vi "BAES RI Retrieval with LABVIEW.vi"() -> ()   [LabVIEW 2013]
uses:
  BaesDataTypeDefinition.ctl
  ReadBaesDataTypeDefinition.ctl
  ParticleDistributionData.ctl
  GeneralDataForRIRetrieval.ctl
  <vilib>/Native 3D Graph/xcontrol/3DPC_SurfacePlot.xctl
  <vilib>/Native 3D Graph/classes/Surface/Surface.lvclass
  RIandRIMCResults.ctl
  <vilib>/gmath/NumericalOptimization/stopping criteria.ctl
  <vilib>/Analysis/1siggen.llb/Ramp Pattern by Samples.vi
  <vilib>/gmath/NumericalOptimization/Conjugate Gradient.vi
  <vilib>/Utility/file.llb/Write To Spreadsheet File (string).vi
  <vilib>/Analysis/Matrix/Numeric/Conversions/Matrix To Array - RM.vi
  <vilib>/gmath/statdist.llb/Normal Inverse CDF.vi
  <vilib>/imath/engines/lvmath2/RunTimeEngine/ErrorHandling/NIMS_Finalize Error.vi
  <vilib>/imath/engines/lvmath2/RunTimeEngine/RangeToken/NIMS_Range_R2 - Float.vi
  <instcachedir>/0/NIMS_Range_R2 - Float_E19924E36A3948A4B33043226480F83C.lvgen/NIMS_Range_R2 - Float_E19924E36A3948A4B33043226480F83C_000.vi
  <vilib>/imath/engines/lvmath2/RunTimeEngine/NodeEndStatement/NIMS_NodeEndStatement_Output.vi
  <instcachedir>/0/NIMS_NodeEndStatement_Output_53EC0D466D134D7ABD903AC30B43404B.lvgen/NIMS_NodeEndStatement_Output_53EC0D466D134D7ABD903AC30B43404B_002.vi
  <vilib>/imath/engines/lvmath2/RunTimeEngine/CommandStatement/MC_CommandStatement_break.vi
  <vilib>/imath/engines/lvmath2/RunTimeSupport/NIMS_Error if Not Equal.vi
  <instcachedir>/0/NIMS_Error if Not Equal_902F5D2649E64F5087A1EF57C55C58AB.lvgen/NIMS_Error if Not Equal_902F5D2649E64F5087A1EF57C55C58AB_000.vi
  <vilib>/imath/engines/lvmath2/RunTimeEngine/IndexRead/NIMS M($,S).vi
  <instcachedir>/0/NIMS M($,S)_3E5749BBB62E49528D4765A77F1F6D98.lvgen/NIMS M($,S)_3E5749BBB62E49528D4765A77F1F6D98_000.vi
  <vilib>/imath/engines/lvmath2/RunTimeEngine/RowToken/NIMS_RowToken_M_CV.vi
  <instcachedir>/0/NIMS_RowToken_M_CV_4FFFB80A1A2C4A06BEF1E2564C6BAFA4.lvgen/NIMS_RowToken_M_CV_4FFFB80A1A2C4A06BEF1E2564C6BAFA4_000.vi
  <vilib>/imath/engines/lvmath2/RunTimeEngine/ErrorHandling/NIMS_Create Error From Enums.vi
  <vilib>/gmath/NI_Gmath.lvlib
  <vilib>/Analysis/Matrix/NI_Matrix.lvlib
  <vilib>/Analysis/NI_AALBase.lvlib
panel:
  out "Size Distribution":T1(graph)=[{"Ramp Pattern"=[105.5, 109.4, 113.4, 117.6, 121.9, 126.3, 131.0, 135.8, 140.7, 145.9, 151.2, 156.8, 162.5, 168.5, 174.7, 181.1, 187.7, 194.6, 201.7, 209.1, 216.7, 224.7, 232.9, 241.4, 250.3, 259.5, 269.0, 278.8, 289.0, 299.6, 310.6, 322.0, 333.8, 346.0, 358.7, 371.8, 385.4, 399.5, 414.2, 429.4, 445.1, 461.4, 478.3, 495.8, 514.0, 532.8, 552.3, 572.5, 593.5, 615.3, 637.8, 661.2, 685.4, 710.5, 736.5, 763.5, 791.5], "Extinction"=[0.0, 0.0, 0.0, 0.0, 0.0, 0.0, 0.00366116, 0.0296415, 0.103002, 0.199671, 0.237311, 0.178682, 0.0821533, 0.0212338, 0.00234049, 0.0, 0.0, 0.0, 0.000322909, 0.00289299, 0.0111396, 0.0241563, 0.0327108, 0.029032, 0.0169297, 0.00614836, 0.00137168, 0.000708524, 0.00196524, 0.0037587, 0.00463248, 0.00371899, 0.00198243, 0.000683679, 0.00013815, 1.21e-05, 0.0, 0.0, 0.0, 0.0, 0.0, 0.0, 0.0, 0.0, 0.0, 0.0, 0.0, 0.0, 0.0, 0.0, 0.0, 0.0, 0.0, 0.0, 0.0, 0.0, 0.0]}, {"Ramp Pattern"=[105.5, 109.4, 113.4, 117.6, 121.9, 126.3, 131.0, 135.8, 140.7, 145.9, 151.2, 156.8, 162.5, 168.5, 174.7, 181.1, 187.7, 194.6, 201.7, 209.1, 216.7, 224.7, 232.9, 241.4, 250.3, 259.5, 269.0, 278.8, 289.0, 299.6, 310.6, 322.0, 333.8, 346.0, 358.7, 371.8, 385.4, 399.5, 414.2, 429.4, 445.1, 461.4, 478.3, 495.8, 514.0, 532.8, 552.3, 572.5, 593.5, 615.3, 637.8, 661.2, 685.4, 710.5, 736.5, 763.5, 791.5], "Extinction"=[0.0, 0.0, 0.0, 0.0, 0.0, 0.0, 0.0, 0.0, 0.0, 0.0, 0.0, 0.0, 0.0, 0.0, 0.00492, 0.0371074, 0.121809, 0.224941, 0.255025, 0.181972, 0.0807483, 0.0201359, 0.00215921, 0.0, 0.0, 0.0, 0.0, 0.000345586, 0.00252918, 0.00805624, 0.0149912, 0.0175018, 0.0135532, 0.00703785, 0.00236058, 0.000456625, 0.000114849, 0.000344556, 0.000807346, 0.00117242, 0.0010019, 0.000622724, 0.000225813, 5.24e-05, 7.42e-06, 4.28e-07, 0.0, 0.0, 0.0, 0.0, 0.0, 0.0, 0.0, 0.0, 0.0, 0.0, 0.0]}, {"Ramp Pattern"=[105.5, 109.4, 113.4, 117.6, 121.9, 126.3, 131.0, 135.8, 140.7, 145.9, 151.2, 156.8, 162.5, 168.5, 174.7, 181.1, 187.7, 194.6, 201.7, 209.1, 216.7, 224.7, 232.9, 241.4, 250.3, 259.5, 269.0, 278.8, 289.0, 299.6, 310.6, 322.0, 333.8, 346.0, 358.7, 371.8, 385.4, 399.5, 414.2, 429.4, 445.1, 461.4, 478.3, 495.8, 514.0, 532.8, 552.3, 572.5, 593.5, 615.3, 637.8, 661.2, 685.4, 710.5, 736.5, 763.5, 791.5], "Extinction"=[0.0, 0.0, 0.0, 0.0, 0.0, 0.0, 0.0, 0.0, 0.0, 0.0, 0.0, 0.0, 0.0, 0.0, 0.0, 0.0, 0.0, 0.0, 0.0, 0.0, 0.00609686, 0.0438534, 0.136127, 0.240173, 0.263478, 0.180795, 0.0780342, 0.019699, 0.00232773, 5.83e-05, 0.0, 0.0, 0.0, 0.0, 0.000288595, 0.00176402, 0.00479166, 0.00737608, 0.00718805, 0.004762, 0.00191333, 0.000545424, 8.17e-05, 1.76e-05, 5.87e-05, 0.000120519, 0.000171987, 0.000138883, 9.46e-05, 3.36e-05, 9.69e-06, 1.71e-06, 1.17e-07, 0.0, 0.0, 0.0, 0.0]}, {"Ramp Pattern"=[105.5, 109.4, 113.4, 117.6, 121.9, 126.3, 131.0, 135.8, 140.7, 145.9, 151.2, 156.8, 162.5, 168.5, 174.7, 181.1, 187.7, 194.6, 201.7, 209.1, 216.7, 224.7, 232.9, 241.4, 250.3, 259.5, 269.0, 278.8, 289.0, 299.6, 310.6, 322.0, 333.8, 346.0, 358.7, 371.8, 385.4, 399.5, 414.2, 429.4, 445.1, 461.4, 478.3, 495.8, 514.0, 532.8, 552.3, 572.5, 593.5, 615.3, 637.8, 661.2, 685.4, 710.5, 736.5, 763.5, 791.5], "Extinction"=[0.0, 0.0, 0.0, 0.0, 0.0, 0.0, 0.0, 0.0, 0.0, 0.0, 0.0, 0.0, 0.0, 0.0, 0.0, 0.0, 0.0, 0.0, 0.0, 0.0, 0.0, 0.0, 0.0, 0.0, 0.0, 0.00736806, 0.0500661, 0.148338, 0.249147, 0.261489, 0.176277, 0.0750088, 0.0194137, 0.00265533, 0.000136312, 0.0, 0.0, 0.0, 0.0, 7.49e-05, 0.000496319, 0.00144105, 0.00238802, 0.00252961, 0.00178475, 0.000847522, 0.000261538, 5.8e-05, 6.72e-06, 5.33e-06, 1.09e-05, 2.51e-05, 4.82e-05, 4.62e-05, 3.31e-05, 2.71e-05, 1.62e-05]}, {"Ramp Pattern"=[105.5, 109.4, 113.4, 117.6, 121.9, 126.3, 131.0, 135.8, 140.7, 145.9, 151.2, 156.8, 162.5, 168.5, 174.7, 181.1, 187.7, 194.6, 201.7, 209.1, 216.7, 224.7, 232.9, 241.4, 250.3, 259.5, 269.0, 278.8, 289.0, 299.6, 310.6, 322.0, 333.8, 346.0, 358.7, 371.8, 385.4, 399.5, 414.2, 429.4, 445.1, 461.4, 478.3, 495.8, 514.0, 532.8, 552.3, 572.5, 593.5, 615.3, 637.8, 661.2, 685.4, 710.5, 736.5, 763.5, 791.5], "Extinction"=[0.0, 0.0, 0.0, 0.0, 0.0, 0.0, 0.0, 0.0, 0.0, 0.0, 0.0, 0.0, 0.0, 0.0, 0.0, 0.0, 0.0, 0.0, 0.0, 0.0, 0.0, 0.0, 0.0, 0.0, 0.0, 0.0, 0.0, 0.0, 0.0, 0.00859775, 0.0562809, 0.158878, 0.25715, 0.258686, 0.166916, 0.0697154, 0.0177192, 0.00255357, 0.000156501, 0.0, 0.0, 0.0, 0.0, 0.0, 5.58e-05, 0.000279561, 0.000610125, 0.000902507, 0.000776539, 0.000511588, 0.000129793, 4.12e-05, 1.04e-05, 1.65e-06, 3.63e-06, 1.15e-05, 1.27e-05]}, {"Ramp Pattern"=[105.5, 109.4, 113.4, 117.6, 121.9, 126.3, 131.0, 135.8, 140.7, 145.9, 151.2, 156.8, 162.5, 168.5, 174.7, 181.1, 187.7, 194.6, 201.7, 209.1, 216.7, 224.7, 232.9, 241.4, 250.3, 259.5, 269.0, 278.8, 289.0, 299.6, 310.6, 322.0, 333.8, 346.0, 358.7, 371.8, 385.4, 399.5, 414.2, 429.4, 445.1, 461.4, 478.3, 495.8, 514.0, 532.8, 552.3, 572.5, 593.5, 615.3, 637.8, 661.2, 685.4, 710.5, 736.5, 763.5, 791.5], "Extinction"=[0.0, 0.0, 0.0, 0.0, 0.0, 0.0, 0.0, 0.0, 0.0, 0.0, 0.0, 0.0, 0.0, 0.0, 0.0, 0.0, 0.0, 0.0, 0.0, 0.0, 0.0, 0.0, 0.0, 0.0, 0.0, 0.0, 0.0, 0.0, 0.0, 0.0, 0.0, 0.0, 0.000337342, 0.0120252, 0.0672961, 0.175789, 0.261716, 0.2491, 0.154041, 0.0606694, 0.0148893, 0.00206533, 0.00012431, 0.0, 0.0, 0.0, 0.0, 0.0, 1.8e-05, 0.000111181, 0.000176009, 0.000314306, 0.00048843, 0.000387935, 0.000231014, 0.000148961, 7.12e-05]}]
  out "Extinction Data per size":T1(graph)=[{"Ramp Pattern"=[350.32001, 350.89999, 351.48999, 352.07001, 352.64001, 353.22, 353.79999, 354.37, 354.94, 355.51001, 356.07999, 356.64999, 357.22, 357.78, 358.35001, 358.91, 359.47, 360.03, 360.59, 361.14999, 361.70001, 362.26001, 362.81, 363.35999, 363.91, 364.45999, 365.01001, 365.56, 366.10001, 366.64999, 367.19, 367.73001, 368.26999, 368.81, 369.35001, 369.89001, 370.42001, 370.95999, 371.48999, 372.03, 372.56, 373.09, 373.62, 374.14999, 374.67999, 375.20999, 375.73001, 376.26001, 376.78, 377.31, 377.82999, 378.35001, 378.87, 379.39001, 379.91, 380.42999, 380.95001, 381.47, 381.98001, 382.5, 383.01001, 383.53, 384.04001, 384.54999, 385.07001, 385.57999, 386.09, 386.60001, 387.10999, 387.62, 388.13, 388.63, 389.14001, 389.64999, 390.14999, 390.66, 391.16, 391.67001, 392.17001, 392.67999, 389.64999, 390.14999, 390.66, 391.16, 391.67001, 392.17001, 392.67999, 393.17999, 393.67999, 394.17999, 394.67999, 395.19, 395.69, 396.19, 396.69, 397.19, 397.69, 398.19, 398.69, 399.19, 399.67999, 400.17999, 400.67999, 401.17999, 401.67999, 402.17001, 402.67001, 403.17001, 403.66, 404.16, 404.66, 405.14999, 405.64999, 406.14999, 406.64001, 407.14001, 407.64001, 408.13, 408.63, 409.13, 409.62, 410.12, 410.62, 411.10999, 411.60999, 412.10001, 412.60001, 413.10001, 413.60001, 414.09, 414.59, 415.09, 415.59, 416.07999, 416.57999, 417.07999, 417.57999, 418.07999, 418.57999, 419.07999, 419.57999, 420.07999, 420.57999, 421.07999, 421.57999, 422.07999, 422.57999, 423.09, 423.59, 424.09, 424.60001], "Extinction"=[3.6031483e-10, 3.5469322e-10, 3.408637e-10, 3.4673833e-10, 3.5910694e-10, 3.5203071e-10, 3.5239295e-10, 3.4944306e-10, 3.493629e-10, 3.5286396e-10, 3.4795894e-10, 3.4986902e-10, 3.4853767e-10, 3.5096345e-10, 3.4530029e-10, 3.4466185e-10, 3.4626552e-10, 3.4120637e-10, 3.4241246e-10, 3.4200121e-10, 3.4181197e-10, 3.3720463e-10, 3.3719594e-10, 3.3340947e-10, 3.3354805e-10, 3.3274e-10, 3.3309006e-10, 3.3158104e-10, 3.2785902e-10, 3.2471797e-10, 3.2142672e-10, 3.2117481e-10, 3.2014302e-10, 3.1719813e-10, 3.166491e-10, 3.1405822e-10, 3.1195083e-10, 3.110861e-10, 3.094415e-10, 3.099751e-10, 3.088679e-10, 3.0802863e-10, 3.071938e-10, 3.0652214e-10, 3.0398342e-10, 3.0334521e-10, 3.0076652e-10, 3.0019606e-10, 3.0035269e-10, 2.9731254e-10, 2.96869e-10, 2.9696506e-10, 2.9196398e-10, 2.9276614e-10, 2.9044214e-10, 2.9082409e-10, 2.8741481e-10, 2.9179151e-10, 2.8504288e-10, 2.8709229e-10, 2.8394356e-10, 2.8090996e-10, 2.8518576e-10, 2.8868899e-10, 2.8050293e-10, 2.7950373e-10, 2.7672264e-10, 2.8093736e-10, 2.7299504e-10, 2.720929e-10, 2.7319211e-10, 2.6788952e-10, 2.7177685e-10, 2.6777444e-10, 2.6549007e-10, 2.6517588e-10, 2.5819685e-10, 2.5802396e-10, 2.6200589e-10, 2.5678593e-10, 2.4595365e-10, 2.5029506e-10, 2.4660043e-10, 2.5315519e-10, 2.4632907e-10, 2.4791411e-10, 2.5175051e-10, 2.5503766e-10, 2.5349259e-10, 2.5248667e-10, 2.501967e-10, 2.5600969e-10, 2.5403385e-10, 2.5142943e-10, 2.4527874e-10, 2.5058799e-10, 2.4682448e-10, 2.5107827e-10, 2.5126284e-10, 2.474817e-10, 2.450305e-10, 2.4602284e-10, 2.4861557e-10, 2.450293e-10, 2.4555724e-10, 2.4487221e-10, 2.4607943e-10, 2.4489663e-10, 2.4417793e-10, 2.4483943e-10, 2.4053959e-10, 2.4118174e-10, 2.3976635e-10, 2.3970775e-10, 2.3782495e-10, 2.3706551e-10, 2.3564872e-10, 2.3965774e-10, 2.3784502e-10, 2.348195e-10, 2.346271e-10, 2.3122344e-10, 2.3139682e-10, 2.3208811e-10, 2.324928e-10, 2.2936233e-10, 2.2667579e-10, 2.2877959e-10, 2.2661809e-10, 2.2463069e-10, 2.2015421e-10, 2.2428925e-10, 2.2008011e-10, 2.200797e-10, 2.2119345e-10, 2.1855351e-10, 2.1575526e-10, 2.0835728e-10, 2.106471e-10, 2.1428238e-10, 2.0796455e-10, 2.0401462e-10, 2.1009262e-10, 2.1211491e-10, 2.0801062e-10, 1.9972174e-10, 2.0241465e-10, 1.9137965e-10, 2.0742474e-10, 1.8590617e-10, 1.9720794e-10]}, {"Ramp Pattern"=[350.32001, 350.32001, 350.32001, 350.89999, 350.89999, 350.89999, 351.48999, 351.48999, 351.48999, 352.07001, 352.07001, 352.07001, 352.64001, 352.64001, 352.64001, 353.22, 353.22, 353.22, 353.79999, 353.79999, 353.79999, 354.37, 354.37, 354.37, 354.94, 354.94, 354.94, 355.51001, 355.51001, 355.51001, 356.07999, 356.07999, 356.07999, 356.64999, 356.64999, 356.64999, 357.22, 357.22, 357.22, 357.78, 357.78, 357.78, 358.35001, 358.35001, 358.35001, 358.91, 358.91, 358.91, 359.47, 359.47, 359.47, 360.03, 360.03, 360.03, 360.59, 360.59, 360.59, 361.14999, 361.14999, 361.14999, 361.70001, 361.70001, 361.70001, 362.26001, 362.26001, 362.26001, 362.81, 362.81, 362.81, 363.35999, 363.35999, 363.35999, 363.91, 363.91, 363.91, 364.45999, 364.45999, 364.45999, 365.01001, 365.01001, 365.01001, 365.56, 365.56, 365.56, 366.10001, 366.10001, 366.10001, 366.64999, 366.64999, 366.64999, 367.19, 367.19, 367.19, 367.73001, 367.73001, 367.73001, 368.26999, 368.26999, 368.26999, 368.81, 368.81, 368.81, 369.35001, 369.35001, 369.35001, 369.89001, 369.89001, 369.89001, 370.42001, 370.42001, 370.42001, 370.95999, 370.95999, 370.95999, 371.48999, 371.48999, 371.48999, 372.03, 372.03, 372.03, 372.56, 372.56, 372.56, 373.09, 373.09, 373.09, 373.62, 373.62, 373.62, 374.14999, 374.14999, 374.14999, 374.67999, 374.67999, 374.67999, 375.20999, 375.20999, 375.20999, 375.73001, 375.73001, 375.73001, 376.26001, 376.26001, 376.26001, 376.78, 376.78, 376.78, 377.31, 377.31, 377.31, 377.82999, 377.82999, 377.82999, 378.35001, 378.35001, 378.35001, 378.87, 378.87, 378.87, 379.39001, 379.39001, 379.39001, 379.91, 379.91, 379.91, 380.42999, 380.42999, 380.42999, 380.95001, 380.95001, 380.95001, 381.47, 381.47, 381.47, 381.98001, 381.98001, 381.98001, 382.5, 382.5, 382.5, 383.01001, 383.01001, 383.01001, 383.53, 383.53, 383.53, 384.04001, 384.04001, 384.04001, 384.54999, 384.54999, 384.54999, 385.07001, 385.07001, 385.07001, 385.57999, 385.57999, 385.57999, 386.09, 386.09, 386.09, 386.60001, 386.60001, 386.60001, 387.10999, 387.10999, 387.10999, 387.62, 387.62, 387.62, 388.13, 388.13, 388.13, 388.63, 388.63, 388.63, 389.14001, 389.14001, 389.14001, 389.64999, 389.64999, 389.64999, 390.14999, 390.14999, 390.14999, 390.66, 390.66, 390.66, 391.16, 391.16, 391.16, 391.67001, 391.67001, 391.67001, 392.17001, 392.17001, 392.17001, 392.67999, 392.67999, 392.67999, 389.64999, 389.64999, 389.64999, 390.14999, 390.14999, 390.14999, 390.66, 390.66, 390.66, 391.16, 391.16, 391.16, 391.67001, 391.67001, 391.67001, 392.17001, 392.17001, 392.17001, 392.67999, 392.67999, 392.67999, 393.17999, 393.17999, 393.17999, 393.67999, 393.67999, 393.67999, 394.17999, 394.17999, 394.17999, 394.67999, 394.67999, 394.67999, 395.19, 395.19, 395.19, 395.69, 395.69, 395.69, 396.19, 396.19, 396.19, 396.69, 396.69, 396.69, 397.19, 397.19, 397.19, 397.69, 397.69, 397.69, 398.19, 398.19, 398.19, 398.69, 398.69, 398.69, 399.19, 399.19, 399.19, 399.67999, 399.67999, 399.67999, 400.17999, 400.17999, 400.17999, 400.67999, 400.67999, 400.67999, 401.17999, 401.17999, 401.17999, 401.67999, 401.67999, 401.67999, 402.17001, 402.17001, 402.17001, 402.67001, 402.67001, 402.67001, 403.17001, 403.17001, 403.17001, 403.66, 403.66, 403.66, 404.16, 404.16, 404.16, 404.66, 404.66, 404.66, 405.14999, 405.14999, 405.14999, 405.64999, 405.64999, 405.64999, 406.14999, 406.14999, 406.14999, 406.64001, 406.64001, 406.64001, 407.14001, 407.14001, 407.14001, 407.64001, 407.64001, 407.64001, 408.13, 408.13, 408.13, 408.63, 408.63, 408.63, 409.13, 409.13, 409.13, 409.62, 409.62, 409.62, 410.12, 410.12, 410.12, 410.62, 410.62, 410.62, 411.10999, 411.10999, 411.10999, 411.60999, 411.60999, 411.60999, 412.10001, 412.10001, 412.10001, 412.60001, 412.60001, 412.60001, 413.10001, 413.10001, 413.10001, 413.60001, 413.60001, 413.60001, 414.09, 414.09, 414.09, 414.59, 414.59, 414.59, 415.09, 415.09, 415.09, 415.59, 415.59, 415.59, 416.07999, 416.07999, 416.07999, 416.57999, 416.57999, 416.57999, 417.07999, 417.07999, 417.07999, 417.57999, 417.57999, 417.57999, 418.07999, 418.07999, 418.07999, 418.57999, 418.57999, 418.57999, 419.07999, 419.07999, 419.07999, 419.57999, 419.57999, 419.57999, 420.07999, 420.07999, 420.07999, 420.57999, 420.57999, 420.57999, 421.07999, 421.07999, 421.07999, 421.57999, 421.57999, 421.57999, 422.07999, 422.07999, 422.07999, 422.57999, 422.57999, 422.57999, 423.09, 423.09, 423.09, 423.59, 423.59, 423.59, 424.09, 424.09, 424.09, 424.60001, 424.60001, 424.60001], "Extinction"=[nan, 3.7357246399999996e-10, 3.47057196e-10, nan, 3.611797045e-10, 3.4820673550000004e-10, nan, 3.460333152e-10, 3.356940848e-10, nan, 3.5692603099999997e-10, 3.36550629e-10, nan, 3.66903319e-10, 3.5131056099999996e-10, nan, 3.571584273e-10, 3.4690299269999997e-10, nan, 3.612825804e-10, 3.435033196e-10, nan, 3.5314861060000003e-10, 3.457375094e-10, nan, 3.554364388e-10, 3.432893612e-10, nan, 3.588979332e-10, 3.4682998680000004e-10, nan, 3.546371275e-10, 3.412807525e-10, nan, 3.546063382e-10, 3.4513170179999997e-10, nan, 3.5280543929999996e-10, 3.442699007e-10, nan, 3.533413404e-10, 3.485855596e-10, nan, 3.487292019e-10, 3.4187137809999997e-10, nan, 3.478808699e-10, 3.414428301e-10, nan, 3.495679634e-10, 3.4296307659999997e-10, nan, 3.4375230480000004e-10, 3.386604352e-10, nan, 3.44482695e-10, 3.40342225e-10, nan, 3.444220593e-10, 3.395803607e-10, nan, 3.439163073e-10, 3.3970763270000003e-10, nan, 3.396687709e-10, 3.347404891e-10, nan, 3.386509659e-10, 3.357409141e-10, nan, 3.360008012e-10, 3.308181388e-10, nan, 3.358736546e-10, 3.312224454e-10, nan, 3.350119146e-10, 3.304680854e-10, nan, 3.3535446179999997e-10, 3.308256582e-10, nan, 3.3310472089999996e-10, 3.300573591e-10, nan, 3.2985239140000003e-10, 3.258656486e-10, nan, 3.265653824e-10, 3.228705576e-10, nan, 3.236659915e-10, 3.191874485e-10, nan, 3.234753625e-10, 3.188742575e-10, nan, 3.215786086e-10, 3.187074314e-10, nan, 3.192160928e-10, 3.151801672e-10, nan, 3.190595757e-10, 3.1423862430000003e-10, nan, 3.1628065709999996e-10, 3.118357829e-10, nan, 3.142807117e-10, 3.096209483e-10, nan, 3.133735016e-10, 3.087986984e-10, nan, 3.1179670109999996e-10, 3.070862989e-10, nan, 3.1277273539999997e-10, 3.071774646e-10, nan, 3.111672851e-10, 3.0656851489999997e-10, nan, 3.1042584240000004e-10, 3.056314176e-10, nan, 3.1053022920000003e-10, 3.038573708e-10, nan, 3.086601583e-10, 3.043841217e-10, nan, 3.062210144e-10, 3.017458256e-10, nan, 3.053000185e-10, 3.013904015e-10, nan, 3.037117359e-10, 2.9782130409999997e-10, nan, 3.026835177e-10, 2.9770860229999996e-10, nan, 3.025671699e-10, 2.981382101e-10, nan, 3.006446094e-10, 2.9398047060000003e-10, nan, 2.998528254e-10, 2.9388517460000003e-10, nan, 3.0030125809999996e-10, 2.936288619e-10, nan, 2.942132147e-10, 2.8971474529999997e-10, nan, 2.955178106e-10, 2.9001446939999996e-10, nan, 2.949105049e-10, 2.859737751e-10, nan, 2.938521242e-10, 2.877960558e-10, nan, 2.915295541e-10, 2.8330006590000003e-10, nan, 2.9364942289999996e-10, 2.899335971e-10, nan, 2.8797354719999997e-10, 2.821122128e-10, nan, 2.911359621e-10, 2.830486179e-10, nan, 2.871950353e-10, 2.8069208469999997e-10, nan, 2.842249953e-10, 2.775949247e-10, nan, 2.897911438e-10, 2.805803762e-10, nan, 2.913717672e-10, 2.860062128e-10, nan, 2.845407231e-10, 2.7646513689999997e-10, nan, 2.8275284669999997e-10, 2.762546133e-10, nan, 2.814956432e-10, 2.7194963679999997e-10, nan, 2.873712226e-10, 2.7450349739999997e-10, nan, 2.784144974e-10, 2.675755826e-10, nan, 2.7726002579999996e-10, 2.669257742e-10, nan, 2.795155613e-10, 2.668686587e-10, nan, 2.713324675e-10, 2.6444657250000004e-10, nan, 2.767898778e-10, 2.667638222e-10, nan, 2.7177316279999996e-10, 2.637757172e-10, nan, 2.6815014789999997e-10, 2.628299921e-10, nan, 2.730826585e-10, 2.572691015e-10, nan, 2.6436251349999997e-10, 2.520311865e-10, nan, 2.67955506e-10, 2.4809241400000003e-10, nan, 2.72526023e-10, 2.51485757e-10, nan, 2.69673682e-10, 2.4389817800000003e-10, nan, 2.5855748999999997e-10, 2.3334981e-10, nan, 2.62096477e-10, 2.3849364300000004e-10, nan, 2.57483807e-10, 2.35717053e-10, nan, 2.613657256e-10, 2.4494465440000003e-10, nan, 2.5075890450000003e-10, 2.418992355e-10, nan, 2.542791691e-10, 2.415490509e-10, nan, 2.5525458829999996e-10, 2.482464317e-10, nan, 2.609401976e-10, 2.491351224e-10, nan, 2.5839575079999997e-10, 2.485894292e-10, nan, 2.5728630509999996e-10, 2.476870349e-10, nan, 2.544552172e-10, 2.459381828e-10, nan, 2.620428236e-10, 2.499765564e-10, nan, 2.6098389899999997e-10, 2.47083801e-10, nan, 2.560743681e-10, 2.4678449190000005e-10, nan, 2.4962326859999997e-10, 2.409342114e-10, nan, 2.549615744e-10, 2.462144056e-10, nan, 2.508877041e-10, 2.4276125589999996e-10, nan, 2.543044231e-10, 2.4785211690000004e-10, nan, 2.544857008e-10, 2.480399792e-10, nan, 2.518423238e-10, 2.431210762e-10, nan, 2.4976100809999997e-10, 2.402999919e-10, nan, 2.488735545e-10, 2.431721255e-10, nan, 2.532837213e-10, 2.4394741869999996e-10, nan, 2.471098866e-10, 2.4294871340000004e-10, nan, 2.491831438e-10, 2.419313362e-10, nan, 2.4917066350000003e-10, 2.405737565e-10, nan, 2.500401307e-10, 2.4211872929999997e-10, nan, 2.480934699e-10, 2.416997901e-10, nan, 2.4687098060000003e-10, 2.414848794e-10, nan, 2.475274434e-10, 2.421514166e-10, nan, 2.435932305e-10, 2.374859495e-10, nan, 2.439275295e-10, 2.384359505e-10, nan, 2.434947023e-10, 2.3603799770000004e-10, nan, 2.432596674e-10, 2.361558326e-10, nan, 2.405329433e-10, 2.351169567e-10, nan, 2.4038961179999997e-10, 2.337414082e-10, nan, 2.385667333e-10, 2.327307067e-10, nan, 2.425947214e-10, 2.367207586e-10, nan, 2.413914316e-10, 2.342986084e-10, nan, 2.371332746e-10, 2.3250572540000003e-10, nan, 2.386091625e-10, 2.306450375e-10, nan, 2.344445661e-10, 2.280023139e-10, nan, 2.362935818e-10, 2.265000582e-10, nan, 2.3381514970000003e-10, 2.303610703e-10, nan, 2.355048984e-10, 2.294807016e-10, nan, 2.325831818e-10, 2.2614147820000001e-10, nan, 2.31238013e-10, 2.22113567e-10, nan, 2.3017824149999998e-10, 2.273809385e-10, nan, 2.303406583e-10, 2.228955217e-10, nan, 2.296121575e-10, 2.196492225e-10, nan, 2.213793912e-10, 2.189290288e-10, nan, 2.274153637e-10, 2.211631363e-10, nan, 2.224827695e-10, 2.176774505e-10, nan, 2.244833706e-10, 2.1567602940000001e-10, nan, 2.252119244e-10, 2.171749756e-10, nan, 2.237101742e-10, 2.1339684580000002e-10, nan, 2.230860236e-10, 2.084244964e-10, nan, 2.134441645e-10, 2.0327039549999999e-10, nan, 2.1511980949999999e-10, 2.061743905e-10, nan, 2.229584347e-10, 2.0560632530000002e-10, nan, 2.143742708e-10, 2.015548292e-10, nan, 2.1595248e-10, 1.9207676000000001e-10, nan, 2.2051368200000002e-10, 1.99671558e-10, nan, 2.23149221e-10, 2.01080599e-10, nan, 2.151061911e-10, 2.009150489e-10, nan, 2.083253995e-10, 1.911180805e-10, nan, 2.06863828e-10, 1.97965472e-10, nan, 1.988425119e-10, 1.8391678810000001e-10, nan, 2.152217166e-10, 1.9962776339999998e-10, nan, 1.9240108010000002e-10, 1.794112599e-10, nan, 2.1755240700000001e-10, 1.76863473e-10]}, {"Ramp Pattern"=[350.32001, 350.89999, 351.48999, 352.07001, 352.64001, 353.22, 353.79999, 354.37, 354.94, 355.51001, 356.07999, 356.64999, 357.22, 357.78, 358.35001, 358.91, 359.47, 360.03, 360.59, 361.14999, 361.70001, 362.26001, 362.81, 363.35999, 363.91, 364.45999, 365.01001, 365.56, 366.10001, 366.64999, 367.19, 367.73001, 368.26999, 368.81, 369.35001, 369.89001, 370.42001, 370.95999, 371.48999, 372.03, 372.56, 373.09, 373.62, 374.14999, 374.67999, 375.20999, 375.73001, 376.26001, 376.78, 377.31, 377.82999, 378.35001, 378.87, 379.39001, 379.91, 380.42999, 380.95001, 381.47, 381.98001, 382.5, 383.01001, 383.53, 384.04001, 384.54999, 385.07001, 385.57999, 386.09, 386.60001, 387.10999, 387.62, 388.13, 388.63, 389.14001, 389.64999, 390.14999, 390.66, 391.16, 391.67001, 392.17001, 392.67999, 389.64999, 390.14999, 390.66, 391.16, 391.67001, 392.17001, 392.67999, 393.17999, 393.67999, 394.17999, 394.67999, 395.19, 395.69, 396.19, 396.69, 397.19, 397.69, 398.19, 398.69, 399.19, 399.67999, 400.17999, 400.67999, 401.17999, 401.67999, 402.17001, 402.67001, 403.17001, 403.66, 404.16, 404.66, 405.14999, 405.64999, 406.14999, 406.64001, 407.14001, 407.64001, 408.13, 408.63, 409.13, 409.62, 410.12, 410.62, 411.10999, 411.60999, 412.10001, 412.60001, 413.10001, 413.60001, 414.09, 414.59, 415.09, 415.59, 416.07999, 416.57999, 417.07999, 417.57999, 418.07999, 418.57999, 419.07999, 419.57999, 420.07999, 420.57999, 421.07999, 421.57999, 422.07999, 422.57999, 423.09, 423.59, 424.09, 424.60001], "Extinction"=[8.6188351e-10, 8.5375762e-10, 8.3701029e-10, 8.405508e-10, 8.4759394e-10, 8.425069e-10, 8.5118895e-10, 8.4900309e-10, 8.5163598e-10, 8.5219604e-10, 8.4385615e-10, 8.454788e-10, 8.4285379e-10, 8.4870405e-10, 8.4042162e-10, 8.3830898e-10, 8.3843837e-10, 8.3187179e-10, 8.3101676e-10, 8.3085511e-10, 8.2594287e-10, 8.2098861e-10, 8.1772827e-10, 8.0942825e-10, 8.1061979e-10, 8.0654622e-10, 8.0405049e-10, 7.9797779e-10, 7.9032164e-10, 7.8061213e-10, 7.7135631e-10, 7.6664514e-10, 7.615068e-10, 7.5434514e-10, 7.5137241e-10, 7.4639356e-10, 7.3874012e-10, 7.3859185e-10, 7.3796669e-10, 7.3793333e-10, 7.3737022e-10, 7.3464668e-10, 7.3152939e-10, 7.2850703e-10, 7.2570666e-10, 7.2356021e-10, 7.1694006e-10, 7.1616524e-10, 7.1679107e-10, 7.1252398e-10, 7.1199663e-10, 7.0437617e-10, 6.9805273e-10, 7.0041534e-10, 6.9733275e-10, 6.9385686e-10, 6.9427603e-10, 6.893473e-10, 6.8755057e-10, 6.8600159e-10, 6.8316441e-10, 6.7775269e-10, 6.859785e-10, 6.8539219e-10, 6.7673761e-10, 6.7310091e-10, 6.6937972e-10, 6.7443784e-10, 6.6113431e-10, 6.5686584e-10, 6.5843608e-10, 6.4766359e-10, 6.4207201e-10, 6.4009492e-10, 6.3714722e-10, 6.3121103e-10, 6.2613853e-10, 6.0922761e-10, 6.0888056e-10, 6.0960798e-10, 5.9956151e-10, 6.1041266e-10, 6.2627464e-10, 6.2038352e-10, 6.0793703e-10, 6.0937488e-10, 6.2101285e-10, 6.1976541e-10, 6.2583327e-10, 6.1622307e-10, 6.1643368e-10, 6.1373145e-10, 6.1815736e-10, 6.1268868e-10, 6.1207384e-10, 6.156628e-10, 6.096168e-10, 6.1431243e-10, 6.1562594e-10, 6.1070826e-10, 6.1028776e-10, 6.0787936e-10, 6.1183425e-10, 6.0589955e-10, 6.0511174e-10, 6.0429189e-10, 5.9970662e-10, 6.0359145e-10, 6.0024885e-10, 5.9936373e-10, 5.9146121e-10, 5.9577365e-10, 5.8999733e-10, 5.9331562e-10, 5.8554422e-10, 5.7981214e-10, 5.8095651e-10, 5.8204769e-10, 5.7982857e-10, 5.7476485e-10, 5.6982158e-10, 5.7281113e-10, 5.7053068e-10, 5.6508048e-10, 5.6397831e-10, 5.6201027e-10, 5.5479082e-10, 5.5355104e-10, 5.4746363e-10, 5.5054628e-10, 5.4731625e-10, 5.4695287e-10, 5.4355409e-10, 5.4195931e-10, 5.3488858e-10, 5.3292099e-10, 5.2904964e-10, 5.2232596e-10, 5.1543331e-10, 5.1405197e-10, 5.0648696e-10, 5.0454541e-10, 5.1921417e-10, 5.1247828e-10, 5.1160692e-10, 5.0328786e-10, 4.9137666e-10, 4.7446586e-10, 4.8615734e-10, 4.7988896e-10, 4.8073928e-10]}, {"Ramp Pattern"=[350.32001, 350.32001, 350.32001, 350.89999, 350.89999, 350.89999, 351.48999, 351.48999, 351.48999, 352.07001, 352.07001, 352.07001, 352.64001, 352.64001, 352.64001, 353.22, 353.22, 353.22, 353.79999, 353.79999, 353.79999, 354.37, 354.37, 354.37, 354.94, 354.94, 354.94, 355.51001, 355.51001, 355.51001, 356.07999, 356.07999, 356.07999, 356.64999, 356.64999, 356.64999, 357.22, 357.22, 357.22, 357.78, 357.78, 357.78, 358.35001, 358.35001, 358.35001, 358.91, 358.91, 358.91, 359.47, 359.47, 359.47, 360.03, 360.03, 360.03, 360.59, 360.59, 360.59, 361.14999, 361.14999, 361.14999, 361.70001, 361.70001, 361.70001, 362.26001, 362.26001, 362.26001, 362.81, 362.81, 362.81, 363.35999, 363.35999, 363.35999, 363.91, 363.91, 363.91, 364.45999, 364.45999, 364.45999, 365.01001, 365.01001, 365.01001, 365.56, 365.56, 365.56, 366.10001, 366.10001, 366.10001, 366.64999, 366.64999, 366.64999, 367.19, 367.19, 367.19, 367.73001, 367.73001, 367.73001, 368.26999, 368.26999, 368.26999, 368.81, 368.81, 368.81, 369.35001, 369.35001, 369.35001, 369.89001, 369.89001, 369.89001, 370.42001, 370.42001, 370.42001, 370.95999, 370.95999, 370.95999, 371.48999, 371.48999, 371.48999, 372.03, 372.03, 372.03, 372.56, 372.56, 372.56, 373.09, 373.09, 373.09, 373.62, 373.62, 373.62, 374.14999, 374.14999, 374.14999, 374.67999, 374.67999, 374.67999, 375.20999, 375.20999, 375.20999, 375.73001, 375.73001, 375.73001, 376.26001, 376.26001, 376.26001, 376.78, 376.78, 376.78, 377.31, 377.31, 377.31, 377.82999, 377.82999, 377.82999, 378.35001, 378.35001, 378.35001, 378.87, 378.87, 378.87, 379.39001, 379.39001, 379.39001, 379.91, 379.91, 379.91, 380.42999, 380.42999, 380.42999, 380.95001, 380.95001, 380.95001, 381.47, 381.47, 381.47, 381.98001, 381.98001, 381.98001, 382.5, 382.5, 382.5, 383.01001, 383.01001, 383.01001, 383.53, 383.53, 383.53, 384.04001, 384.04001, 384.04001, 384.54999, 384.54999, 384.54999, 385.07001, 385.07001, 385.07001, 385.57999, 385.57999, 385.57999, 386.09, 386.09, 386.09, 386.60001, 386.60001, 386.60001, 387.10999, 387.10999, 387.10999, 387.62, 387.62, 387.62, 388.13, 388.13, 388.13, 388.63, 388.63, 388.63, 389.14001, 389.14001, 389.14001, 389.64999, 389.64999, 389.64999, 390.14999, 390.14999, 390.14999, 390.66, 390.66, 390.66, 391.16, 391.16, 391.16, 391.67001, 391.67001, 391.67001, 392.17001, 392.17001, 392.17001, 392.67999, 392.67999, 392.67999, 389.64999, 389.64999, 389.64999, 390.14999, 390.14999, 390.14999, 390.66, 390.66, 390.66, 391.16, 391.16, 391.16, 391.67001, 391.67001, 391.67001, 392.17001, 392.17001, 392.17001, 392.67999, 392.67999, 392.67999, 393.17999, 393.17999, 393.17999, 393.67999, 393.67999, 393.67999, 394.17999, 394.17999, 394.17999, 394.67999, 394.67999, 394.67999, 395.19, 395.19, 395.19, 395.69, 395.69, 395.69, 396.19, 396.19, 396.19, 396.69, 396.69, 396.69, 397.19, 397.19, 397.19, 397.69, 397.69, 397.69, 398.19, 398.19, 398.19, 398.69, 398.69, 398.69, 399.19, 399.19, 399.19, 399.67999, 399.67999, 399.67999, 400.17999, 400.17999, 400.17999, 400.67999, 400.67999, 400.67999, 401.17999, 401.17999, 401.17999, 401.67999, 401.67999, 401.67999, 402.17001, 402.17001, 402.17001, 402.67001, 402.67001, 402.67001, 403.17001, 403.17001, 403.17001, 403.66, 403.66, 403.66, 404.16, 404.16, 404.16, 404.66, 404.66, 404.66, 405.14999, 405.14999, 405.14999, 405.64999, 405.64999, 405.64999, 406.14999, 406.14999, 406.14999, 406.64001, 406.64001, 406.64001, 407.14001, 407.14001, 407.14001, 407.64001, 407.64001, 407.64001, 408.13, 408.13, 408.13, 408.63, 408.63, 408.63, 409.13, 409.13, 409.13, 409.62, 409.62, 409.62, 410.12, 410.12, 410.12, 410.62, 410.62, 410.62, 411.10999, 411.10999, 411.10999, 411.60999, 411.60999, 411.60999, 412.10001, 412.10001, 412.10001, 412.60001, 412.60001, 412.60001, 413.10001, 413.10001, 413.10001, 413.60001, 413.60001, 413.60001, 414.09, 414.09, 414.09, 414.59, 414.59, 414.59, 415.09, 415.09, 415.09, 415.59, 415.59, 415.59, 416.07999, 416.07999, 416.07999, 416.57999, 416.57999, 416.57999, 417.07999, 417.07999, 417.07999, 417.57999, 417.57999, 417.57999, 418.07999, 418.07999, 418.07999, 418.57999, 418.57999, 418.57999, 419.07999, 419.07999, 419.07999, 419.57999, 419.57999, 419.57999, 420.07999, 420.07999, 420.07999, 420.57999, 420.57999, 420.57999, 421.07999, 421.07999, 421.07999, 421.57999, 421.57999, 421.57999, 422.07999, 422.07999, 422.07999, 422.57999, 422.57999, 422.57999, 423.09, 423.09, 423.09, 423.59, 423.59, 423.59, 424.09, 424.09, 424.09, 424.60001, 424.60001, 424.60001], "Extinction"=[nan, 8.67621006e-10, 8.561460140000001e-10, nan, 8.595138961e-10, 8.480013439e-10, nan, 8.444521696e-10, 8.295684104e-10, nan, 8.504097366e-10, 8.306918634e-10, nan, 8.535281671000001e-10, 8.416597129e-10, nan, 8.474807959e-10, 8.375330040999999e-10, nan, 8.575972883000001e-10, 8.447806117e-10, nan, 8.528993375e-10, 8.451068424999999e-10, nan, 8.560060477e-10, 8.472659123000001e-10, nan, 8.560297584999999e-10, 8.483623215e-10, nan, 8.498799942000001e-10, 8.378323058e-10, nan, 8.484340829e-10, 8.425235171e-10, nan, 8.456156762e-10, 8.400919037999999e-10, nan, 8.50961417e-10, 8.46446683e-10, nan, 8.436407559e-10, 8.372024841e-10, nan, 8.408139534e-10, 8.358040066e-10, nan, 8.404637982000001e-10, 8.364129418e-10, nan, 8.336055267e-10, 8.301380532999999e-10, nan, 8.336424294e-10, 8.283910906000001e-10, nan, 8.334866111e-10, 8.282236089e-10, nan, 8.282481961e-10, 8.236375439e-10, nan, 8.22803843e-10, 8.19173377e-10, nan, 8.19734798e-10, 8.157217419999999e-10, nan, 8.11604425e-10, 8.07252075e-10, nan, 8.129024348000001e-10, 8.083371452e-10, nan, 8.085615127e-10, 8.045309273e-10, nan, 8.066140271e-10, 8.014869529e-10, nan, 8.003117822e-10, 7.956437978000001e-10, nan, 7.93140629e-10, 7.87502651e-10, nan, 7.830493679000001e-10, 7.781748921e-10, nan, 7.738794293e-10, 7.688331907e-10, nan, 7.695510573e-10, 7.637392227e-10, nan, 7.643132313e-10, 7.587003687e-10, nan, 7.573774869e-10, 7.513127931000001e-10, nan, 7.550176187e-10, 7.477272013e-10, nan, 7.498331708e-10, 7.429539491999999e-10, nan, 7.423344679e-10, 7.351457721e-10, nan, 7.41896212e-10, 7.35287488e-10, nan, 7.418571604000001e-10, 7.340762196e-10, nan, 7.420926002e-10, 7.337740598e-10, nan, 7.412363817e-10, 7.335040582999999e-10, nan, 7.390708359e-10, 7.302225241000001e-10, nan, 7.359794584e-10, 7.270793216000001e-10, nan, 7.33063175e-10, 7.23950885e-10, nan, 7.291781242e-10, 7.222351958e-10, nan, 7.269656723000001e-10, 7.201547477e-10, nan, 7.210692318e-10, 7.128108882e-10, nan, 7.196632095e-10, 7.126672705e-10, nan, 7.214903391999999e-10, 7.120918008e-10, nan, 7.170612515999999e-10, 7.079867084e-10, nan, 7.156355586e-10, 7.083577014e-10, nan, 7.084840251e-10, 7.002683149e-10, nan, 7.016623747000001e-10, 6.944430853e-10, nan, 7.038731496e-10, 6.969575303999999e-10, nan, 7.023469938e-10, 6.923185061999999e-10, nan, 6.970039981e-10, 6.907097219e-10, nan, 6.994512431e-10, 6.891008169e-10, nan, 6.951437627e-10, 6.835508373e-10, nan, 6.902380795e-10, 6.848630605e-10, nan, 6.911030469999999e-10, 6.80900133e-10, nan, 6.876785374000001e-10, 6.786502826e-10, nan, 6.814977064e-10, 6.740076735999999e-10, nan, 6.893606711e-10, 6.825963289e-10, nan, 6.890246832e-10, 6.817596967999999e-10, nan, 6.828508293e-10, 6.706243907e-10, nan, 6.775242723e-10, 6.686775477e-10, nan, 6.751503011000001e-10, 6.636091389e-10, nan, 6.816836008e-10, 6.671920792e-10, nan, 6.655549462000001e-10, 6.567136738e-10, nan, 6.644629426e-10, 6.492687374e-10, nan, 6.644497911999999e-10, 6.524223688e-10, nan, 6.52986193e-10, 6.42340987e-10, nan, 6.490808371e-10, 6.350631829e-10, nan, 6.449972876e-10, 6.351925524e-10, nan, 6.407721196e-10, 6.335223204e-10, nan, 6.375934644999999e-10, 6.248285955e-10, nan, 6.323641919000001e-10, 6.199128681e-10, nan, 6.157469333e-10, 6.027082867e-10, nan, 6.19371488e-10, 5.983896319999999e-10, nan, 6.190064004e-10, 6.002095596e-10, nan, 6.053290964999999e-10, 5.937939235e-10, nan, 6.185120345000001e-10, 6.023132855e-10, nan, 6.355838974e-10, 6.169653826000001e-10, nan, 6.253522594e-10, 6.154147806e-10, nan, 6.135416574e-10, 6.023324026e-10, nan, 6.16595022e-10, 6.02154738e-10, nan, 6.270037687e-10, 6.150219313e-10, nan, 6.277772729e-10, 6.117535471000001e-10, nan, 6.305012842e-10, 6.211652558e-10, nan, 6.215217074e-10, 6.109244326e-10, nan, 6.249738815e-10, 6.078934784999999e-10, nan, 6.199811993999999e-10, 6.074817006e-10, nan, 6.237864175e-10, 6.125283025e-10, nan, 6.185901191e-10, 6.067872408999999e-10, nan, 6.163611497e-10, 6.077865303e-10, nan, 6.182809940999999e-10, 6.130446059e-10, nan, 6.14525874e-10, 6.04707726e-10, nan, 6.197029362e-10, 6.089219238e-10, nan, 6.217857826e-10, 6.094660974e-10, nan, 6.175906261999999e-10, 6.038258938e-10, nan, 6.142632839e-10, 6.063122361000001e-10, nan, 6.111489109e-10, 6.046098091e-10, nan, 6.157452786e-10, 6.079232214e-10, nan, 6.094992595000001e-10, 6.022998405e-10, nan, 6.094062214e-10, 6.008172586e-10, nan, 6.086996285000001e-10, 5.998841515e-10, nan, 6.053972698000001e-10, 5.940159702e-10, nan, 6.093043988e-10, 5.978785012000001e-10, nan, 6.030072405000001e-10, 5.974904595e-10, nan, 6.023525669999999e-10, 5.96374893e-10, nan, 5.949095842e-10, 5.880128357999999e-10, nan, 6.012870791e-10, 5.902602209e-10, nan, 5.940761346e-10, 5.859185254000001e-10, nan, 5.974529585e-10, 5.891782815e-10, nan, 5.897613063e-10, 5.813271337e-10, nan, 5.852088417e-10, 5.744154383e-10, nan, 5.854095447e-10, 5.765034753e-10, nan, 5.863220248000001e-10, 5.777733552e-10, nan, 5.847120841999999e-10, 5.749450558e-10, nan, 5.789439492999999e-10, 5.705857507e-10, nan, 5.745901622e-10, 5.650529978e-10, nan, 5.763431161e-10, 5.692791439e-10, nan, 5.762962117e-10, 5.647651483e-10, nan, 5.704217213e-10, 5.597392387000001e-10, nan, 5.685083755999999e-10, 5.594482444e-10, nan, 5.661100894e-10, 5.579104505999999e-10, nan, 5.590891061e-10, 5.504925339000001e-10, nan, 5.580024172e-10, 5.490996628e-10, nan, 5.537190181000001e-10, 5.412082419e-10, nan, 5.537292541e-10, 5.473633059e-10, nan, 5.503389872e-10, 5.442935128e-10, nan, 5.496522812e-10, 5.442534588000001e-10, nan, 5.485693217e-10, 5.385388583e-10, nan, 5.477796473e-10, 5.361389727e-10, nan, 5.421077471e-10, 5.276694129e-10, nan, 5.384708973000001e-10, 5.273710827e-10, nan, 5.343063574e-10, 5.237929226e-10, nan, 5.31148297e-10, 5.13503623e-10, nan, 5.204702188e-10, 5.103964012e-10, nan, 5.181617953e-10, 5.099421446999999e-10, nan, 5.136710696e-10, 4.993028503999999e-10, nan, 5.140257033e-10, 4.950651167e-10, nan, 5.282282069e-10, 5.102001331e-10, nan, 5.185561986e-10, 5.064003614e-10, nan, 5.177331103e-10, 5.054807296999999e-10, nan, 5.14768532e-10, 4.91807188e-10, nan, 4.936311183e-10, 4.891222017e-10, nan, 4.799721680999999e-10, 4.689595519e-10, nan, 4.922572219000001e-10, 4.800574581e-10, nan, 4.96835812e-10, 4.62942108e-10, nan, 5.00217928e-10, 4.61260632e-10]}, {"Ramp Pattern"=[350.32001, 350.89999, 351.48999, 352.07001, 352.64001, 353.22, 353.79999, 354.37, 354.94, 355.51001, 356.07999, 356.64999, 357.22, 357.78, 358.35001, 358.91, 359.47, 360.03, 360.59, 361.14999, 361.70001, 362.26001, 362.81, 363.35999, 363.91, 364.45999, 365.01001, 365.56, 366.10001, 366.64999, 367.19, 367.73001, 368.26999, 368.81, 369.35001, 369.89001, 370.42001, 370.95999, 371.48999, 372.03, 372.56, 373.09, 373.62, 374.14999, 374.67999, 375.20999, 375.73001, 376.26001, 376.78, 377.31, 377.82999, 378.35001, 378.87, 379.39001, 379.91, 380.42999, 380.95001, 381.47, 381.98001, 382.5, 383.01001, 383.53, 384.04001, 384.54999, 385.07001, 385.57999, 386.09, 386.60001, 387.10999, 387.62, 388.13, 388.63, 389.14001, 389.64999, 390.14999, 390.66, 391.16, 391.67001, 392.17001, 392.67999, 389.64999, 390.14999, 390.66, 391.16, 391.67001, 392.17001, 392.67999, 393.17999, 393.67999, 394.17999, 394.67999, 395.19, 395.69, 396.19, 396.69, 397.19, 397.69, 398.19, 398.69, 399.19, 399.67999, 400.17999, 400.67999, 401.17999, 401.67999, 402.17001, 402.67001, 403.17001, 403.66, 404.16, 404.66, 405.14999, 405.64999, 406.14999, 406.64001, 407.14001, 407.64001, 408.13, 408.63, 409.13, 409.62, 410.12, 410.62, 411.10999, 411.60999, 412.10001, 412.60001, 413.10001, 413.60001, 414.09, 414.59, 415.09, 415.59, 416.07999, 416.57999, 417.07999, 417.57999, 418.07999, 418.57999, 419.07999, 419.57999, 420.07999, 420.57999, 421.07999, 421.57999, 422.07999, 422.57999, 423.09, 423.59, 424.09, 424.60001], "Extinction"=[1.6042444e-09, 1.6193433e-09, 1.607113e-09, 1.6134795e-09, 1.5807594e-09, 1.566866e-09, 1.590775e-09, 1.5640784e-09, 1.5754599e-09, 1.5819691e-09, 1.5575061e-09, 1.5780176e-09, 1.5567401e-09, 1.5462417e-09, 1.5405127e-09, 1.5478201e-09, 1.535495e-09, 1.5271079e-09, 1.5251926e-09, 1.5253228e-09, 1.5133768e-09, 1.516078e-09, 1.5150128e-09, 1.4988693e-09, 1.4973418e-09, 1.4976772e-09, 1.493291e-09, 1.488961e-09, 1.480441e-09, 1.4782531e-09, 1.4693284e-09, 1.4685163e-09, 1.4619217e-09, 1.4496809e-09, 1.4480611e-09, 1.4436951e-09, 1.4379518e-09, 1.4346799e-09, 1.4352233e-09, 1.4302546e-09, 1.4279919e-09, 1.427039e-09, 1.4235819e-09, 1.4244379e-09, 1.4198029e-09, 1.4138236e-09, 1.413819e-09, 1.4099226e-09, 1.4018124e-09, 1.4024498e-09, 1.4042442e-09, 1.4017647e-09, 1.3910322e-09, 1.3930013e-09, 1.3894086e-09, 1.38554e-09, 1.384027e-09, 1.375292e-09, 1.3852907e-09, 1.3769809e-09, 1.3757454e-09, 1.386908e-09, 1.376557e-09, 1.3837755e-09, 1.3738084e-09, 1.379403e-09, 1.3696372e-09, 1.3581176e-09, 1.3710086e-09, 1.3627306e-09, 1.3558902e-09, 1.339493e-09, 1.3503464e-09, 1.3414119e-09, 1.332737e-09, 1.3475286e-09, 1.3471819e-09, 1.3413515e-09, 1.3037036e-09, 1.3505032e-09, 1.317102e-09, 1.3257242e-09, 1.3175273e-09, 1.33094e-09, 1.3134843e-09, 1.3320818e-09, 1.3220177e-09, 1.2950032e-09, 1.3120133e-09, 1.3101115e-09, 1.304379e-09, 1.3040179e-09, 1.3026366e-09, 1.2923907e-09, 1.2850443e-09, 1.2891297e-09, 1.2866137e-09, 1.2864294e-09, 1.2758068e-09, 1.2776398e-09, 1.2847561e-09, 1.2772065e-09, 1.2805823e-09, 1.2777885e-09, 1.275908e-09, 1.2663115e-09, 1.2797776e-09, 1.2728698e-09, 1.268134e-09, 1.2669639e-09, 1.261699e-09, 1.2627666e-09, 1.2579354e-09, 1.2516999e-09, 1.2484116e-09, 1.2449271e-09, 1.252131e-09, 1.2448163e-09, 1.2371809e-09, 1.2396761e-09, 1.2407702e-09, 1.2405125e-09, 1.2292343e-09, 1.2229795e-09, 1.2224624e-09, 1.228458e-09, 1.2202899e-09, 1.2203069e-09, 1.1996554e-09, 1.2139013e-09, 1.2188386e-09, 1.2051193e-09, 1.1992796e-09, 1.1997117e-09, 1.1963343e-09, 1.1817739e-09, 1.1957139e-09, 1.1627628e-09, 1.1618078e-09, 1.182384e-09, 1.1596676e-09, 1.1607032e-09, 1.1761888e-09, 1.1516913e-09, 1.1730256e-09, 1.1319983e-09, 1.1242637e-09, 1.1504181e-09, 1.1687754e-09, 1.1205662e-09, 1.1325998e-09]}, {"Ramp Pattern"=[350.32001, 350.32001, 350.32001, 350.89999, 350.89999, 350.89999, 351.48999, 351.48999, 351.48999, 352.07001, 352.07001, 352.07001, 352.64001, 352.64001, 352.64001, 353.22, 353.22, 353.22, 353.79999, 353.79999, 353.79999, 354.37, 354.37, 354.37, 354.94, 354.94, 354.94, 355.51001, 355.51001, 355.51001, 356.07999, 356.07999, 356.07999, 356.64999, 356.64999, 356.64999, 357.22, 357.22, 357.22, 357.78, 357.78, 357.78, 358.35001, 358.35001, 358.35001, 358.91, 358.91, 358.91, 359.47, 359.47, 359.47, 360.03, 360.03, 360.03, 360.59, 360.59, 360.59, 361.14999, 361.14999, 361.14999, 361.70001, 361.70001, 361.70001, 362.26001, 362.26001, 362.26001, 362.81, 362.81, 362.81, 363.35999, 363.35999, 363.35999, 363.91, 363.91, 363.91, 364.45999, 364.45999, 364.45999, 365.01001, 365.01001, 365.01001, 365.56, 365.56, 365.56, 366.10001, 366.10001, 366.10001, 366.64999, 366.64999, 366.64999, 367.19, 367.19, 367.19, 367.73001, 367.73001, 367.73001, 368.26999, 368.26999, 368.26999, 368.81, 368.81, 368.81, 369.35001, 369.35001, 369.35001, 369.89001, 369.89001, 369.89001, 370.42001, 370.42001, 370.42001, 370.95999, 370.95999, 370.95999, 371.48999, 371.48999, 371.48999, 372.03, 372.03, 372.03, 372.56, 372.56, 372.56, 373.09, 373.09, 373.09, 373.62, 373.62, 373.62, 374.14999, 374.14999, 374.14999, 374.67999, 374.67999, 374.67999, 375.20999, 375.20999, 375.20999, 375.73001, 375.73001, 375.73001, 376.26001, 376.26001, 376.26001, 376.78, 376.78, 376.78, 377.31, 377.31, 377.31, 377.82999, 377.82999, 377.82999, 378.35001, 378.35001, 378.35001, 378.87, 378.87, 378.87, 379.39001, 379.39001, 379.39001, 379.91, 379.91, 379.91, 380.42999, 380.42999, 380.42999, 380.95001, 380.95001, 380.95001, 381.47, 381.47, 381.47, 381.98001, 381.98001, 381.98001, 382.5, 382.5, 382.5, 383.01001, 383.01001, 383.01001, 383.53, 383.53, 383.53, 384.04001, 384.04001, 384.04001, 384.54999, 384.54999, 384.54999, 385.07001, 385.07001, 385.07001, 385.57999, 385.57999, 385.57999, 386.09, 386.09, 386.09, 386.60001, 386.60001, 386.60001, 387.10999, 387.10999, 387.10999, 387.62, 387.62, 387.62, 388.13, 388.13, 388.13, 388.63, 388.63, 388.63, 389.14001, 389.14001, 389.14001, 389.64999, 389.64999, 389.64999, 390.14999, 390.14999, 390.14999, 390.66, 390.66, 390.66, 391.16, 391.16, 391.16, 391.67001, 391.67001, 391.67001, 392.17001, 392.17001, 392.17001, 392.67999, 392.67999, 392.67999, 389.64999, 389.64999, 389.64999, 390.14999, 390.14999, 390.14999, 390.66, 390.66, 390.66, 391.16, 391.16, 391.16, 391.67001, 391.67001, 391.67001, 392.17001, 392.17001, 392.17001, 392.67999, 392.67999, 392.67999, 393.17999, 393.17999, 393.17999, 393.67999, 393.67999, 393.67999, 394.17999, 394.17999, 394.17999, 394.67999, 394.67999, 394.67999, 395.19, 395.19, 395.19, 395.69, 395.69, 395.69, 396.19, 396.19, 396.19, 396.69, 396.69, 396.69, 397.19, 397.19, 397.19, 397.69, 397.69, 397.69, 398.19, 398.19, 398.19, 398.69, 398.69, 398.69, 399.19, 399.19, 399.19, 399.67999, 399.67999, 399.67999, 400.17999, 400.17999, 400.17999, 400.67999, 400.67999, 400.67999, 401.17999, 401.17999, 401.17999, 401.67999, 401.67999, 401.67999, 402.17001, 402.17001, 402.17001, 402.67001, 402.67001, 402.67001, 403.17001, 403.17001, 403.17001, 403.66, 403.66, 403.66, 404.16, 404.16, 404.16, 404.66, 404.66, 404.66, 405.14999, 405.14999, 405.14999, 405.64999, 405.64999, 405.64999, 406.14999, 406.14999, 406.14999, 406.64001, 406.64001, 406.64001, 407.14001, 407.14001, 407.14001, 407.64001, 407.64001, 407.64001, 408.13, 408.13, 408.13, 408.63, 408.63, 408.63, 409.13, 409.13, 409.13, 409.62, 409.62, 409.62, 410.12, 410.12, 410.12, 410.62, 410.62, 410.62, 411.10999, 411.10999, 411.10999, 411.60999, 411.60999, 411.60999, 412.10001, 412.10001, 412.10001, 412.60001, 412.60001, 412.60001, 413.10001, 413.10001, 413.10001, 413.60001, 413.60001, 413.60001, 414.09, 414.09, 414.09, 414.59, 414.59, 414.59, 415.09, 415.09, 415.09, 415.59, 415.59, 415.59, 416.07999, 416.07999, 416.07999, 416.57999, 416.57999, 416.57999, 417.07999, 417.07999, 417.07999, 417.57999, 417.57999, 417.57999, 418.07999, 418.07999, 418.07999, 418.57999, 418.57999, 418.57999, 419.07999, 419.07999, 419.07999, 419.57999, 419.57999, 419.57999, 420.07999, 420.07999, 420.07999, 420.57999, 420.57999, 420.57999, 421.07999, 421.07999, 421.07999, 421.57999, 421.57999, 421.57999, 422.07999, 422.07999, 422.07999, 422.57999, 422.57999, 422.57999, 423.09, 423.09, 423.09, 423.59, 423.59, 423.59, 424.09, 424.09, 424.09, 424.60001, 424.60001, 424.60001], "Extinction"=[nan, 1.628401705e-09, 1.580087095e-09, nan, 1.658736525e-09, 1.579950075e-09, nan, 1.630528891e-09, 1.583697109e-09, nan, 1.6272254589999999e-09, 1.599733541e-09, nan, 1.5984802210000001e-09, 1.563038579e-09, nan, 1.58162972e-09, 1.5521022799999999e-09, nan, 1.605907491e-09, 1.575642509e-09, nan, 1.580556571e-09, 1.547600229e-09, nan, 1.5928839e-09, 1.5580359e-09, nan, 1.595474427e-09, 1.568463773e-09, nan, 1.5732366419999998e-09, 1.541775558e-09, nan, 1.590952161e-09, 1.5650830389999999e-09, nan, 1.567766457e-09, 1.545713743e-09, nan, 1.558785622e-09, 1.533697778e-09, nan, 1.553574827e-09, 1.5274505729999998e-09, nan, 1.5559646684e-09, 1.5396755315999999e-09, nan, 1.5437539066e-09, 1.5272360934e-09, nan, 1.538798526e-09, 1.5154172740000001e-09, nan, 1.538418848e-09, 1.511966352e-09, nan, 1.5351482572999999e-09, 1.5154973427e-09, nan, 1.5215967031e-09, 1.5051568969e-09, nan, 1.5237714162e-09, 1.5083845838e-09, nan, 1.525027078e-09, 1.504998522e-09, nan, 1.509405434e-09, 1.488333166e-09, nan, 1.5050786979000001e-09, 1.4896049021e-09, nan, 1.5067267181000001e-09, 1.4886276819e-09, nan, 1.5010468602e-09, 1.4855351398e-09, nan, 1.4959158538e-09, 1.4820061461999998e-09, nan, 1.4887938054e-09, 1.4720881946e-09, nan, 1.4861244919000001e-09, 1.4703817081e-09, nan, 1.4763601641e-09, 1.4622966359e-09, nan, 1.4755234306e-09, 1.4615091694e-09, nan, 1.4690368778e-09, 1.4548065222e-09, nan, 1.4570590814e-09, 1.4423027186e-09, nan, 1.4542004217e-09, 1.4419217783e-09, nan, 1.4513892726e-09, 1.4360009274e-09, nan, 1.4448900521e-09, 1.4310135478999999e-09, nan, 1.4413160821e-09, 1.4280437179e-09, nan, 1.4426472764e-09, 1.4277993235999999e-09, nan, 1.4379362643e-09, 1.4225729356999999e-09, nan, 1.435517454e-09, 1.4204663459999998e-09, nan, 1.4333693408e-09, 1.4207086591999999e-09, nan, 1.4310349841999999e-09, 1.4161288158e-09, nan, 1.4305741946e-09, 1.4183016054000001e-09, nan, 1.4254901606000001e-09, 1.4141156394e-09, nan, 1.4208384041e-09, 1.4068087959000001e-09, nan, 1.4205157525e-09, 1.4071222475000001e-09, nan, 1.416502211e-09, 1.403342989e-09, nan, 1.4112666143e-09, 1.3923581857000002e-09, nan, 1.4115532081e-09, 1.3933463919e-09, nan, 1.4125797909e-09, 1.3959086091e-09, nan, 1.4089264759e-09, 1.3946029241e-09, nan, 1.3974592763e-09, 1.3846051237e-09, nan, 1.4011043009e-09, 1.3848982991000001e-09, nan, 1.3978037466e-09, 1.3810134534e-09, nan, 1.3942633311e-09, 1.3768166689e-09, nan, 1.397102508e-09, 1.3709514919999998e-09, nan, 1.387370169e-09, 1.363213831e-09, nan, 1.3953490480000002e-09, 1.375232352e-09, nan, 1.3838281888e-09, 1.3701336112e-09, nan, 1.3837754912999999e-09, 1.3677153087e-09, nan, 1.3971360299999999e-09, 1.37667997e-09, nan, 1.3904144659999998e-09, 1.362699534e-09, nan, 1.395623825e-09, 1.371927175e-09, nan, 1.3844872449999999e-09, 1.363129555e-09, nan, 1.389408202e-09, 1.3693977979999999e-09, nan, 1.385400487e-09, 1.3538739129999999e-09, nan, 1.369113442e-09, 1.3471217579999999e-09, nan, 1.38585322e-09, 1.35616398e-09, nan, 1.3713080452e-09, 1.3541531548000002e-09, nan, 1.368696274e-09, 1.343084126e-09, nan, 1.3493280633e-09, 1.3296579367e-09, nan, 1.364019246e-09, 1.3366735540000002e-09, nan, 1.353521515e-09, 1.329302285e-09, nan, 1.350878951e-09, 1.314595049e-09, nan, 1.365432853e-09, 1.329624347e-09, nan, 1.369192889e-09, 1.3251709110000002e-09, nan, 1.360199697e-09, 1.322503303e-09, nan, 1.324006344e-09, 1.283400856e-09, nan, 1.383703958e-09, 1.317302442e-09, nan, 1.3370847879999998e-09, 1.297119212e-09, nan, 1.3352040708999998e-09, 1.3162443291e-09, nan, 1.3294987190000002e-09, 1.305555881e-09, nan, 1.3523904749999999e-09, 1.309489525e-09, nan, 1.3302793170000001e-09, 1.296689283e-09, nan, 1.347858643e-09, 1.316304957e-09, nan, 1.334730796e-09, 1.309304604e-09, nan, 1.307162044e-09, 1.2828443559999999e-09, nan, 1.331746859e-09, 1.2922797409999998e-09, nan, 1.324097142e-09, 1.296125858e-09, nan, 1.3174922410000002e-09, 1.291265759e-09, nan, 1.3123341817e-09, 1.2957016182999999e-09, nan, 1.3104734751999999e-09, 1.2947997248e-09, nan, 1.3023693472e-09, 1.2824120528e-09, nan, 1.299928514e-09, 1.270160086e-09, nan, 1.300285662e-09, 1.277973738e-09, nan, 1.2931945751999998e-09, 1.2800328248e-09, nan, 1.2958883692e-09, 1.2769704308000001e-09, nan, 1.286745121e-09, 1.264868479e-09, nan, 1.2869712237000002e-09, 1.2683083763e-09, nan, 1.2929360368e-09, 1.2765761632000001e-09, nan, 1.2863341483e-09, 1.2680788517000002e-09, nan, 1.2888394276e-09, 1.2723251724000001e-09, nan, 1.2856852743999999e-09, 1.2698917256e-09, nan, 1.288159864e-09, 1.263656136e-09, nan, 1.2739039987e-09, 1.2587190013e-09, nan, 1.29190229e-09, 1.26765291e-09, nan, 1.2802641949999999e-09, 1.265475405e-09, nan, 1.277759507e-09, 1.2585084930000002e-09, nan, 1.2754495549e-09, 1.2584782450999998e-09, nan, 1.2688647741e-09, 1.2545332259e-09, nan, 1.2700121478999999e-09, 1.2555210521e-09, nan, 1.2655928138e-09, 1.2502779862000002e-09, nan, 1.2600171245000002e-09, 1.2433826755e-09, nan, 1.2537452844e-09, 1.2430779156e-09, nan, 1.2530569831e-09, 1.2367972169000002e-09, nan, 1.2616217988e-09, 1.2426402012e-09, nan, 1.2520758458e-09, 1.2375567541999999e-09, nan, 1.2448439672e-09, 1.2295178328e-09, nan, 1.2472621273e-09, 1.2320900727e-09, nan, 1.2500232522999999e-09, 1.2315171477e-09, nan, 1.248065506e-09, 1.232959494e-09, nan, 1.2385682312e-09, 1.2199003688e-09, nan, 1.2305889755000001e-09, 1.2153700245e-09, nan, 1.2359189600000001e-09, 1.20900584e-09, nan, 1.237995318e-09, 1.2189206820000002e-09, nan, 1.2284961654999999e-09, 1.2120836345e-09, nan, 1.231422416e-09, 1.209191384e-09, nan, 1.2122312279999999e-09, 1.187079572e-09, nan, 1.228691372e-09, 1.1991112279999998e-09, nan, 1.2256005404e-09, 1.2120766596e-09, nan, 1.2135598443e-09, 1.1966787557000001e-09, nan, 1.209882186e-09, 1.1886770140000002e-09, nan, 1.210207675e-09, 1.1892157249999998e-09, nan, 1.2027634519000001e-09, 1.1899051481e-09, nan, 1.19445196e-09, 1.16909584e-09, nan, 1.209019523e-09, 1.182408277e-09, nan, 1.1738859500000001e-09, 1.15163965e-09, nan, 1.186474409e-09, 1.1371411910000001e-09, nan, 1.192463644e-09, 1.172304356e-09, nan, 1.1692856017000001e-09, 1.1500495983e-09, nan, 1.172510167e-09, 1.1488962329999998e-09, nan, 1.18879739e-09, 1.1635802100000001e-09, nan, 1.168521088e-09, 1.134861512e-09, nan, 1.195075122e-09, 1.1509760780000001e-09, nan, 1.1566526500000002e-09, 1.10734395e-09, nan, 1.1549251799999999e-09, 1.09360222e-09, nan, 1.1729806840000001e-09, 1.127855516e-09, nan, 1.199854137e-09, 1.137696663e-09, nan, 1.13336668e-09, 1.10776572e-09, nan, 1.1477455509999999e-09, 1.117454049e-09]}, {"Ramp Pattern"=[350.32001, 350.89999, 351.48999, 352.07001, 352.64001, 353.22, 353.79999, 354.37, 354.94, 355.51001, 356.07999, 356.64999, 357.22, 357.78, 358.35001, 358.91, 359.47, 360.03, 360.59, 361.14999, 361.70001, 362.26001, 362.81, 363.35999, 363.91, 364.45999, 365.01001, 365.56, 366.10001, 366.64999, 367.19, 367.73001, 368.26999, 368.81, 369.35001, 369.89001, 370.42001, 370.95999, 371.48999, 372.03, 372.56, 373.09, 373.62, 374.14999, 374.67999, 375.20999, 375.73001, 376.26001, 376.78, 377.31, 377.82999, 378.35001, 378.87, 379.39001, 379.91, 380.42999, 380.95001, 381.47, 381.98001, 382.5, 383.01001, 383.53, 384.04001, 384.54999, 385.07001, 385.57999, 386.09, 386.60001, 387.10999, 387.62, 388.13, 388.63, 389.14001, 389.64999, 390.14999, 390.66, 391.16, 391.67001, 392.17001, 392.67999, 389.64999, 390.14999, 390.66, 391.16, 391.67001, 392.17001, 392.67999, 393.17999, 393.67999, 394.17999, 394.67999, 395.19, 395.69, 396.19, 396.69, 397.19, 397.69, 398.19, 398.69, 399.19, 399.67999, 400.17999, 400.67999, 401.17999, 401.67999, 402.17001, 402.67001, 403.17001, 403.66, 404.16, 404.66, 405.14999, 405.64999, 406.14999, 406.64001, 407.14001, 407.64001, 408.13, 408.63, 409.13, 409.62, 410.12, 410.62, 411.10999, 411.60999, 412.10001, 412.60001, 413.10001, 413.60001, 414.09, 414.59, 415.09, 415.59, 416.07999, 416.57999, 417.07999, 417.57999, 418.07999, 418.57999, 419.07999, 419.57999, 420.07999, 420.57999, 421.07999, 421.57999, 422.07999, 422.57999, 423.09, 423.59, 424.09, 424.60001], "Extinction"=[2.772367e-09, 2.7228004e-09, 2.7553348e-09, 2.7445968e-09, 2.7080524e-09, 2.6963629e-09, 2.7228155e-09, 2.7038518e-09, 2.7120022e-09, 2.7041378e-09, 2.681011e-09, 2.7063101e-09, 2.6995763e-09, 2.6839533e-09, 2.6846094e-09, 2.6921303e-09, 2.6684794e-09, 2.6661997e-09, 2.6704619e-09, 2.6729465e-09, 2.6511755e-09, 2.6560254e-09, 2.6534506e-09, 2.6429319e-09, 2.6384424e-09, 2.6388964e-09, 2.6328564e-09, 2.6227853e-09, 2.6148381e-09, 2.6067057e-09, 2.5946323e-09, 2.5875326e-09, 2.5804678e-09, 2.5645457e-09, 2.5595865e-09, 2.5525952e-09, 2.5388394e-09, 2.5458087e-09, 2.5432108e-09, 2.5406579e-09, 2.5337874e-09, 2.5365456e-09, 2.5335596e-09, 2.5324081e-09, 2.5241746e-09, 2.5148934e-09, 2.5135354e-09, 2.5082587e-09, 2.4993363e-09, 2.5058078e-09, 2.5011062e-09, 2.4967493e-09, 2.4744338e-09, 2.4773057e-09, 2.4814943e-09, 2.48579e-09, 2.474674e-09, 2.4616695e-09, 2.4650513e-09, 2.4744553e-09, 2.4559641e-09, 2.4618632e-09, 2.4667153e-09, 2.4588873e-09, 2.4505622e-09, 2.4398825e-09, 2.43972e-09, 2.421207e-09, 2.4187508e-09, 2.4247635e-09, 2.4183975e-09, 2.3746243e-09, 2.3975719e-09, 2.3739155e-09, 2.3682234e-09, 2.3716624e-09, 2.37271e-09, 2.3573938e-09, 2.3243405e-09, 2.3504572e-09, 2.3266755e-09, 2.3583941e-09, 2.3436673e-09, 2.3537712e-09, 2.3249183e-09, 2.3632014e-09, 2.3467379e-09, 2.3109796e-09, 2.3347106e-09, 2.3174391e-09, 2.3162434e-09, 2.3121753e-09, 2.2907389e-09, 2.2822149e-09, 2.2733098e-09, 2.2722575e-09, 2.2669215e-09, 2.2607483e-09, 2.2467708e-09, 2.2294797e-09, 2.2549358e-09, 2.2250621e-09, 2.2528104e-09, 2.2260656e-09, 2.2279372e-09, 2.2082056e-09, 2.2304125e-09, 2.2120181e-09, 2.2075739e-09, 2.2009825e-09, 2.1842652e-09, 2.186693e-09, 2.1678033e-09, 2.1691866e-09, 2.1622639e-09, 2.1585573e-09, 2.1555637e-09, 2.1533959e-09, 2.1358235e-09, 2.1476172e-09, 2.1404227e-09, 2.1248747e-09, 2.1276483e-09, 2.1060507e-09, 2.1012125e-09, 2.0962829e-09, 2.0926265e-09, 2.0892696e-09, 2.0678974e-09, 2.0693607e-09, 2.0709898e-09, 2.0644824e-09, 2.0653022e-09, 2.0376822e-09, 2.0472324e-09, 2.0212887e-09, 2.0346873e-09, 1.9883715e-09, 2.002555e-09, 2.0188162e-09, 1.9756812e-09, 1.9786406e-09, 1.9613791e-09, 1.9421744e-09, 2.0166537e-09, 1.9663078e-09, 1.8936779e-09, 1.9514952e-09, 1.9762367e-09, 1.9853403e-09, 1.8305074e-09]}, {"Ramp Pattern"=[350.32001, 350.32001, 350.32001, 350.89999, 350.89999, 350.89999, 351.48999, 351.48999, 351.48999, 352.07001, 352.07001, 352.07001, 352.64001, 352.64001, 352.64001, 353.22, 353.22, 353.22, 353.79999, 353.79999, 353.79999, 354.37, 354.37, 354.37, 354.94, 354.94, 354.94, 355.51001, 355.51001, 355.51001, 356.07999, 356.07999, 356.07999, 356.64999, 356.64999, 356.64999, 357.22, 357.22, 357.22, 357.78, 357.78, 357.78, 358.35001, 358.35001, 358.35001, 358.91, 358.91, 358.91, 359.47, 359.47, 359.47, 360.03, 360.03, 360.03, 360.59, 360.59, 360.59, 361.14999, 361.14999, 361.14999, 361.70001, 361.70001, 361.70001, 362.26001, 362.26001, 362.26001, 362.81, 362.81, 362.81, 363.35999, 363.35999, 363.35999, 363.91, 363.91, 363.91, 364.45999, 364.45999, 364.45999, 365.01001, 365.01001, 365.01001, 365.56, 365.56, 365.56, 366.10001, 366.10001, 366.10001, 366.64999, 366.64999, 366.64999, 367.19, 367.19, 367.19, 367.73001, 367.73001, 367.73001, 368.26999, 368.26999, 368.26999, 368.81, 368.81, 368.81, 369.35001, 369.35001, 369.35001, 369.89001, 369.89001, 369.89001, 370.42001, 370.42001, 370.42001, 370.95999, 370.95999, 370.95999, 371.48999, 371.48999, 371.48999, 372.03, 372.03, 372.03, 372.56, 372.56, 372.56, 373.09, 373.09, 373.09, 373.62, 373.62, 373.62, 374.14999, 374.14999, 374.14999, 374.67999, 374.67999, 374.67999, 375.20999, 375.20999, 375.20999, 375.73001, 375.73001, 375.73001, 376.26001, 376.26001, 376.26001, 376.78, 376.78, 376.78, 377.31, 377.31, 377.31, 377.82999, 377.82999, 377.82999, 378.35001, 378.35001, 378.35001, 378.87, 378.87, 378.87, 379.39001, 379.39001, 379.39001, 379.91, 379.91, 379.91, 380.42999, 380.42999, 380.42999, 380.95001, 380.95001, 380.95001, 381.47, 381.47, 381.47, 381.98001, 381.98001, 381.98001, 382.5, 382.5, 382.5, 383.01001, 383.01001, 383.01001, 383.53, 383.53, 383.53, 384.04001, 384.04001, 384.04001, 384.54999, 384.54999, 384.54999, 385.07001, 385.07001, 385.07001, 385.57999, 385.57999, 385.57999, 386.09, 386.09, 386.09, 386.60001, 386.60001, 386.60001, 387.10999, 387.10999, 387.10999, 387.62, 387.62, 387.62, 388.13, 388.13, 388.13, 388.63, 388.63, 388.63, 389.14001, 389.14001, 389.14001, 389.64999, 389.64999, 389.64999, 390.14999, 390.14999, 390.14999, 390.66, 390.66, 390.66, 391.16, 391.16, 391.16, 391.67001, 391.67001, 391.67001, 392.17001, 392.17001, 392.17001, 392.67999, 392.67999, 392.67999, 389.64999, 389.64999, 389.64999, 390.14999, 390.14999, 390.14999, 390.66, 390.66, 390.66, 391.16, 391.16, 391.16, 391.67001, 391.67001, 391.67001, 392.17001, 392.17001, 392.17001, 392.67999, 392.67999, 392.67999, 393.17999, 393.17999, 393.17999, 393.67999, 393.67999, 393.67999, 394.17999, 394.17999, 394.17999, 394.67999, 394.67999, 394.67999, 395.19, 395.19, 395.19, 395.69, 395.69, 395.69, 396.19, 396.19, 396.19, 396.69, 396.69, 396.69, 397.19, 397.19, 397.19, 397.69, 397.69, 397.69, 398.19, 398.19, 398.19, 398.69, 398.69, 398.69, 399.19, 399.19, 399.19, 399.67999, 399.67999, 399.67999, 400.17999, 400.17999, 400.17999, 400.67999, 400.67999, 400.67999, 401.17999, 401.17999, 401.17999, 401.67999, 401.67999, 401.67999, 402.17001, 402.17001, 402.17001, 402.67001, 402.67001, 402.67001, 403.17001, 403.17001, 403.17001, 403.66, 403.66, 403.66, 404.16, 404.16, 404.16, 404.66, 404.66, 404.66, 405.14999, 405.14999, 405.14999, 405.64999, 405.64999, 405.64999, 406.14999, 406.14999, 406.14999, 406.64001, 406.64001, 406.64001, 407.14001, 407.14001, 407.14001, 407.64001, 407.64001, 407.64001, 408.13, 408.13, 408.13, 408.63, 408.63, 408.63, 409.13, 409.13, 409.13, 409.62, 409.62, 409.62, 410.12, 410.12, 410.12, 410.62, 410.62, 410.62, 411.10999, 411.10999, 411.10999, 411.60999, 411.60999, 411.60999, 412.10001, 412.10001, 412.10001, 412.60001, 412.60001, 412.60001, 413.10001, 413.10001, 413.10001, 413.60001, 413.60001, 413.60001, 414.09, 414.09, 414.09, 414.59, 414.59, 414.59, 415.09, 415.09, 415.09, 415.59, 415.59, 415.59, 416.07999, 416.07999, 416.07999, 416.57999, 416.57999, 416.57999, 417.07999, 417.07999, 417.07999, 417.57999, 417.57999, 417.57999, 418.07999, 418.07999, 418.07999, 418.57999, 418.57999, 418.57999, 419.07999, 419.07999, 419.07999, 419.57999, 419.57999, 419.57999, 420.07999, 420.07999, 420.07999, 420.57999, 420.57999, 420.57999, 421.07999, 421.07999, 421.07999, 421.57999, 421.57999, 421.57999, 422.07999, 422.07999, 422.07999, 422.57999, 422.57999, 422.57999, 423.09, 423.09, 423.09, 423.59, 423.59, 423.59, 424.09, 424.09, 424.09, 424.60001, 424.60001, 424.60001], "Extinction"=[nan, 2.8087139709999998e-09, 2.736020029e-09, nan, 2.75871081e-09, 2.6868899899999998e-09, nan, 2.7765402510000002e-09, 2.734129349e-09, nan, 2.776797563e-09, 2.712396037e-09, nan, 2.7328686549999998e-09, 2.683236145e-09, nan, 2.71958642e-09, 2.6731393800000003e-09, nan, 2.753880026e-09, 2.691750974e-09, nan, 2.7319257600000002e-09, 2.67577784e-09, nan, 2.740898429e-09, 2.683105971e-09, nan, 2.738533488e-09, 2.669742112e-09, nan, 2.7167032029999997e-09, 2.645318797e-09, nan, 2.741205339e-09, 2.671414861e-09, nan, 2.733064065e-09, 2.666088535e-09, nan, 2.722805648e-09, 2.6451009519999997e-09, nan, 2.718969939e-09, 2.650248861e-09, nan, 2.726463159e-09, 2.657797441e-09, nan, 2.701524172e-09, 2.635434628e-09, nan, 2.7011863910000003e-09, 2.631213009e-09, nan, 2.7054647370000003e-09, 2.635459063e-09, nan, 2.707658521e-09, 2.6382344790000003e-09, nan, 2.68606548e-09, 2.61628552e-09, nan, 2.690436291e-09, 2.6216145090000003e-09, nan, 2.686385557e-09, 2.620515643e-09, nan, 2.679286274e-09, 2.6065775259999997e-09, nan, 2.6715202110000004e-09, 2.605364589e-09, nan, 2.673015625e-09, 2.604777175e-09, nan, 2.6670668750000002e-09, 2.598645925e-09, nan, 2.655425489e-09, 2.590145111e-09, nan, 2.647342762e-09, 2.582333438e-09, nan, 2.639107951e-09, 2.574303449e-09, nan, 2.627262771e-09, 2.562001829e-09, nan, 2.61753177e-09, 2.55753343e-09, nan, 2.609773108e-09, 2.551162492e-09, nan, 2.593950279e-09, 2.535141121e-09, nan, 2.591006231e-09, 2.528166769e-09, nan, 2.5818010670000003e-09, 2.523389333e-09, nan, 2.569336227e-09, 2.508342573e-09, nan, 2.5761214869999998e-09, 2.515495913e-09, nan, 2.5734265850000003e-09, 2.512995015e-09, nan, 2.5679839809999997e-09, 2.513331819e-09, nan, 2.56392456e-09, 2.5036502400000004e-09, nan, 2.5648440430000003e-09, 2.508247157e-09, nan, 2.559890164e-09, 2.507229036e-09, nan, 2.560555482e-09, 2.5042607180000002e-09, nan, 2.5525038430000002e-09, 2.495845357e-09, nan, 2.544511097e-09, 2.4852757030000002e-09, nan, 2.5416769150000003e-09, 2.485393885e-09, nan, 2.535480782e-09, 2.4810366180000003e-09, nan, 2.527534483e-09, 2.4711381169999997e-09, nan, 2.531513446e-09, 2.480102154e-09, nan, 2.530157321e-09, 2.4720550789999997e-09, nan, 2.522824036e-09, 2.470674564e-09, nan, 2.501360197e-09, 2.447507403e-09, nan, 2.504676844e-09, 2.449934556e-09, nan, 2.512241909e-09, 2.450746691e-09, nan, 2.516616199e-09, 2.454963801e-09, nan, 2.505352547e-09, 2.443995453e-09, nan, 2.492153293e-09, 2.4311857070000003e-09, nan, 2.4895924189999998e-09, 2.440510181e-09, nan, 2.5048758199999997e-09, 2.44403478e-09, nan, 2.482064513e-09, 2.4298636869999998e-09, nan, 2.4866608139999996e-09, 2.437065586e-09, nan, 2.4977552100000002e-09, 2.43567539e-09, nan, 2.478814939e-09, 2.438959661e-09, nan, 2.475257756e-09, 2.425866644e-09, nan, 2.470731421e-09, 2.409033579e-09, nan, 2.463185131e-09, 2.416254869e-09, nan, 2.444201247e-09, 2.3982127530000002e-09, nan, 2.447412474e-09, 2.390089126e-09, nan, 2.443293813e-09, 2.406233187e-09, nan, 2.448610128e-09, 2.3881848719999998e-09, nan, 2.398049328e-09, 2.351199272e-09, nan, 2.416015822e-09, 2.3791279779999996e-09, nan, 2.3963233079999996e-09, 2.351507692e-09, nan, 2.398833595e-09, 2.3376132050000003e-09, nan, 2.399855913e-09, 2.343468887e-09, nan, 2.390772612e-09, 2.354647388e-09, nan, 2.3764971529999998e-09, 2.338290447e-09, nan, 2.357468976e-09, 2.291212024e-09, nan, 2.3773779210000003e-09, 2.323536479e-09, nan, 2.349389624e-09, 2.3039613759999997e-09, nan, 2.382537511e-09, 2.3342506889999997e-09, nan, 2.372094382e-09, 2.315240218e-09, nan, 2.3830054750000002e-09, 2.324536925e-09, nan, 2.3561074760000002e-09, 2.293729124e-09, nan, 2.385895344e-09, 2.340507456e-09, nan, 2.382728662e-09, 2.310747138e-09, nan, 2.3358472830000003e-09, 2.286111917e-09, nan, 2.375948412e-09, 2.293472788e-09, nan, 2.347457064e-09, 2.287421136e-09, nan, 2.351326298e-09, 2.281160502e-09, nan, 2.328120854e-09, 2.2962297459999998e-09, nan, 2.312804021e-09, 2.268673779e-09, nan, 2.307581841e-09, 2.256847959e-09, nan, 2.2996850559999997e-09, 2.246934544e-09, nan, 2.293727602e-09, 2.2507873980000004e-09, nan, 2.294540211e-09, 2.239302789e-09, nan, 2.282034405e-09, 2.239462195e-09, nan, 2.27782609e-09, 2.21571551e-09, nan, 2.2559517899999998e-09, 2.20300761e-09, nan, 2.273248013e-09, 2.236623587e-09, nan, 2.259540895e-09, 2.190583305e-09, nan, 2.277559342e-09, 2.228061458e-09, nan, 2.2450422950000003e-09, 2.207088905e-09, nan, 2.252437026e-09, 2.203437374e-09, nan, 2.237038732e-09, 2.179372468e-09, nan, 2.252171546e-09, 2.208653454e-09, nan, 2.231319858e-09, 2.1927163420000004e-09, nan, 2.230091563e-09, 2.185056237e-09, nan, 2.227022507e-09, 2.174942493e-09, nan, 2.2087684410000002e-09, 2.159761959e-09, nan, 2.2045545320000002e-09, 2.168831468e-09, nan, 2.194368e-09, 2.1412386000000003e-09, nan, 2.1895774730000003e-09, 2.148795727e-09, nan, 2.193680943e-09, 2.130846857e-09, nan, 2.187479491e-09, 2.129635109e-09, nan, 2.182145449e-09, 2.1289819509999998e-09, nan, 2.184342243e-09, 2.122449557e-09, nan, 2.1553560440000002e-09, 2.116290956e-09, nan, 2.170575492e-09, 2.124658908e-09, nan, 2.166876369e-09, 2.113969031e-09, nan, 2.145557782e-09, 2.1041916180000002e-09, nan, 2.15090674e-09, 2.1043898600000002e-09, nan, 2.130936712e-09, 2.081164688e-09, nan, 2.124908526e-09, 2.077516474e-09, nan, 2.118136591e-09, 2.0744292089999997e-09, nan, 2.11958119e-09, 2.0656718100000004e-09, nan, 2.109357332e-09, 2.069181868e-09, nan, 2.0979268269999997e-09, 2.037867973e-09, nan, 2.0927021450000004e-09, 2.046019255e-09, nan, 2.096391965e-09, 2.045587635e-09, nan, 2.0825970829999997e-09, 2.046367717e-09, nan, 2.084580453e-09, 2.0460239470000003e-09, nan, 2.056492861e-09, 2.0188715389999998e-09, nan, 2.064994112e-09, 2.029470688e-09, nan, 2.048468955e-09, 1.9941084450000003e-09, nan, 2.058566357e-09, 2.010808243e-09, nan, 2.006146877e-09, 1.970596123e-09, nan, 2.0341655339999997e-09, 1.970944466e-09, nan, 2.037588371e-09, 2.000044029e-09, nan, 1.995429982e-09, 1.955932418e-09, nan, 2.010580245e-09, 1.9467009549999997e-09, nan, 1.984861734e-09, 1.9378964659999997e-09, nan, 1.9611013609999998e-09, 1.923247439e-09, nan, 2.054100628e-09, 1.979206772e-09, nan, 2.006100667e-09, 1.926514933e-09, nan, 1.913555016e-09, 1.8738007840000002e-09, nan, 1.9613192122999997e-09, 1.9416711877e-09, nan, 2.00943537e-09, 1.94303803e-09, nan, 2.0036614400000003e-09, 1.96701916e-09, nan, 1.865503888e-09, 1.795510912e-09]}, {"Ramp Pattern"=[350.32001, 350.89999, 351.48999, 352.07001, 352.64001, 353.22, 353.79999, 354.37, 354.94, 355.51001, 356.07999, 356.64999, 357.22, 357.78, 358.35001, 358.91, 359.47, 360.03, 360.59, 361.14999, 361.70001, 362.26001, 362.81, 363.35999, 363.91, 364.45999, 365.01001, 365.56, 366.10001, 366.64999, 367.19, 367.73001, 368.26999, 368.81, 369.35001, 369.89001, 370.42001, 370.95999, 371.48999, 372.03, 372.56, 373.09, 373.62, 374.14999, 374.67999, 375.20999, 375.73001, 376.26001, 376.78, 377.31, 377.82999, 378.35001, 378.87, 379.39001, 379.91, 380.42999, 380.95001, 381.47, 381.98001, 382.5, 383.01001, 383.53, 384.04001, 384.54999, 385.07001, 385.57999, 386.09, 386.60001, 387.10999, 387.62, 388.13, 388.63, 389.14001, 389.64999, 390.14999, 390.66, 391.16, 391.67001, 392.17001, 392.67999, 389.64999, 390.14999, 390.66, 391.16, 391.67001, 392.17001, 392.67999, 393.17999, 393.67999, 394.17999, 394.67999, 395.19, 395.69, 396.19, 396.69, 397.19, 397.69, 398.19, 398.69, 399.19, 399.67999, 400.17999, 400.67999, 401.17999, 401.67999, 402.17001, 402.67001, 403.17001, 403.66, 404.16, 404.66, 405.14999, 405.64999, 406.14999, 406.64001, 407.14001, 407.64001, 408.13, 408.63, 409.13, 409.62, 410.12, 410.62, 411.10999, 411.60999, 412.10001, 412.60001, 413.10001, 413.60001, 414.09, 414.59, 415.09, 415.59, 416.07999, 416.57999, 417.07999, 417.57999, 418.07999, 418.57999, 419.07999, 419.57999, 420.07999, 420.57999, 421.07999, 421.57999, 422.07999, 422.57999, 423.09, 423.59, 424.09, 424.60001], "Extinction"=[3.7474073e-09, 3.7074486e-09, 3.6598513e-09, 3.6549492e-09, 3.5969301e-09, 3.6299781e-09, 3.651963e-09, 3.6045327e-09, 3.6079004e-09, 3.6398144e-09, 3.6043215e-09, 3.6234278e-09, 3.5779146e-09, 3.5782266e-09, 3.5755705e-09, 3.5890875e-09, 3.5385066e-09, 3.5425163e-09, 3.5297552e-09, 3.5531891e-09, 3.53375e-09, 3.5373493e-09, 3.520743e-09, 3.5107139e-09, 3.4941887e-09, 3.5045247e-09, 3.4933612e-09, 3.4834748e-09, 3.4722214e-09, 3.4675505e-09, 3.4477934e-09, 3.4372998e-09, 3.4275862e-09, 3.4168457e-09, 3.4125107e-09, 3.4006749e-09, 3.3962524e-09, 3.3919685e-09, 3.3795857e-09, 3.3828191e-09, 3.3812189e-09, 3.3785783e-09, 3.3728846e-09, 3.3668262e-09, 3.3390335e-09, 3.3446357e-09, 3.3506398e-09, 3.354641e-09, 3.3375056e-09, 3.3427636e-09, 3.3320953e-09, 3.3111829e-09, 3.3251071e-09, 3.3194745e-09, 3.3225096e-09, 3.3372629e-09, 3.3312213e-09, 3.3045431e-09, 3.2981087e-09, 3.3109069e-09, 3.3083305e-09, 3.300465e-09, 3.3208729e-09, 3.3029757e-09, 3.3287881e-09, 3.2993899e-09, 3.2980294e-09, 3.2588727e-09, 3.299915e-09, 3.2995859e-09, 3.3010643e-09, 3.2732419e-09, 3.2728542e-09, 3.2734144e-09, 3.247697e-09, 3.2917e-09, 3.2790919e-09, 3.2495604e-09, 3.2474754e-09, 3.3088081e-09, 3.2537593e-09, 3.2989182e-09, 3.2555398e-09, 3.2793475e-09, 3.2306242e-09, 3.2161613e-09, 3.2337031e-09, 3.2439356e-09, 3.2693275e-09, 3.238765e-09, 3.2587568e-09, 3.2314214e-09, 3.2456937e-09, 3.251492e-09, 3.2155485e-09, 3.2224214e-09, 3.238054e-09, 3.2333936e-09, 3.2242247e-09, 3.2056175e-09, 3.2117129e-09, 3.2370677e-09, 3.248853e-09, 3.2536456e-09, 3.2312324e-09, 3.227683e-09, 3.2410366e-09, 3.2395302e-09, 3.2429917e-09, 3.2214176e-09, 3.2375387e-09, 3.2434122e-09, 3.2143246e-09, 3.2134606e-09, 3.2222718e-09, 3.207389e-09, 3.2258165e-09, 3.2156064e-09, 3.2161591e-09, 3.2278837e-09, 3.2202092e-09, 3.2140077e-09, 3.2067629e-09, 3.1962242e-09, 3.2102889e-09, 3.215213e-09, 3.200106e-09, 3.2350358e-09, 3.1780696e-09, 3.1962939e-09, 3.1882597e-09, 3.1952168e-09, 3.2247427e-09, 3.1955336e-09, 3.2007321e-09, 3.1840914e-09, 3.1359968e-09, 3.0872773e-09, 3.1342036e-09, 3.1927376e-09, 3.0964638e-09, 3.1321892e-09, 3.1040883e-09, 3.0997929e-09, 3.1517573e-09, 3.1029235e-09, 3.1260168e-09, 3.1430067e-09, 3.2714684e-09, 3.1587717e-09, 3.076986e-09]}, {"Ramp Pattern"=[350.32001, 350.32001, 350.32001, 350.89999, 350.89999, 350.89999, 351.48999, 351.48999, 351.48999, 352.07001, 352.07001, 352.07001, 352.64001, 352.64001, 352.64001, 353.22, 353.22, 353.22, 353.79999, 353.79999, 353.79999, 354.37, 354.37, 354.37, 354.94, 354.94, 354.94, 355.51001, 355.51001, 355.51001, 356.07999, 356.07999, 356.07999, 356.64999, 356.64999, 356.64999, 357.22, 357.22, 357.22, 357.78, 357.78, 357.78, 358.35001, 358.35001, 358.35001, 358.91, 358.91, 358.91, 359.47, 359.47, 359.47, 360.03, 360.03, 360.03, 360.59, 360.59, 360.59, 361.14999, 361.14999, 361.14999, 361.70001, 361.70001, 361.70001, 362.26001, 362.26001, 362.26001, 362.81, 362.81, 362.81, 363.35999, 363.35999, 363.35999, 363.91, 363.91, 363.91, 364.45999, 364.45999, 364.45999, 365.01001, 365.01001, 365.01001, 365.56, 365.56, 365.56, 366.10001, 366.10001, 366.10001, 366.64999, 366.64999, 366.64999, 367.19, 367.19, 367.19, 367.73001, 367.73001, 367.73001, 368.26999, 368.26999, 368.26999, 368.81, 368.81, 368.81, 369.35001, 369.35001, 369.35001, 369.89001, 369.89001, 369.89001, 370.42001, 370.42001, 370.42001, 370.95999, 370.95999, 370.95999, 371.48999, 371.48999, 371.48999, 372.03, 372.03, 372.03, 372.56, 372.56, 372.56, 373.09, 373.09, 373.09, 373.62, 373.62, 373.62, 374.14999, 374.14999, 374.14999, 374.67999, 374.67999, 374.67999, 375.20999, 375.20999, 375.20999, 375.73001, 375.73001, 375.73001, 376.26001, 376.26001, 376.26001, 376.78, 376.78, 376.78, 377.31, 377.31, 377.31, 377.82999, 377.82999, 377.82999, 378.35001, 378.35001, 378.35001, 378.87, 378.87, 378.87, 379.39001, 379.39001, 379.39001, 379.91, 379.91, 379.91, 380.42999, 380.42999, 380.42999, 380.95001, 380.95001, 380.95001, 381.47, 381.47, 381.47, 381.98001, 381.98001, 381.98001, 382.5, 382.5, 382.5, 383.01001, 383.01001, 383.01001, 383.53, 383.53, 383.53, 384.04001, 384.04001, 384.04001, 384.54999, 384.54999, 384.54999, 385.07001, 385.07001, 385.07001, 385.57999, 385.57999, 385.57999, 386.09, 386.09, 386.09, 386.60001, 386.60001, 386.60001, 387.10999, 387.10999, 387.10999, 387.62, 387.62, 387.62, 388.13, 388.13, 388.13, 388.63, 388.63, 388.63, 389.14001, 389.14001, 389.14001, 389.64999, 389.64999, 389.64999, 390.14999, 390.14999, 390.14999, 390.66, 390.66, 390.66, 391.16, 391.16, 391.16, 391.67001, 391.67001, 391.67001, 392.17001, 392.17001, 392.17001, 392.67999, 392.67999, 392.67999, 389.64999, 389.64999, 389.64999, 390.14999, 390.14999, 390.14999, 390.66, 390.66, 390.66, 391.16, 391.16, 391.16, 391.67001, 391.67001, 391.67001, 392.17001, 392.17001, 392.17001, 392.67999, 392.67999, 392.67999, 393.17999, 393.17999, 393.17999, 393.67999, 393.67999, 393.67999, 394.17999, 394.17999, 394.17999, 394.67999, 394.67999, 394.67999, 395.19, 395.19, 395.19, 395.69, 395.69, 395.69, 396.19, 396.19, 396.19, 396.69, 396.69, 396.69, 397.19, 397.19, 397.19, 397.69, 397.69, 397.69, 398.19, 398.19, 398.19, 398.69, 398.69, 398.69, 399.19, 399.19, 399.19, 399.67999, 399.67999, 399.67999, 400.17999, 400.17999, 400.17999, 400.67999, 400.67999, 400.67999, 401.17999, 401.17999, 401.17999, 401.67999, 401.67999, 401.67999, 402.17001, 402.17001, 402.17001, 402.67001, 402.67001, 402.67001, 403.17001, 403.17001, 403.17001, 403.66, 403.66, 403.66, 404.16, 404.16, 404.16, 404.66, 404.66, 404.66, 405.14999, 405.14999, 405.14999, 405.64999, 405.64999, 405.64999, 406.14999, 406.14999, 406.14999, 406.64001, 406.64001, 406.64001, 407.14001, 407.14001, 407.14001, 407.64001, 407.64001, 407.64001, 408.13, 408.13, 408.13, 408.63, 408.63, 408.63, 409.13, 409.13, 409.13, 409.62, 409.62, 409.62, 410.12, 410.12, 410.12, 410.62, 410.62, 410.62, 411.10999, 411.10999, 411.10999, 411.60999, 411.60999, 411.60999, 412.10001, 412.10001, 412.10001, 412.60001, 412.60001, 412.60001, 413.10001, 413.10001, 413.10001, 413.60001, 413.60001, 413.60001, 414.09, 414.09, 414.09, 414.59, 414.59, 414.59, 415.09, 415.09, 415.09, 415.59, 415.59, 415.59, 416.07999, 416.07999, 416.07999, 416.57999, 416.57999, 416.57999, 417.07999, 417.07999, 417.07999, 417.57999, 417.57999, 417.57999, 418.07999, 418.07999, 418.07999, 418.57999, 418.57999, 418.57999, 419.07999, 419.07999, 419.07999, 419.57999, 419.57999, 419.57999, 420.07999, 420.07999, 420.07999, 420.57999, 420.57999, 420.57999, 421.07999, 421.07999, 421.07999, 421.57999, 421.57999, 421.57999, 422.07999, 422.07999, 422.07999, 422.57999, 422.57999, 422.57999, 423.09, 423.09, 423.09, 423.59, 423.59, 423.59, 424.09, 424.09, 424.09, 424.60001, 424.60001, 424.60001], "Extinction"=[nan, 3.799603134e-09, 3.6952114660000005e-09, nan, 3.784085568e-09, 3.630811632e-09, nan, 3.708245328e-09, 3.6114572719999998e-09, nan, 3.697910026e-09, 3.611988374e-09, nan, 3.6307311769999998e-09, 3.563129023e-09, nan, 3.666703986e-09, 3.593252214e-09, nan, 3.69298784e-09, 3.61093816e-09, nan, 3.6367540780000004e-09, 3.572311322e-09, nan, 3.638905213e-09, 3.576895587e-09, nan, 3.6774136259999997e-09, 3.602215174e-09, nan, 3.625947994e-09, 3.5826950059999998e-09, nan, 3.647727484e-09, 3.599128116e-09, nan, 3.609716512e-09, 3.5461126879999998e-09, nan, 3.603699566e-09, 3.552753634e-09, nan, 3.599004614e-09, 3.552136386e-09, nan, 3.612646287e-09, 3.565528713e-09, nan, 3.561348896e-09, 3.515664304e-09, nan, 3.562823781e-09, 3.522208819e-09, nan, 3.551964325e-09, 3.5075460750000004e-09, nan, 3.5812853599999997e-09, 3.52509284e-09, nan, 3.557313155e-09, 3.510186845e-09, nan, 3.558690215e-09, 3.5160083850000003e-09, nan, 3.541645086e-09, 3.499840914e-09, nan, 3.530837666e-09, 3.490590134e-09, nan, 3.514679743e-09, 3.473697657e-09, nan, 3.526016921e-09, 3.4830324790000003e-09, nan, 3.516535229e-09, 3.470187171e-09, nan, 3.504461866e-09, 3.462487734e-09, nan, 3.492240487e-09, 3.452202313e-09, nan, 3.487519681e-09, 3.4475813189999997e-09, nan, 3.467993908e-09, 3.427592892e-09, nan, 3.457887843e-09, 3.4167117570000002e-09, nan, 3.449215733e-09, 3.4059566670000003e-09, nan, 3.437480158e-09, 3.3962112420000002e-09, nan, 3.433978531e-09, 3.391042869e-09, nan, 3.422514987e-09, 3.3788348129999998e-09, nan, 3.418448175e-09, 3.374056625e-09, nan, 3.413253338e-09, 3.3706836620000003e-09, nan, 3.3998652250000003e-09, 3.359306175e-09, nan, 3.405848413e-09, 3.3597897869999997e-09, nan, 3.40245667e-09, 3.35998113e-09, nan, 3.401635226e-09, 3.355521374e-09, nan, 3.3932991949999997e-09, 3.352470005e-09, nan, 3.388728834e-09, 3.3449235660000003e-09, nan, 3.358749187e-09, 3.319317813e-09, nan, 3.368058247e-09, 3.321213153e-09, nan, 3.373278538e-09, 3.3280010619999997e-09, nan, 3.3782871939999998e-09, 3.330994806e-09, nan, 3.3616303129999997e-09, 3.313380887e-09, nan, 3.367998076e-09, 3.3175291240000002e-09, nan, 3.352068448e-09, 3.3121221519999997e-09, nan, 3.336593789e-09, 3.2857720109999997e-09, nan, 3.346607785e-09, 3.3036064149999998e-09, nan, 3.344519447e-09, 3.294429553e-09, nan, 3.347340045e-09, 3.2976791549999998e-09, nan, 3.3712806749999998e-09, 3.303245125e-09, nan, 3.358968799e-09, 3.303473801e-09, nan, 3.330549554e-09, 3.278536646e-09, nan, 3.325700866e-09, 3.270516534e-09, nan, 3.337819083e-09, 3.283994717e-09, nan, 3.330303247e-09, 3.286357753e-09, nan, 3.329102754e-09, 3.271827246e-09, nan, 3.351966611e-09, 3.289779189e-09, nan, 3.332917145e-09, 3.273034255e-09, nan, 3.370514757e-09, 3.287061443e-09, nan, 3.323857824e-09, 3.274921976e-09, nan, 3.3321321759999998e-09, 3.263926624e-09, nan, 3.292277645e-09, 3.225467755e-09, nan, 3.337500018e-09, 3.262329982e-09, nan, 3.321588754e-09, 3.277583046e-09, nan, 3.341285671e-09, 3.260842929e-09, nan, 3.305082961e-09, 3.241400839e-09, nan, 3.30082029e-09, 3.24488811e-09, nan, 3.3065457689999997e-09, 3.240283031e-09, nan, 3.276240074e-09, 3.219153926e-09, nan, 3.351928232e-09, 3.231471768e-09, nan, 3.323976815e-09, 3.234206985e-09, nan, 3.2978474719999997e-09, 3.201273328e-09, nan, 3.3103276029999998e-09, 3.184623197e-09, nan, 3.365160391e-09, 3.252455809e-09, nan, 3.29108547e-09, 3.21643313e-09, nan, 3.35472354e-09, 3.24311286e-09, nan, 3.3154709640000002e-09, 3.195608636e-09, nan, 3.3093050089999998e-09, 3.249389991e-09, nan, 3.261934137e-09, 3.1993142629999998e-09, nan, 3.2419211370000004e-09, 3.190401463e-09, nan, 3.2698936229999998e-09, 3.197512577e-09, nan, 3.2748142050000002e-09, 3.213056995e-09, nan, 3.293756474e-09, 3.244898526e-09, nan, 3.275759241e-09, 3.201770759e-09, nan, 3.291619405e-09, 3.2258941949999997e-09, nan, 3.25922709e-09, 3.20361571e-09, nan, 3.284108877e-09, 3.207278523e-09, nan, 3.276677911e-09, 3.2263060890000002e-09, nan, 3.241880202e-09, 3.189216798e-09, nan, 3.24289615e-09, 3.2019466500000003e-09, nan, 3.273201992e-09, 3.202906008e-09, nan, 3.260335415e-09, 3.2064517850000002e-09, nan, 3.246781139e-09, 3.201668261e-09, nan, 3.230875868e-09, 3.180359132e-09, nan, 3.239757593e-09, 3.183668207e-09, nan, 3.270632021e-09, 3.203503379e-09, nan, 3.2802971530000003e-09, 3.217408847e-09, nan, 3.278924964e-09, 3.228366236e-09, nan, 3.251454514e-09, 3.211010286e-09, nan, 3.261093063e-09, 3.194272937e-09, nan, 3.264935988e-09, 3.217137212e-09, nan, 3.263266279e-09, 3.215794121e-09, nan, 3.26916709e-09, 3.21681631e-09, nan, 3.245136569e-09, 3.197698631e-09, nan, 3.260366912e-09, 3.214710488e-09, nan, 3.265615337e-09, 3.221209063e-09, nan, 3.237369395e-09, 3.191279805e-09, nan, 3.237770815e-09, 3.189150385e-09, nan, 3.247689824e-09, 3.196853776e-09, nan, 3.231488731e-09, 3.183289269e-09, nan, 3.25105048e-09, 3.20058252e-09, nan, 3.2380714799999997e-09, 3.19314132e-09, nan, 3.246822721e-09, 3.1854954789999998e-09, nan, 3.249355203e-09, 3.206412197e-09, nan, 3.246378735e-09, 3.1940396650000003e-09, nan, 3.240324319e-09, 3.1876910809999998e-09, nan, 3.229251676e-09, 3.1842741239999997e-09, nan, 3.228898862e-09, 3.163549538e-09, nan, 3.233204198e-09, 3.187373602e-09, nan, 3.2420609939999997e-09, 3.188365006e-09, nan, 3.232523947e-09, 3.167688053e-09, nan, 3.269178513e-09, 3.200893087e-09, nan, 3.206068431e-09, 3.150070769e-09, nan, 3.219633694e-09, 3.172954106e-09, nan, 3.214493339e-09, 3.1620260609999996e-09, nan, 3.225451167e-09, 3.164982433e-09, nan, 3.250190854e-09, 3.1992945459999996e-09, nan, 3.235913678e-09, 3.155153522e-09, nan, 3.241276373e-09, 3.1601878269999996e-09, nan, 3.211601585e-09, 3.156581215e-09, nan, 3.174687892e-09, 3.097305708e-09, nan, 3.131261734e-09, 3.043292866e-09, nan, 3.181808992e-09, 3.0865982080000003e-09, nan, 3.233700142e-09, 3.151775058e-09, nan, 3.1425407649999998e-09, 3.050386835e-09, nan, 3.180176193e-09, 3.084202207e-09, nan, 3.153028197e-09, 3.055148403e-09, nan, 3.1541028700000003e-09, 3.04548293e-09, nan, 3.19496369e-09, 3.1085509099999997e-09, nan, 3.167224856e-09, 3.038622144e-09, nan, 3.190068779e-09, 3.061964821e-09, nan, 3.226477521e-09, 3.059535879e-09, nan, 3.336822185e-09, 3.2061146149999998e-09, nan, 3.226348748e-09, 3.091194652e-09, nan, 3.171589519e-09, 2.9823824810000002e-09]}, {"Ramp Pattern"=[350.32001, 350.89999, 351.48999, 352.07001, 352.64001, 353.22, 353.79999, 354.37, 354.94, 355.51001, 356.07999, 356.64999, 357.22, 357.78, 358.35001, 358.91, 359.47, 360.03, 360.59, 361.14999, 361.70001, 362.26001, 362.81, 363.35999, 363.91, 364.45999, 365.01001, 365.56, 366.10001, 366.64999, 367.19, 367.73001, 368.26999, 368.81, 369.35001, 369.89001, 370.42001, 370.95999, 371.48999, 372.03, 372.56, 373.09, 373.62, 374.14999, 374.67999, 375.20999, 375.73001, 376.26001, 376.78, 377.31, 377.82999, 378.35001, 378.87, 379.39001, 379.91, 380.42999, 380.95001, 381.47, 381.98001, 382.5, 383.01001, 383.53, 384.04001, 384.54999, 385.07001, 385.57999, 386.09, 386.60001, 387.10999, 387.62, 388.13, 388.63, 389.14001, 389.64999, 390.14999, 390.66, 391.16, 391.67001, 392.17001, 392.67999, 389.64999, 390.14999, 390.66, 391.16, 391.67001, 392.17001, 392.67999, 393.17999, 393.67999, 394.17999, 394.67999, 395.19, 395.69, 396.19, 396.69, 397.19, 397.69, 398.19, 398.69, 399.19, 399.67999, 400.17999, 400.67999, 401.17999, 401.67999, 402.17001, 402.67001, 403.17001, 403.66, 404.16, 404.66, 405.14999, 405.64999, 406.14999, 406.64001, 407.14001, 407.64001, 408.13, 408.63, 409.13, 409.62, 410.12, 410.62, 411.10999, 411.60999, 412.10001, 412.60001, 413.10001, 413.60001, 414.09, 414.59, 415.09, 415.59, 416.07999, 416.57999, 417.07999, 417.57999, 418.07999, 418.57999, 419.07999, 419.57999, 420.07999, 420.57999, 421.07999, 421.57999, 422.07999, 422.57999, 423.09, 423.59, 424.09, 424.60001], "Extinction"=[4.3745572e-09, 4.337859e-09, 4.3808392e-09, 4.2718717e-09, 4.2808499e-09, 4.2863175e-09, 4.3089967e-09, 4.2364467e-09, 4.2719086e-09, 4.3698383e-09, 4.2854689e-09, 4.3801793e-09, 4.2871369e-09, 4.3137476e-09, 4.3153761e-09, 4.3193946e-09, 4.3025539e-09, 4.3145727e-09, 4.2992561e-09, 4.2915933e-09, 4.3011381e-09, 4.3050088e-09, 4.3078563e-09, 4.3033039e-09, 4.2906803e-09, 4.3190056e-09, 4.2985975e-09, 4.2953712e-09, 4.273538e-09, 4.285202e-09, 4.2655972e-09, 4.2557406e-09, 4.2351731e-09, 4.2364405e-09, 4.239824e-09, 4.2367976e-09, 4.242585e-09, 4.2576787e-09, 4.2411732e-09, 4.2629402e-09, 4.2566697e-09, 4.2559081e-09, 4.2717194e-09, 4.2823403e-09, 4.2671848e-09, 4.2666968e-09, 4.2822963e-09, 4.2859845e-09, 4.259193e-09, 4.3025241e-09, 4.3002313e-09, 4.3079904e-09, 4.2648201e-09, 4.275365e-09, 4.3164854e-09, 4.3354316e-09, 4.3161061e-09, 4.3707171e-09, 4.300801e-09, 4.3639781e-09, 4.35656e-09, 4.3658579e-09, 4.3601576e-09, 4.3791446e-09, 4.3526223e-09, 4.3885016e-09, 4.4086303e-09, 4.332867e-09, 4.3520516e-09, 4.4201776e-09, 4.3225445e-09, 4.29515e-09, 4.3346944e-09, 4.4070965e-09, 4.2593467e-09, 4.3264445e-09, 4.344729e-09, 4.3095034e-09, 4.2225561e-09, 4.3461257e-09, 4.2268198e-09, 4.3749777e-09, 4.3380153e-09, 4.3563904e-09, 4.3220387e-09, 4.3807669e-09, 4.3495292e-09, 4.336667e-09, 4.2956527e-09, 4.3645358e-09, 4.3047832e-09, 4.2943773e-09, 4.3470743e-09, 4.3549173e-09, 4.3017003e-09, 4.2789572e-09, 4.2708352e-09, 4.3186028e-09, 4.2920174e-09, 4.2470116e-09, 4.3064237e-09, 4.2893338e-09, 4.3340087e-09, 4.2642037e-09, 4.2642316e-09, 4.2634505e-09, 4.3024331e-09, 4.2846944e-09, 4.2405737e-09, 4.2380535e-09, 4.2506514e-09, 4.2684727e-09, 4.2686574e-09, 4.2304191e-09, 4.2500532e-09, 4.1988755e-09, 4.2486992e-09, 4.1885593e-09, 4.1801038e-09, 4.1874708e-09, 4.1708148e-09, 4.165682e-09, 4.203045e-09, 4.1132915e-09, 4.1717669e-09, 4.1820898e-09, 4.1241646e-09, 4.1477115e-09, 4.1017785e-09, 4.1311292e-09, 4.1095225e-09, 4.1101336e-09, 4.1410555e-09, 4.1347041e-09, 4.1272665e-09, 4.0885055e-09, 4.0175006e-09, 3.9775774e-09, 3.9987973e-09, 4.1108059e-09, 4.0211798e-09, 4.0659596e-09, 3.9198844e-09, 3.8821679e-09, 4.1236388e-09, 4.040702e-09, 3.9411363e-09, 4.1209991e-09, 4.1564316e-09, 3.8459174e-09, 3.8327905e-09]}, {"Ramp Pattern"=[350.32001, 350.32001, 350.32001, 350.89999, 350.89999, 350.89999, 351.48999, 351.48999, 351.48999, 352.07001, 352.07001, 352.07001, 352.64001, 352.64001, 352.64001, 353.22, 353.22, 353.22, 353.79999, 353.79999, 353.79999, 354.37, 354.37, 354.37, 354.94, 354.94, 354.94, 355.51001, 355.51001, 355.51001, 356.07999, 356.07999, 356.07999, 356.64999, 356.64999, 356.64999, 357.22, 357.22, 357.22, 357.78, 357.78, 357.78, 358.35001, 358.35001, 358.35001, 358.91, 358.91, 358.91, 359.47, 359.47, 359.47, 360.03, 360.03, 360.03, 360.59, 360.59, 360.59, 361.14999, 361.14999, 361.14999, 361.70001, 361.70001, 361.70001, 362.26001, 362.26001, 362.26001, 362.81, 362.81, 362.81, 363.35999, 363.35999, 363.35999, 363.91, 363.91, 363.91, 364.45999, 364.45999, 364.45999, 365.01001, 365.01001, 365.01001, 365.56, 365.56, 365.56, 366.10001, 366.10001, 366.10001, 366.64999, 366.64999, 366.64999, 367.19, 367.19, 367.19, 367.73001, 367.73001, 367.73001, 368.26999, 368.26999, 368.26999, 368.81, 368.81, 368.81, 369.35001, 369.35001, 369.35001, 369.89001, 369.89001, 369.89001, 370.42001, 370.42001, 370.42001, 370.95999, 370.95999, 370.95999, 371.48999, 371.48999, 371.48999, 372.03, 372.03, 372.03, 372.56, 372.56, 372.56, 373.09, 373.09, 373.09, 373.62, 373.62, 373.62, 374.14999, 374.14999, 374.14999, 374.67999, 374.67999, 374.67999, 375.20999, 375.20999, 375.20999, 375.73001, 375.73001, 375.73001, 376.26001, 376.26001, 376.26001, 376.78, 376.78, 376.78, 377.31, 377.31, 377.31, 377.82999, 377.82999, 377.82999, 378.35001, 378.35001, 378.35001, 378.87, 378.87, 378.87, 379.39001, 379.39001, 379.39001, 379.91, 379.91, 379.91, 380.42999, 380.42999, 380.42999, 380.95001, 380.95001, 380.95001, 381.47, 381.47, 381.47, 381.98001, 381.98001, 381.98001, 382.5, 382.5, 382.5, 383.01001, 383.01001, 383.01001, 383.53, 383.53, 383.53, 384.04001, 384.04001, 384.04001, 384.54999, 384.54999, 384.54999, 385.07001, 385.07001, 385.07001, 385.57999, 385.57999, 385.57999, 386.09, 386.09, 386.09, 386.60001, 386.60001, 386.60001, 387.10999, 387.10999, 387.10999, 387.62, 387.62, 387.62, 388.13, 388.13, 388.13, 388.63, 388.63, 388.63, 389.14001, 389.14001, 389.14001, 389.64999, 389.64999, 389.64999, 390.14999, 390.14999, 390.14999, 390.66, 390.66, 390.66, 391.16, 391.16, 391.16, 391.67001, 391.67001, 391.67001, 392.17001, 392.17001, 392.17001, 392.67999, 392.67999, 392.67999, 389.64999, 389.64999, 389.64999, 390.14999, 390.14999, 390.14999, 390.66, 390.66, 390.66, 391.16, 391.16, 391.16, 391.67001, 391.67001, 391.67001, 392.17001, 392.17001, 392.17001, 392.67999, 392.67999, 392.67999, 393.17999, 393.17999, 393.17999, 393.67999, 393.67999, 393.67999, 394.17999, 394.17999, 394.17999, 394.67999, 394.67999, 394.67999, 395.19, 395.19, 395.19, 395.69, 395.69, 395.69, 396.19, 396.19, 396.19, 396.69, 396.69, 396.69, 397.19, 397.19, 397.19, 397.69, 397.69, 397.69, 398.19, 398.19, 398.19, 398.69, 398.69, 398.69, 399.19, 399.19, 399.19, 399.67999, 399.67999, 399.67999, 400.17999, 400.17999, 400.17999, 400.67999, 400.67999, 400.67999, 401.17999, 401.17999, 401.17999, 401.67999, 401.67999, 401.67999, 402.17001, 402.17001, 402.17001, 402.67001, 402.67001, 402.67001, 403.17001, 403.17001, 403.17001, 403.66, 403.66, 403.66, 404.16, 404.16, 404.16, 404.66, 404.66, 404.66, 405.14999, 405.14999, 405.14999, 405.64999, 405.64999, 405.64999, 406.14999, 406.14999, 406.14999, 406.64001, 406.64001, 406.64001, 407.14001, 407.14001, 407.14001, 407.64001, 407.64001, 407.64001, 408.13, 408.13, 408.13, 408.63, 408.63, 408.63, 409.13, 409.13, 409.13, 409.62, 409.62, 409.62, 410.12, 410.12, 410.12, 410.62, 410.62, 410.62, 411.10999, 411.10999, 411.10999, 411.60999, 411.60999, 411.60999, 412.10001, 412.10001, 412.10001, 412.60001, 412.60001, 412.60001, 413.10001, 413.10001, 413.10001, 413.60001, 413.60001, 413.60001, 414.09, 414.09, 414.09, 414.59, 414.59, 414.59, 415.09, 415.09, 415.09, 415.59, 415.59, 415.59, 416.07999, 416.07999, 416.07999, 416.57999, 416.57999, 416.57999, 417.07999, 417.07999, 417.07999, 417.57999, 417.57999, 417.57999, 418.07999, 418.07999, 418.07999, 418.57999, 418.57999, 418.57999, 419.07999, 419.07999, 419.07999, 419.57999, 419.57999, 419.57999, 420.07999, 420.07999, 420.07999, 420.57999, 420.57999, 420.57999, 421.07999, 421.07999, 421.07999, 421.57999, 421.57999, 421.57999, 422.07999, 422.07999, 422.07999, 422.57999, 422.57999, 422.57999, 423.09, 423.09, 423.09, 423.59, 423.59, 423.59, 424.09, 424.09, 424.09, 424.60001, 424.60001, 424.60001], "Extinction"=[nan, 4.51505262e-09, 4.234061779999999e-09, nan, 4.51054986e-09, 4.16516814e-09, nan, 4.509363339999999e-09, 4.25231506e-09, nan, 4.366163781e-09, 4.177579619e-09, nan, 4.3253394819999995e-09, 4.236360318e-09, nan, 4.339907955e-09, 4.232727045e-09, nan, 4.3972248119999994e-09, 4.220768588e-09, nan, 4.297852081e-09, 4.175041319e-09, nan, 4.34450965e-09, 4.19930755e-09, nan, 4.451701719e-09, 4.287974881e-09, nan, 4.34323964e-09, 4.2276981599999994e-09, nan, 4.43429784e-09, 4.32606076e-09, nan, 4.357570288e-09, 4.2167035120000006e-09, nan, 4.365039286e-09, 4.2624559140000006e-09, nan, 4.371368051e-09, 4.259384149e-09, nan, 4.371103473e-09, 4.2676857269999995e-09, nan, 4.365652655e-09, 4.2394551449999995e-09, nan, 4.363322527e-09, 4.265822873000001e-09, nan, 4.34865887e-09, 4.24985333e-09, nan, 4.346896357e-09, 4.2362902429999995e-09, nan, 4.352915866e-09, 4.2493603340000005e-09, nan, 4.3460312489999996e-09, 4.263986351e-09, nan, 4.349944553e-09, 4.265768047e-09, nan, 4.348372942e-09, 4.258234858e-09, nan, 4.333825534e-09, 4.247535066e-09, nan, 4.366002191e-09, 4.272009008999999e-09, nan, 4.342833608e-09, 4.254361392e-09, nan, 4.336081097e-09, 4.254661303e-09, nan, 4.318436887e-09, 4.2286391129999996e-09, nan, 4.325340427e-09, 4.245063573e-09, nan, 4.306806396e-09, 4.224388004e-09, nan, 4.297243377e-09, 4.214237823e-09, nan, 4.279686979e-09, 4.1906592210000005e-09, nan, 4.2797227669999995e-09, 4.193158233e-09, nan, 4.278479992000001e-09, 4.201168008e-09, nan, 4.276949745e-09, 4.1966454550000005e-09, nan, 4.282696754e-09, 4.202473246000001e-09, nan, 4.301415367e-09, 4.213942033e-09, nan, 4.281809816e-09, 4.200536584e-09, nan, 4.303931286e-09, 4.221949114e-09, nan, 4.294033708000001e-09, 4.219305692e-09, nan, 4.297600881e-09, 4.214215319e-09, nan, 4.312235987e-09, 4.231202813e-09, nan, 4.320753881e-09, 4.243926719e-09, nan, 4.311747163999999e-09, 4.222622436e-09, nan, 4.315050486e-09, 4.218343114000001e-09, nan, 4.325888319e-09, 4.2387042810000005e-09, nan, 4.325097411e-09, 4.246871589e-09, nan, 4.3006507609999994e-09, 4.217735239e-09, nan, 4.34754618e-09, 4.2575020200000006e-09, nan, 4.338373484e-09, 4.262089116e-09, nan, 4.35805148e-09, 4.2579293199999995e-09, nan, 4.318452351000001e-09, 4.211187849e-09, nan, 4.322386092e-09, 4.228343908e-09, nan, 4.358466628e-09, 4.274504171999999e-09, nan, 4.396485443e-09, 4.274377757e-09, nan, 4.369621507e-09, 4.262590693000001e-09, nan, 4.428605176e-09, 4.312829024e-09, nan, 4.364680055e-09, 4.236921945e-09, nan, 4.42127015e-09, 4.30668605e-09, nan, 4.40553301e-09, 4.3075869900000005e-09, nan, 4.42813457e-09, 4.30358123e-09, nan, 4.401090354e-09, 4.319224846e-09, nan, 4.4441449869999996e-09, 4.314144213e-09, nan, 4.414960483e-09, 4.2902841169999995e-09, nan, 4.432183942000001e-09, 4.344819258e-09, nan, 4.470260258e-09, 4.3470003420000006e-09, nan, 4.3950376509999996e-09, 4.270696349e-09, nan, 4.430181485e-09, 4.2739217149999995e-09, nan, 4.482809416000001e-09, 4.357545784e-09, nan, 4.3852826689999995e-09, 4.259806331e-09, nan, 4.3513305639999995e-09, 4.238969436e-09, nan, 4.413327472e-09, 4.256061328e-09, nan, 4.49041463e-09, 4.3237783700000005e-09, nan, 4.328408456e-09, 4.1902849439999996e-09, nan, 4.4386351400000006e-09, 4.21425386e-09, nan, 4.416409516e-09, 4.2730484839999995e-09, nan, 4.398986529e-09, 4.2200202709999996e-09, nan, 4.274906783e-09, 4.170205417e-09, nan, 4.4905965e-09, 4.2016549e-09, nan, 4.316273446e-09, 4.137366154e-09, nan, 4.468173054e-09, 4.281782345999999e-09, nan, 4.510447989999999e-09, 4.16558261e-09, nan, 4.436460864e-09, 4.2763199359999995e-09, nan, 4.418419838999999e-09, 4.225657561e-09, nan, 4.4444581609999996e-09, 4.317075639e-09, nan, 4.434949308e-09, 4.264109092e-09, nan, 4.418428868e-09, 4.254905132e-09, nan, 4.377726798e-09, 4.2135786020000005e-09, nan, 4.426867752e-09, 4.3022038479999996e-09, nan, 4.3664191879999995e-09, 4.243147212e-09, nan, 4.364418724e-09, 4.2243358759999996e-09, nan, 4.445894294e-09, 4.2482543059999995e-09, nan, 4.421218515e-09, 4.288616085e-09, nan, 4.3781496399999995e-09, 4.22525096e-09, nan, 4.3393608200000005e-09, 4.21855358e-09, nan, 4.336454051e-09, 4.2052163490000004e-09, nan, 4.38052245e-09, 4.2566831499999996e-09, nan, 4.352084476e-09, 4.2319503240000004e-09, nan, 4.312513933e-09, 4.181509267000001e-09, nan, 4.381874936e-09, 4.230972464e-09, nan, 4.360525707e-09, 4.2181418930000005e-09, nan, 4.405650544999999e-09, 4.262366855e-09, nan, 4.328697707e-09, 4.1997096929999994e-09, nan, 4.3201804120000005e-09, 4.208282788e-09, nan, 4.341863366e-09, 4.1850376340000004e-09, nan, 4.35987785e-09, 4.2449883500000005e-09, nan, 4.3393694180000005e-09, 4.230019382e-09, nan, 4.300811855e-09, 4.180335545e-09, nan, 4.289066718e-09, 4.187040282e-09, nan, 4.30298595e-09, 4.19831685e-09, nan, 4.322973191e-09, 4.213972209e-09, nan, 4.336922273e-09, 4.200392527e-09, nan, 4.2866464670000005e-09, 4.174191733e-09, nan, 4.302769711999999e-09, 4.197336688e-09, nan, 4.254532396e-09, 4.143218604e-09, nan, 4.302603172e-09, 4.194795228e-09, nan, 4.240444602e-09, 4.136673997999999e-09, nan, 4.24671868e-09, 4.11348892e-09, nan, 4.2546825500000004e-09, 4.12025905e-09, nan, 4.2307371660000005e-09, 4.110892434e-09, nan, 4.224573038e-09, 4.1067909620000005e-09, nan, 4.2645258e-09, 4.1415642e-09, nan, 4.190008098e-09, 4.036574902e-09, nan, 4.243336095e-09, 4.100197705e-09, nan, 4.240226643e-09, 4.123952957e-09, nan, 4.181738272e-09, 4.066590928e-09, nan, 4.235513009e-09, 4.059909991e-09, nan, 4.158501258e-09, 4.045055742e-09, nan, 4.201614117e-09, 4.060644283e-09, nan, 4.197488419e-09, 4.021556581e-09, nan, 4.1924660739999995e-09, 4.027801126e-09, nan, 4.201697325e-09, 4.080413675e-09, nan, 4.195657571000001e-09, 4.073750629e-09, nan, 4.194904721e-09, 4.0596282790000004e-09, nan, 4.138424732e-09, 4.038586268e-09, nan, 4.0889491479999995e-09, 3.946052052e-09, nan, 4.069659894e-09, 3.885494906e-09, nan, 4.077766326e-09, 3.919828274e-09, nan, 4.193909653e-09, 4.0277021469999995e-09, nan, 4.1260693100000004e-09, 3.91629029e-09, nan, 4.20052013e-09, 3.93139907e-09, nan, 4.014133023e-09, 3.825635777e-09, nan, 3.981864477e-09, 3.782471323e-09, nan, 4.216403374e-09, 4.030874226e-09, nan, 4.1472298499999995e-09, 3.93417415e-09, nan, 4.09645545e-09, 3.7858171499999996e-09, nan, 4.22465504e-09, 4.01734316e-09, nan, 4.29784509e-09, 4.0150181100000005e-09, nan, 3.99360605e-09, 3.6982287500000004e-09, nan, 3.98260741e-09, 3.68297359e-09]}]
  out "Wavelength":string="WL=413.600nm"
  out "Imaginary Part":string="k=0.020±0.000"
  out "Real Part":string="n=1.583±0.000"
  in  "Quick Fit":bool
  in  "Diameters to fit":i32[](listbox)=[5]
  out "Residue":dbl=1.6495086916401946
  in  "ExtinctionOrAbsorptionOrScattering":i8(knob) scale=0.0..2.0
  in  "Plot RI":bool
  in  "k":dbl=0.042
  in  "n":dbl=1.668
  out "Residue (CDMRI)":dbl=39.086698664953175
  out "Wavelength":dbl=413.60001 format="%.3g"
  out "Imaginary Uncertainty":dbl caption="±" format="%.3g"
  out "Imaginary Part":dbl=0.0195021318464305 format="%.3g"
  out "Real Uncertainty":dbl caption="±" format="%.3g"
  out "Real part":dbl=1.5826360995824014 format="%.3g"
  out "Diameter Offset":dbl
  out "Diameter Factor":dbl=1.0
  out "Extinction Factor":dbl=1.0
  out "Residue (MDBF)":dbl=5.222371255351293
  out "Time Left (min)":dbl=22.74556666666667 format="%#.1f"
  out "Progress bar for Extinction search":u8(slide)=12 max=5 scale=-1.0..51.0
  in  "Diameter Factor Radio Button":bool
  in  "Diamter Offset Radio Button":bool=TRUE
  in  "Diameter FO Interval":dbl=1.0 caption="Interval"
  in  "Diameter FO Finish":dbl=5.0 caption="Finish"
  in  "Diameter FO start":dbl=-5.0 caption="Start"
  in  "Diameter Offset":dbl
  in  "Diameter Factor":dbl=1.0
  in  "Extinction Factor":dbl=1.2
  in  "Extinction Factor Interval":dbl=0.1 caption="Interval"
  in  "Extinction Factor Finish":dbl=1.2 caption="Finish"
  in  "Extinction Factor Start":dbl=0.8 caption="Start"
  in  "Find Extinction Factor Graph":bool
  out "3D Graph":refnum<class "Base Datatype.lvclass">[](xcontrol)
  in  "Use Factors":bool
  in  "Min Wavelength":string(combo)="0"
  in  "Max Wavelength":string(combo)="150"
  in  "Restrict to Positive Imaginary Part":bool=TRUE
  in  "Calculate Errors":bool=TRUE
  in  "Approximate Errors":bool
  in  "Save RI":bool
  in  "Retrieve RI":bool
  in  "Mutiple Charge Data File":path=path "SRFA_Multiply charge distribution.txt"
  in  "Extinction Cross Section File":path=path "ext data for lior.txt"
  in  "Diameter Factor or Offset 2":bool=TRUE caption="Offset - True, Factor - OFF"
  out "Simplex":T2(graph)=[{"Size parameters"=[1.5804453509322545, 1.5804416862605781, 1.580446807878156, 1.5804453509322545], "Normalized Residuals"=[0.0019796920484383444, 0.0020030778938541043, 0.0020224415674907938, 0.0019796920484383444]}]
  in  "Diameter Factor or Offset":bool=TRUE caption="Offset - True, Factor - OFF"
  in  "Minimization method":u16(ring)=1 items=["LM method", "Simplex Method"]
  in  "Extinction Factor in Data":dbl=1.0
  out "Residue Graph Matrix":dbl[][](array[numeric])=[[0.8817748876641518, 0.7943260267120898, 0.7221799384952265, 0.6683504995926692, 0.6311277469517097, 0.6088767086158524], [0.7307518731289654, 0.673042958848353, 0.6345421279928648, 0.6122901406297341, 0.6040701363961388, 0.6079500250191767], [0.6456146353159482, 0.6217239264490524, 0.6132715417472164, 0.6175167400813633, 0.6328117960393451, 0.6563665043893292], [0.6273068413741216, 0.6311010869376654, 0.6464620791865137, 0.671082182122829, 0.7034305368703453, 0.741845745993439], [0.6631237737749567, 0.6880232407171314, 0.7208560286150587, 0.7602689432195936, 0.8046376766720158, 0.8530494481747876]]
  out "Extinction Factor Results":cluster{dbl[], dbl[]}[](graph)=[{[0.8, 0.9, 1.0, 1.1, 1.2], [1.539671374334097, 1.5976213646223005, 1.5606320545412844, 1.5516397914476685, 1.5319499648100456]}, {[0.8, 0.9, 1.0, 1.1, 1.2], [-0.11096660801067405, -0.0653657766346238, -0.05966999471633491, -0.017727862931787984, 0.01906205546692944]}, {[0.8, 0.9, 1.0, 1.1, 1.2], [13.260187371616055, 8.444315776530917, 1.2615157523101117, 0.7276563123626676, 0.6329059597830448]}]
  in  "General Data for RI Retrieval VI":T3={"Min WaveLength Index"=0, "Max WaveLength Index"=0, "Extinction Factor"=FALSE, "Size Parameter Factor"=FALSE, "Size Paramter Offset"=FALSE, "Extinction Factor"=1.0, "Diameter Factor"=1.0, "Diameter Offset"=0.0, "ExtinctionOrAbsorptionOrScattering"=0} {"ExtinctionOrAbsorptionOrScattering" scale=0.0..2.0; "Max WaveLength Index" max=200 step=1; "Min WaveLength Index" max=200 step=1}
  in  "Graph Refs 2":T4
  in  "Size Parameter Offset":bool
  in  "Size Parameter Factor":bool
  in  "Extinction Factor":bool
  out "Minimized Size Parameter Factor":dbl
  out "Minimized Extinction Factor":dbl
  in  "Data for RIRetrieval VI":T7={"Approximate Errors"=FALSE, "Extinction ExtinctionUncertainity Size parameter and Number ofS sizes"={"Extinction"=[], "Extinction Uncertainty"=[], "Size parameters"=[], "Number ofSizes"=0.0, "GeometricCrossSection"=[], "WaveLength"=[], "Sizes"=[]}, "Minimization method"=0, "Graph Ref"={"Real Part vs wavelength"=refnum, "Imaginary Part vs wavelength"=refnum, "Normalized Residuals vs Size parameter"=refnum, "Not Corrected for Multiple charge particles"=refnum, "Simplex 2"=refnum}, "Particle Distribution Data"={"SMPS Sizes"=[], "Concentration"=[], "Double Charge Correction Flag"=FALSE}, "Calculate Errors"=FALSE, "Restrict to Positive Imaginary Part"=FALSE, "MinMaxWavelength"={0, 0, "Extinction Factor"=FALSE, "Size Parameter Factor"=FALSE, "Size Parameter Offset"=TRUE, "Extinction Factor"=1.0, "Diameter Factor"=1.0, "Diameter Offset"=0.0, "ExtinctionOrAbsorptionOrScattering"=0}} {"MinMaxWavelength"."ExtinctionOrAbsorptionOrScattering" scale=0.0..2.0}
  in  "Graph Refs":T4
  in  "Factor Ext Uncertainty in Data":dbl=1.0
  in  "Save RI expanded Edition":bool
  out "Saved RI to this filename and path 2":path=path "Z:/Dropbox/Lior Segev/Lior Segev Projects/RI retrieval in Labview/Data/Ammonium Sulfate/20130724ForMatlabRetrival-RIresult.xls"
  out "index of element":i32=128
  out "Corrected for multiple charge particles":cluster{"Size parameters":dbl[], dbl[]}[](graph)=[{"Size parameters"=[1.1393590102632467, 1.5191453470176624, 1.8989316837720778, 2.2787180205264934, 2.658504357280909], [9.401560883343829e-11, 3.7348341970896743e-10, 1.0776478608049149e-09, 2.0097516486454724e-09, 3.1564749317119423e-09]}, {"Size parameters"=[1.1393590102632467, 1.5191453470176624, 1.8989316837720778, 2.2787180205264934, 2.658504357280909], [2.2661809e-10, 5.4746363e-10, 1.1996554e-09, 2.0678974e-09, 3.1780696e-09]}, {"Size parameters"=[0.9114872082105974, 0.9342743884158623, 0.9570615686211272, 0.9798487488263922, 1.002635929031657, 1.0254231092369221, 1.048210289442187, 1.0709974696474518, 1.0937846498527168, 1.1165718300579819, 1.1393590102632467, 1.1621461904685115, 1.1849333706737766, 1.2077205508790416, 1.2305077310843064, 1.2532949112895713, 1.2760820914948363, 1.2988692717001014, 1.3216564519053662, 1.344443632110631, 1.367230812315896, 1.390017992521161, 1.412805172726426, 1.4355923529316907, 1.4583795331369558, 1.4811667133422208, 1.5039538935474857, 1.5267410737527505, 1.5495282539580155, 1.5723154341632806, 1.5951026143685454, 1.6178897945738102, 1.6406769747790753, 1.6634641549843403, 1.6862513351896051, 1.70903851539487, 1.731825695600135, 1.7546128758054, 1.7774000560106649, 1.8001872362159297, 1.8229744164211947, 1.8457615966264598, 1.8685487768317246, 1.8913359570369894, 1.9141231372422545, 1.9369103174475195, 1.9596974976527843, 1.9824846778580492, 2.005271858063314, 2.0280590382685793, 2.0508462184738443, 2.073633398679109, 2.096420578884374, 2.119207759089639, 2.1419949392949036, 2.1647821195001686, 2.1875692997054337, 2.2103564799106987, 2.2331436601159638, 2.2559308403212284, 2.2787180205264934, 2.3015052007317585, 2.324292380937023, 2.347079561142288, 2.369866741347553, 2.392653921552818, 2.4154411017580832, 2.438228281963348, 2.461015462168613, 2.483802642373878, 2.5065898225791425, 2.5293770027844076, 2.5521641829896726, 2.5749513631949377, 2.5977385434002027, 2.6205257236054673, 2.6433129038107324, 2.6661000840159974, 2.688887264221262, 2.711674444426527, 2.734461624631792, 2.757248804837057, 2.780035985042322, 2.802823165247587, 2.825610345452852, 2.848397525658117, 2.8711847058633815, 2.8939718860686465, 2.9167590662739116, 2.9395462464791766, 2.9623334266844417, 2.9851206068897063, 3.0079077870949713, 3.0306949673002364, 3.053482147505501, 3.076269327710766, 3.099056507916031, 3.121843688121296, 3.144630868326561, 3.1674180485318257, 3.190205228737091], [2.8627016139019763e-11, 3.2621640096618214e-11, 3.704154269464328e-11, 4.191334345355653e-11, 4.726316052253534e-11, 5.311662717416695e-11, 5.949871590739165e-11, 6.643373170848311e-11, 7.39455997265154e-11, 8.205795408770465e-11, 9.079478993087089e-11, 1.001808265013646e-10, 1.102421605179007e-10, 1.2100776422150365e-10, 1.3251014095638043e-10, 1.4478641906515875e-10, 1.578800421631613e-10, 1.7184266987486228e-10, 1.8673470472876231e-10, 2.0262740501603027e-10, 2.1960362056339615e-10, 2.3775925541856704e-10, 2.5720255494660736e-10, 2.780547333951105e-10, 3.004475518242973e-10, 3.2452049058363325e-10, 3.504168297259522e-10, 3.7827738605854277e-10, 4.0823219274343914e-10, 4.403907047776598e-10, 4.748304519920101e-10, 5.115871434565556e-10, 5.506412361820939e-10, 5.919096452956665e-10, 6.352393422202262e-10, 6.804094898000639e-10, 7.271334267114976e-10, 7.750736937119327e-10, 8.23858550402552e-10, 8.731076787982143e-10, 9.224544572312689e-10, 9.715719005012873e-10, 1.02019399271762e-09, 1.0681283385737478e-09, 1.1152692350656976e-09, 1.1615974828247653e-09, 1.207178466767119e-09, 1.2521523619110985e-09, 1.2967296973115024e-09, 1.341172979748723e-09, 1.3857920865058363e-09, 1.4309315213194903e-09, 1.4769635093934683e-09, 1.5242813475807354e-09, 1.5732951037806631e-09, 1.6244261675808928e-09, 1.6781056690249909e-09, 1.7347680490271024e-09, 1.7948445936541683e-09, 1.8587574988168223e-09, 1.9269024765619817e-09, 1.9996326165294874e-09, 2.077236860001548e-09, 2.1599060705827714e-09, 2.247703085616502e-09, 2.3405288978069358e-09, 2.438087746801078e-09, 2.539863421904488e-09, 2.6451104934935647e-09, 2.7528731610198846e-09, 2.8620228010005904e-09, 2.971311291064927e-09, 3.0794684560556956e-09, 3.1852835638670228e-09, 3.287696777454103e-09, 3.385862671833763e-09, 3.4792024424071533e-09, 3.567418256329342e-09, 3.6504836208046184e-09, 3.7286098001593054e-09, 3.802214815339008e-09, 3.8718696117833835e-09, 3.938261268497967e-09, 4.0021558789005335e-09, 4.064375171128178e-09, 4.125776397318854e-09, 4.187238746651813e-09, 4.2496604424331545e-09, 4.313953178694662e-09, 4.381043155833081e-09, 4.451862950811546e-09, 4.527347964114023e-09, 4.608424479457589e-09, 4.695978919300792e-09, 4.790833316547059e-09, 4.89368854406351e-09, 5.0050629523803745e-09, 5.125209537155244e-09, 5.2540210361110224e-09, 5.390941752573273e-09, 5.534891287544577e-09]}, {"Size parameters"=[1.1393590102632467, 1.1393590102632467, 1.1393590102632467, 1.5191453470176624, 1.5191453470176624, 1.5191453470176624, 1.8989316837720778, 1.8989316837720778, 1.8989316837720778, 2.2787180205264934, 2.2787180205264934, 2.2787180205264934, 2.658504357280909, 2.658504357280909, 2.658504357280909], [nan, 9.773817713343829e-11, 9.029304053343828e-11, nan, 3.7973880780896745e-10, 3.672280316089674e-10, nan, 1.0902236888049148e-09, 1.065072032804915e-09, nan, 2.0397810756454723e-09, 1.9797222216454726e-09, nan, 3.1844737627119423e-09, 3.1284761007119423e-09]}, {"Size parameters"=[1.1393590102632467, 1.5191453470176624, 1.8989316837720778, 2.2787180205264934, 2.658504357280909], [9.542777204943743e-11, 3.849904819901546e-10, 1.050837168490422e-09, 1.8964553943199e-09, 3.21838351648841e-09]}]
  out "Multiple charge correction term":cluster{"Size parameters":dbl[], dbl[]}(graph)={"Size parameters"=[1.1393590102632467, 1.5191453470176624, 1.8989316837720778, 2.2787180205264934, 2.658504357280909], [1.4598125268393792e-10, 2.005655775613868e-10, 1.5364460339416157e-10, 7.844564575651224e-11, 3.2158377368662943e-11]}
  in  "Baes data type definition":T8={"Extinction"=[], "Extinction Uncertainty"=[], "Size parameters"=[], "Number ofSizes"=0.0, "GeometricCrossSection"=[], "Wave Length"=0.0, "SMPS Sizes"=[], "Concentration"=[], "Double Charge Correction"=FALSE, "Extincation Factor"=1.0, "Diameter Factor"=1.0, "Diameter Offset"=0.0, "Extinction Factor Flag"=FALSE, "Diameter Factor Flag"=FALSE, "Diameter Offset Flag"=FALSE, "Sizes"=[], "ExtinctionOrAbsorptionOrScattering"=0} {"ExtinctionOrAbsorptionOrScattering" scale=0.0..2.0}
  in  "Retrieve RI without taking the mean (MC)":bool
  out "Loop index (MC) 2":i32=4
  in  "Retrieve RI Calculate lines seperately":bool
  out "MC progress":u8(slide)=5 max=5 scale=-1.0..5.0
  in  "Save RI MC":bool
  out "Saved RI (MC) to this filename and path":path=path "Z:/Dropbox/Lior Segev/Lior Segev Projects/RI retrieval in Labview/Data/SyntheticData/SRFA_Spectrafit1-RI-MC-result.xls"
  out "Saved RI to this filename and path":path=path "Z:/Dropbox/Lior Segev/Lior Segev Projects/RI retrieval in Labview/Data/SyntheticData/PahokeeSynthetic/data/PahokeeFake4nd-ApproxError-Error-Restricted_RIresult.txt"
  out "Time Left (min) (MC)":dbl=0.0242 format="%#.1f"
  out "Loop index (MC)":i32=4
  out "Imaginary Part MC":cluster{dbl[], dbl[]}[](graph)=[{[414.59], [0.0008685207556328173]}, {[414.59, 414.59, 414.59], [nan, 0.004360832212642005, -0.0026237907013763706]}]
  out "Real Part MC":cluster{dbl[], dbl[]}[](graph)=[{[414.59], [1.5002369861550031]}, {[414.59, 414.59, 414.59], [nan, 1.5023737313826764, 1.4981002409273299]}]
  in  "Size of statistics":i32=5 min=0 max=150 step=1
  in  "Retrieve RI (MC)":bool
  out "Not Corrected for Multiple charge Best fit result":T1(graph)=[{"Ramp Pattern"=[1.1393590102632467, 1.5191453470176624, 1.8989316837720778, 2.2787180205264934, 2.658504357280909], "Extinction"=[2.2661809e-10, 5.4746363e-10, 1.1996554e-09, 2.0678974e-09, 3.1780696e-09]}, {"Ramp Pattern"=[1.1393590102632467, 1.1393590102632467, 1.1393590102632467, 1.5191453470176624, 1.5191453470176624, 1.5191453470176624, 1.8989316837720778, 1.8989316837720778, 1.8989316837720778, 2.2787180205264934, 2.2787180205264934, 2.2787180205264934, 2.658504357280909, 2.658504357280909, 2.658504357280909], "Extinction"=[nan, 2.303406583e-10, 2.228955217e-10, nan, 5.537190181000001e-10, 5.412082419e-10, nan, 1.2122312279999999e-09, 1.187079572e-09, nan, 2.0979268269999997e-09, 2.037867973e-09, nan, 3.206068431e-09, 3.150070769e-09]}, {"Ramp Pattern"=[1.1393590102632467, 1.5191453470176624, 1.8989316837720778, 2.2787180205264934, 2.658504357280909], "Extinction"=[2.2782930008433976e-10, 5.58151556196404e-10, 1.173631806965889e-09, 1.955745494397593e-09, 3.2397709450082568e-09]}]
  out "Normalized Residuals vs Size parameter":T2(graph)=[{"Size parameters"=[1.1393590102632467, 1.5191453470176624, 1.8989316837720778, 2.2787180205264934, 2.658504357280909], "Normalized Residuals"=[0.325368669461459, 1.7085991051071756, -2.069330276750928, -3.7347310857393725, 2.2037097192348725]}]
  out "Imaginary Part vs wavelength":cluster{dbl[], dbl[]}[](graph)=[{[350.32001, 350.89999, 351.48999, 352.07001, 352.64001, 353.22, 353.79999, 354.37, 354.94, 355.51001, 356.07999, 356.64999, 357.22, 357.78, 358.35001, 358.91, 359.47, 360.03, 360.59, 361.14999, 361.70001, 362.26001, 362.81, 363.35999, 363.91, 364.45999, 365.01001, 365.56, 366.10001, 366.64999, 367.19, 367.73001, 368.26999, 368.81, 369.35001, 369.89001, 370.42001, 370.95999, 371.48999, 372.03, 372.56, 373.09, 373.62, 374.14999, 374.67999, 375.20999, 375.73001, 376.26001, 376.78, 377.31, 377.82999, 378.35001, 378.87, 379.39001, 379.91, 380.42999, 380.95001, 381.47, 381.98001, 382.5, 383.01001, 383.53, 384.04001, 384.54999, 385.07001, 385.57999, 386.09, 386.60001, 387.10999, 387.62, 388.13, 388.63, 389.14001, 389.64999, 390.14999, 390.66, 391.16, 391.67001, 392.17001, 392.67999, 389.64999, 390.14999, 390.66, 391.16, 391.67001, 392.17001, 392.67999, 393.17999, 393.67999, 394.17999, 394.67999, 395.19, 395.69, 396.19, 396.69, 397.19, 397.69, 398.19, 398.69, 399.19, 399.67999, 400.17999, 400.67999, 401.17999, 401.67999, 402.17001, 402.67001, 403.17001, 403.66, 404.16, 404.66, 405.14999, 405.64999, 406.14999, 406.64001, 407.14001, 407.64001, 408.13, 408.63, 409.13, 409.62, 410.12, 410.62, 411.10999, 411.60999, 412.10001, 412.60001, 413.10001, 413.60001, 414.09, 414.59, 415.09, 415.59, 416.07999, 416.57999, 417.07999, 417.57999, 418.07999, 418.57999, 419.07999, 419.57999, 420.07999, 420.57999, 421.07999, 421.57999, 422.07999, 422.57999, 423.09, 423.59, 424.09, 424.60001], [0.0032465245443988825, 0.016968699981331367, 0.005037666436984677, 0.01936742454426761, 0.02279093758917637, 0.02016760218392126, 0.017620429931402736, 0.027050954497160256, 0.02280122233144674, 0.021476830360551973, 0.028353294726249048, 0.02356415214116757, 0.027093510170658343, 0.040640367899250046, 0.03157699222944578, 0.027114399603122393, 0.034232110152277236, 0.035509103251145174, 0.04068536416000644, 0.03494289750495387, 0.03886384499272926, 0.03122774114998709, 0.041866583303920096, 0.03426940450675572, 0.03531236152989348, 0.034648618674496215, 0.03534046083383027, 0.03974478999617978, 0.036629905241561095, 0.03473353902726623, 0.030743827354715005, 0.03104417855947706, 0.03745144058806831, 0.03349695166256325, 0.030777343134365153, 0.03230507633820971, 0.02996607375960376, 0.029752518114942554, 0.03317049735256953, 0.03042214022724793, 0.03328364657382599, 0.0298859641083688, 0.03213062410782323, 0.03155198440422261, 0.03208173794083552, 0.03206269676429634, 0.027674130000977498, 0.025252949641615965, 0.03499659883769575, 0.027635368062602046, 0.033380887599540734, 0.026287442477049658, 0.026972927786426987, 0.026338335463461683, 0.029175787653240245, 0.016065785033701784, 0.0280005755486352, 0.03770952793845013, 0.020733597859613092, 0.025452126534518563, 0.029263289281719767, 0.0184168713552146, 0.02359655910592824, 0.022027178531908623, 0.011859986470408541, 0.02822974802983215, 0.01964879502143673, 0.030887667620897792, 0.014480422230023916, 0.032534117044465266, 0.01626315956548971, 0.018283923990351347, 0.024759052372106037, 0.015399317736444908, 0.027067549743449233, -0.0018236079784033448, -0.00032369057028436374, -0.003962513873249953, 0.010044920458841478, 0.0018630153637172848, 0.003291441139401014, -0.008061517736504863, 0.004960993390728122, 0.01693993161337472, 0.016826188906184134, 0.02693300936197654, 0.016476329345686852, 0.02660549400917228, 0.02784598379007515, 0.016141889892599265, 0.022214900618194207, 0.022547598559582813, 0.012701267631432929, 0.025226805058309456, 0.025426721795382627, 0.026591705885986697, 0.012260740380875646, 0.024118716648388532, 0.033363301610408166, 0.03296349297645204, 0.019404280574365204, 0.01732468526718023, 0.018528084756499554, 0.016167773665570314, 0.02949762887660318, 0.019926565644149664, 0.02659248674399744, 0.025392196865126906, 0.019489659350983245, 0.024104275269459012, 0.019739905134710318, 0.023208163652662532, 0.024520492819059526, 0.024907626701606192, 0.0185320369472174, 0.02417297054370946, 0.019857412619872124, 0.024652537501074483, 0.018995024642440777, 0.0194275375305571, 0.01897258480299092, 0.01524214226027398, 0.025452640681257622, 0.014936756577305652, 0.021580613873338372, 0.015208689195331495, 0.01120784030778366, 0.009153973845409087, 0.0195021318464305, 0.016288356747009437, 0.004718247335757715, 0.007597332025340498, 0.008934411009025773, 0.007175404877732928, 0.005732335932651022, 0.012900275231611871, 0.008112209857208846, 0.008946298250202829, 0.0044484880483105765, -0.00765963122398087, 0.0012481177977954156, 0.002513707030240866, 0.01131981169360136, 0.005074136454413231, 0.0035737428691112964, 0.0029461835419141913, -0.0050001317729657475, -0.033910587764534435, -0.02025979691748839, -0.022626314686973594, 0.0019796920484383444]}, ...(3 in all)]
  out "Real Part vs wavelength":cluster{dbl[], dbl[]}[](graph)=[{[350.32001, 350.89999, 351.48999, 352.07001, 352.64001, 353.22, 353.79999, 354.37, 354.94, 355.51001, 356.07999, 356.64999, 357.22, 357.78, 358.35001, 358.91, 359.47, 360.03, 360.59, 361.14999, 361.70001, 362.26001, 362.81, 363.35999, 363.91, 364.45999, 365.01001, 365.56, 366.10001, 366.64999, 367.19, 367.73001, 368.26999, 368.81, 369.35001, 369.89001, 370.42001, 370.95999, 371.48999, 372.03, 372.56, 373.09, 373.62, 374.14999, 374.67999, 375.20999, 375.73001, 376.26001, 376.78, 377.31, 377.82999, 378.35001, 378.87, 379.39001, 379.91, 380.42999, 380.95001, 381.47, 381.98001, 382.5, 383.01001, 383.53, 384.04001, 384.54999, 385.07001, 385.57999, 386.09, 386.60001, 387.10999, 387.62, 388.13, 388.63, 389.14001, 389.64999, 390.14999, 390.66, 391.16, 391.67001, 392.17001, 392.67999, 389.64999, 390.14999, 390.66, 391.16, 391.67001, 392.17001, 392.67999, 393.17999, 393.67999, 394.17999, 394.67999, 395.19, 395.69, 396.19, 396.69, 397.19, 397.69, 398.19, 398.69, 399.19, 399.67999, 400.17999, 400.67999, 401.17999, 401.67999, 402.17001, 402.67001, 403.17001, 403.66, 404.16, 404.66, 405.14999, 405.64999, 406.14999, 406.64001, 407.14001, 407.64001, 408.13, 408.63, 409.13, 409.62, 410.12, 410.62, 411.10999, 411.60999, 412.10001, 412.60001, 413.10001, 413.60001, 414.09, 414.59, 415.09, 415.59, 416.07999, 416.57999, 417.07999, 417.57999, 418.07999, 418.57999, 419.07999, 419.57999, 420.07999, 420.57999, 421.07999, 421.57999, 422.07999, 422.57999, 423.09, 423.59, 424.09, 424.60001], [1.6082150616930115, 1.6077943258027976, 1.6074953767596862, 1.6223823862387432, 1.6119126488351245, 1.6104408936100527, 1.6165398587127808, 1.6125082764908256, 1.6137473643686284, 1.615586969463532, 1.6154720248134051, 1.6134970778733049, 1.613409271211019, 1.6165778909911213, 1.6145851460277012, 1.6154072473919852, 1.6146513747787814, 1.6112255934129953, 1.6140014338462225, 1.615618904931255, 1.6143717140566856, 1.6115592873689435, 1.6118137512894386, 1.6079693852126162, 1.6108840562016167, 1.6090166644803525, 1.6112603639880534, 1.6103718307298391, 1.6077479011063285, 1.6041804540847275, 1.601714417348271, 1.6025803645525307, 1.6020973504905063, 1.5991488179700544, 1.6024185918286262, 1.5985539988441473, 1.5978626034447287, 1.5976750297763194, 1.598552322842027, 1.599885190470355, 1.599383435759499, 1.6028776412678654, 1.6003643351409538, 1.603318407132448, 1.5994122204522851, 1.5974692451735617, 1.5984442344114647, 1.5974618853263602, 1.5974618708987909, 1.5970862896031646, 1.5947991641009733, 1.5971956323451315, 1.594153673250688, 1.5936125916085184, 1.5957450510168307, 1.5929241559881082, 1.593208689715789, 1.594560243374521, 1.5903981531308133, 1.598002470090507, 1.5944690763761014, 1.5925204882691621, 1.5922040022042014, 1.598013464743186, 1.6001585417728268, 1.5928970205695112, 1.5958302965126676, 1.6007782934720762, 1.5911567338752228, 1.6027129361150978, 1.5947088613941691, 1.5911263129682698, 1.5969864438086123, 1.5900941235357504, 1.580380470801179, 1.5922854412521397, 1.5950535671916704, 1.5915880569252736, 1.5874040078615497, 1.5923407886626997, 1.5765365443414265, 1.5908326574650498, 1.5915454112521306, 1.5793573743704725, 1.575168342585465, 1.5849310656864697, 1.5836007127537663, 1.5874627120100984, 1.5794196934306153, 1.584119066928443, 1.5858382892804097, 1.5947438137619612, 1.5926095848294728, 1.5862087701468583, 1.580187427051917, 1.5814658686177987, 1.5893557736261603, 1.5890216649537376, 1.5843997176183158, 1.5870628176797883, 1.5903474806183024, 1.5861924149084734, 1.591176664530558, 1.589386255233374, 1.5850030554512955, 1.5894970006526254, 1.5899115164244704, 1.5930367033262134, 1.588315136776235, 1.5874493103660747, 1.5876993354601736, 1.5924206398938778, 1.5876289483739945, 1.5894394324453454, 1.589758612276476, 1.5866667068669236, 1.5875566094957656, 1.5882490248589205, 1.5911626299327652, 1.5880954463147767, 1.588059994105508, 1.5898918629447971, 1.5883646152295943, 1.5887267355049803, 1.5852681159424749, 1.5883721242582771, 1.587939899514784, 1.590159323633305, 1.5826360995824014, 1.5834161767218957, 1.5877181195386574, 1.5883366780204837, 1.5876053120131373, 1.5899303474533073, 1.5918023983505254, 1.583182689229695, 1.58555388203875, 1.5831404838321699, 1.579203890316478, 1.5881340358552638, 1.5832538207896207, 1.5829868986081963, 1.5865412477336516, 1.5828814734066992, 1.583913498792347, 1.5798499276728604, 1.5772784524001084, 1.590113229148155, 1.5890578729777407, 1.5874694403131198, 1.5804453509322545]}, ...(3 in all)]
  in  "OK":bool
  # "Finding Factors is performed on only a single wavelength"
  # "Developed by Lior Segev\nsegev.lior@gmail.com\nYinon Rudich's Group\nDepartment of Earth and Planetary Sciences\n09 Dec 2013\nVer 1.0"
  # "Factors that minimize \nthe residue"
  # "Extinction Factor"
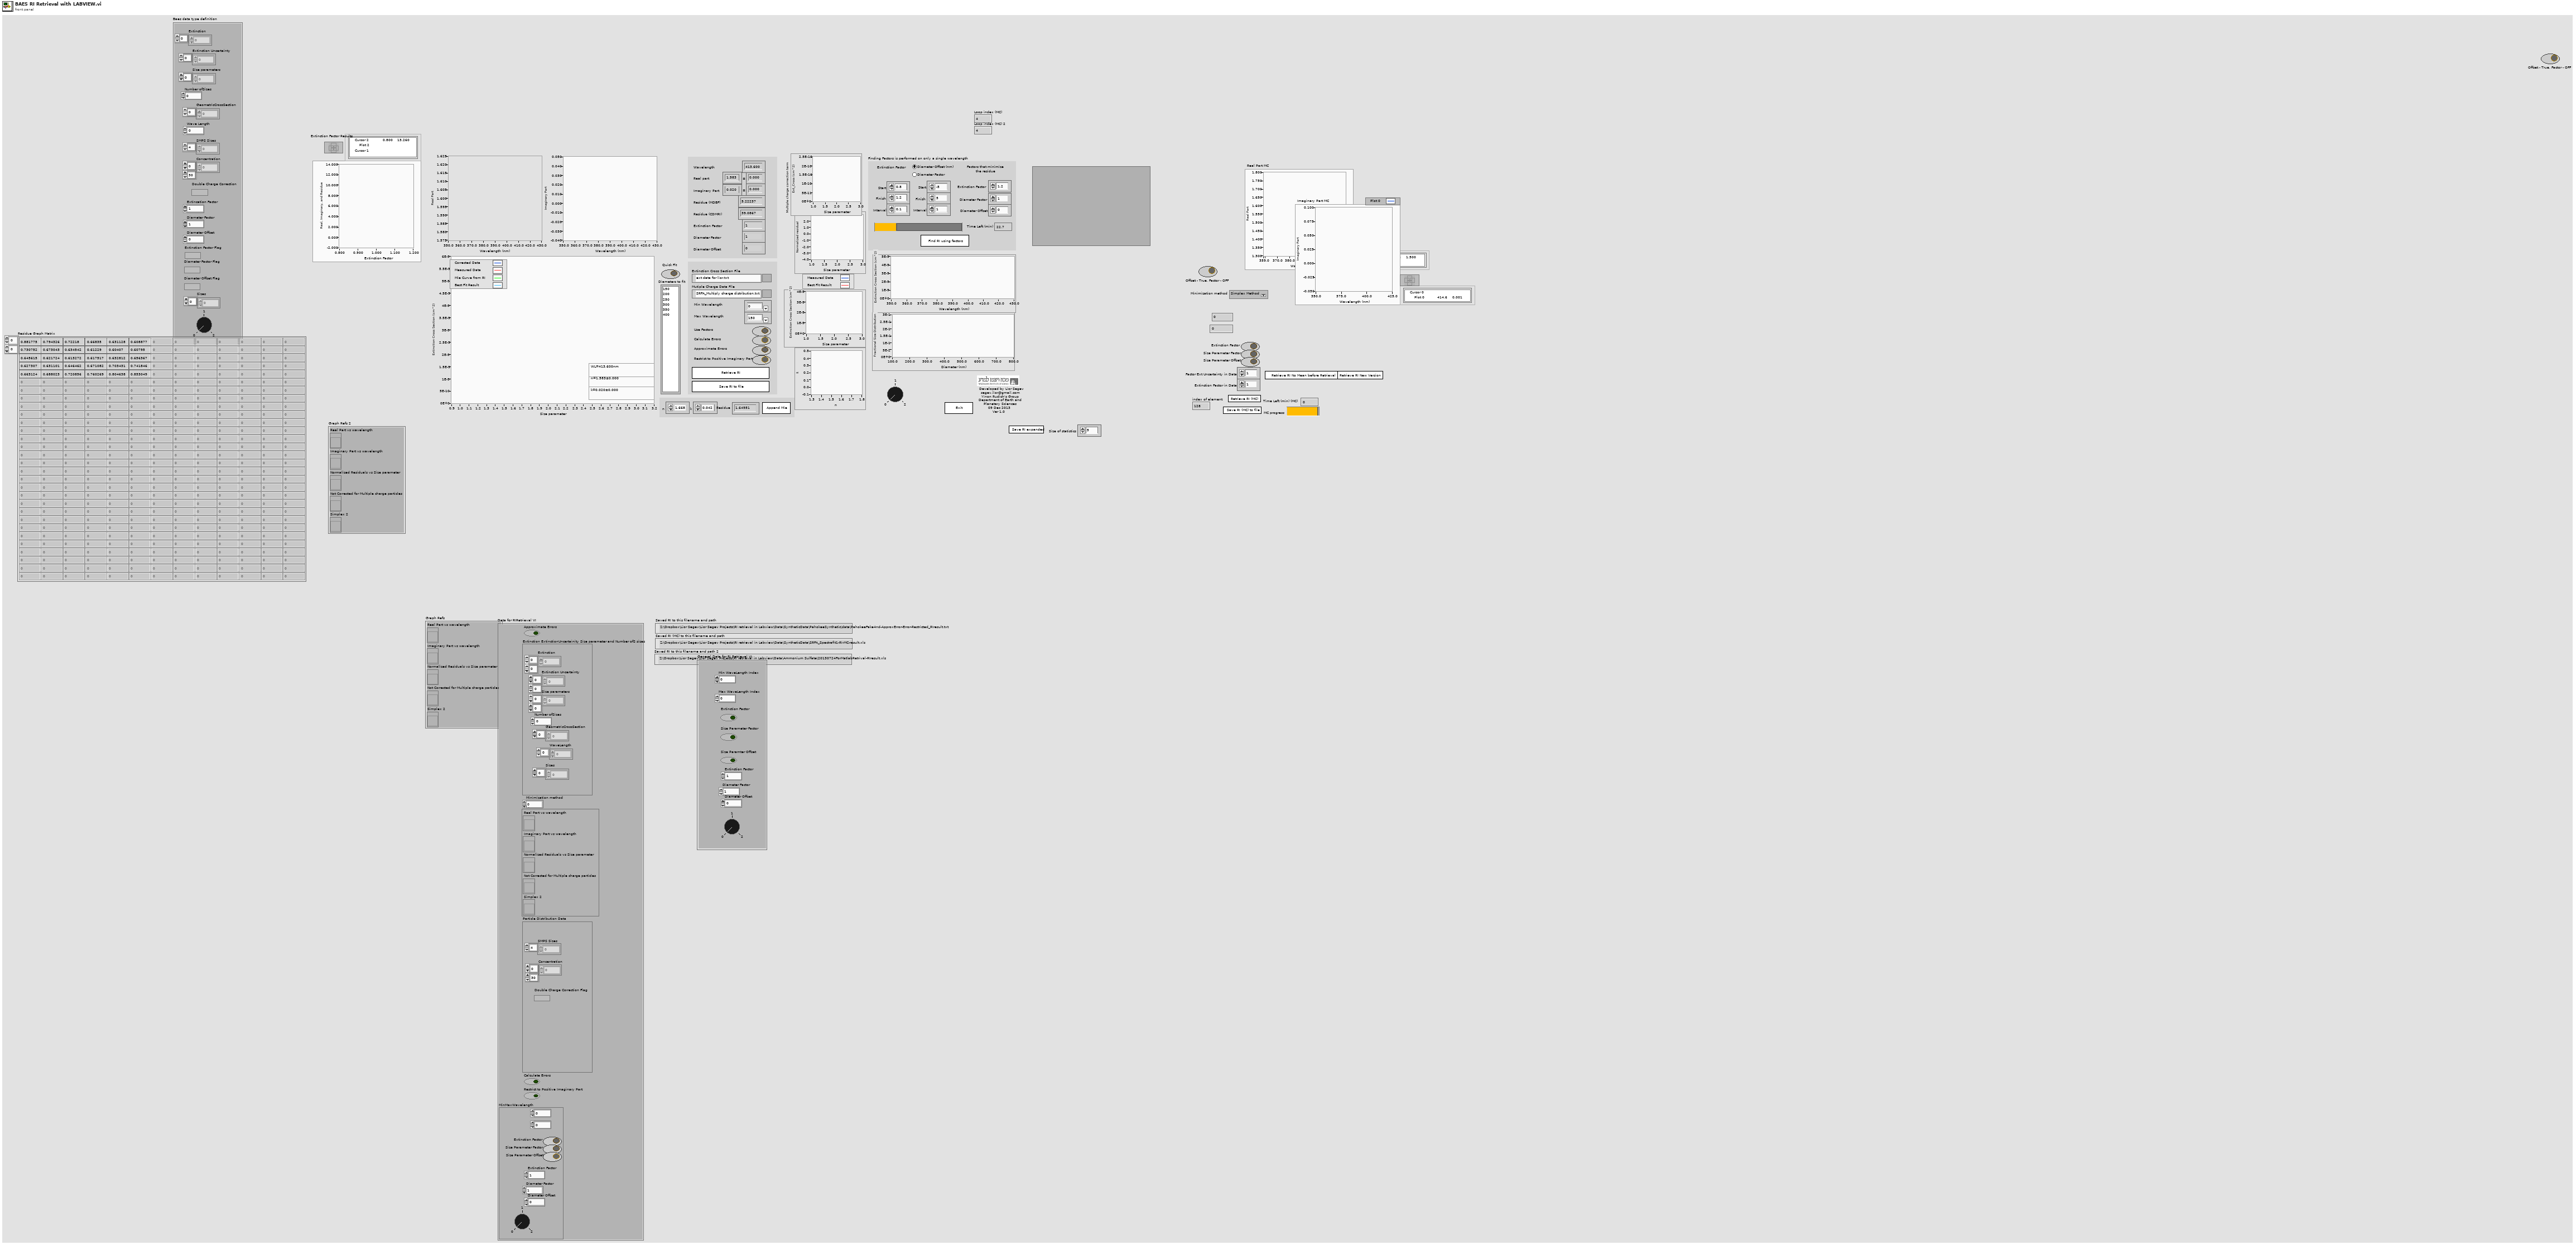
[diagram p1: front panel]
types:
  T1 = cluster{"Ramp Pattern":dbl[], "Extinction":dbl[]}[]
  T2 = cluster{"Size parameters":dbl[], "Normalized Residuals":dbl[]}[]
  T3 = typedef "GeneralDataForRIRetrieval.ctl" = cluster{"Min WaveLength Index":u16, "Max WaveLength Index":u16, "Extinction Factor":bool, "Size Parameter Factor":bool, "Size Paramter Offset":bool, "Extinction Factor":dbl, "Diameter Factor":dbl, "Diameter Offset":dbl, "ExtinctionOrAbsorptionOrScattering":i8}
  T4 = cluster{"Real Part vs wavelength":refnum<vi>, "Imaginary Part vs wavelength":refnum<vi>, "Normalized Residuals vs Size parameter":refnum<vi>, "Not Corrected for Multiple charge particles":refnum<vi>, "Simplex 2":refnum<vi>}
  T5 = typedef "ReadBaesDataTypeDefinition.ctl" = cluster{"Extinction":dbl[][], "Extinction Uncertainty":dbl[][], "Size parameters":dbl[][], "Number ofSizes":dbl, "GeometricCrossSection":dbl[], "WaveLength":dbl[], "Sizes":dbl[]}
  T6 = typedef "ParticleDistributionData.ctl" = cluster{"SMPS Sizes":dbl[], "Concentration":dbl[][], "Double Charge Correction Flag":bool}
  T7 = cluster{"Approximate Errors":bool, "Extinction ExtinctionUncertainity Size parameter and Number ofS sizes":T5, "Minimization method":u16, "Graph Ref":cluster{"Real Part vs wavelength":refnum<vi>, "Imaginary Part vs wavelength":refnum<vi>, "Normalized Residuals vs Size parameter":refnum<vi>, "Not Corrected for Multiple charge particles":refnum<vi>, "Simplex 2":refnum<vi>}, "Particle Distribution Data":T6, "Calculate Errors":bool, "Restrict to Positive Imaginary Part":bool, "MinMaxWavelength":cluster{i32, i32, "Extinction Factor":bool, "Size Parameter Factor":bool, "Size Parameter Offset":bool, "Extinction Factor":dbl, "Diameter Factor":dbl, "Diameter Offset":dbl, "ExtinctionOrAbsorptionOrScattering":i8}}
  T8 = typedef "BaesDataTypeDefinition.ctl" = cluster{"Extinction":dbl[], "Extinction Uncertainty":dbl[], "Size parameters":dbl[], "Number ofSizes":dbl, "GeometricCrossSection":dbl[], "Wave Length":dbl, "SMPS Sizes":dbl[], "Concentration":dbl[][], "Double Charge Correction":bool, "Extincation Factor":dbl, "Diameter Factor":dbl, "Diameter Offset":dbl, "Extinction Factor Flag":bool, "Diameter Factor Flag":bool, "Diameter Offset Flag":bool, "Sizes":dbl[], "ExtinctionOrAbsorptionOrScattering":i8}
  T9 = enum32{"invalid app kind", "Development System", "Run Time System", "Student Edition", "Embedded LabVIEW", "Evaluation", "Custom"}
  T10 = enum32{"Invalid", "Standard", "Closed", "Hidden", "Minimized", "Maximized"}
  T11 = typedef "NI_Gmath.lvlib/stopping criteria.ctl" = cluster{"function tolerance":dbl, "parameter tolerance":dbl, "max iterations":i32, "max function calls":i32, "gradient tolerance":dbl, "max time (sec)":dbl}
  T12 = typedef "LVPoint32TypeDef.ctl" = cluster{"Horizontal":i32, "Vertical":i32}
  T13 = typedef "RIandRIMCResults.ctl" = cluster{"Real RI":dbl[], "Imaginary RI":dbl[], "Std Imaginary RI":dbl[], "Std Real RI":dbl[], "Wavelength":dbl[], "Residue":dbl[], "Extinction Factor":dbl[], "Diameter Factor":dbl[], "Diameter Offset":dbl[], "Best fit result":dbl[][], "Normalized Residuals":dbl[][]}
  T14 = cluster{"Core":cluster{"Current VI Reference":refnum<vi>, "Close Panel on Exit?":bool}, "Extinction ExtinctionUncertainity Size parameter and Number ofS sizes":T5, "Particle Distribution Data":T6, "RI results":T13, "RI MC results":T13, "Extinction Cross section Path":path, "Multiple charge correction file Path":path, "FullExtinctionData":dbl[][], "NumberOfMeasurementsperSize":i32, "Baes data type definition":T8}
  T15 = cluster{"Current VI Reference":refnum<vi>, "Close Panel on Exit?":bool}
  T16 = cluster{"WaveLengths":dbl[], "Extinction":dbl[]}[]
  T17 = cluster{"Size parameters":dbl[], "Extinction Crosssections":dbl[]}
  T18 = cluster{"Size parameters":dbl[], "Extinction Crosssections":dbl[]}[]
  T19 = cluster{"Real Part vs wavelength":refnum<vi>, "Imaginary Part vs wavelength":refnum<vi>, "Normalized Residuals vs Size parameter":refnum<vi>, "Not Corrected for Multiple charge Best fit result":refnum<vi>, "Simplex":refnum<vi>}
  T20 = typedef "NI_Matrix.lvlib/RealMatrix.ctl" = dbl[][]
  T21 = cluster{"Size parameters":dbl[], "Extinction":dbl[]}
  T22 = cluster{"Size parameters":dbl[], "Normalized Residuals":dbl[]}
  T23 = cluster{"Size parameters":dbl[], "Best fit result":dbl[]}
  T24 = cluster{"Size parameters":dbl[], "Best fit result":dbl[]}[]
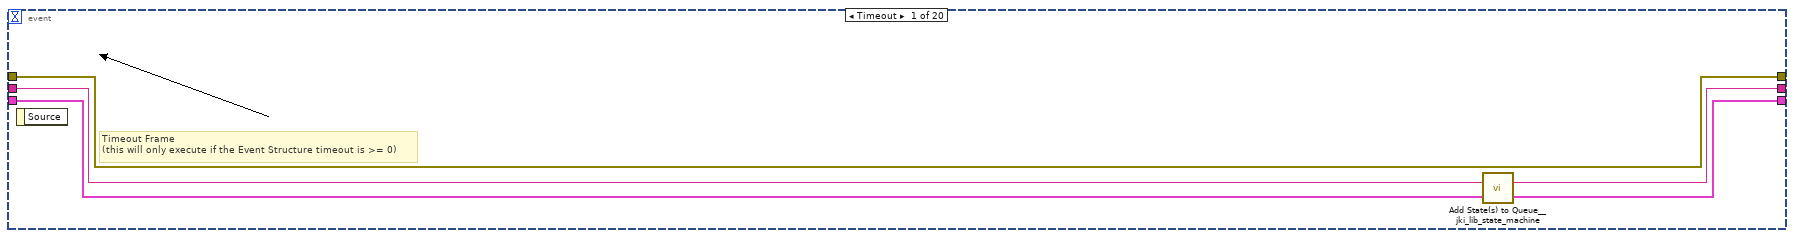
[diagram p2: hidden frame]
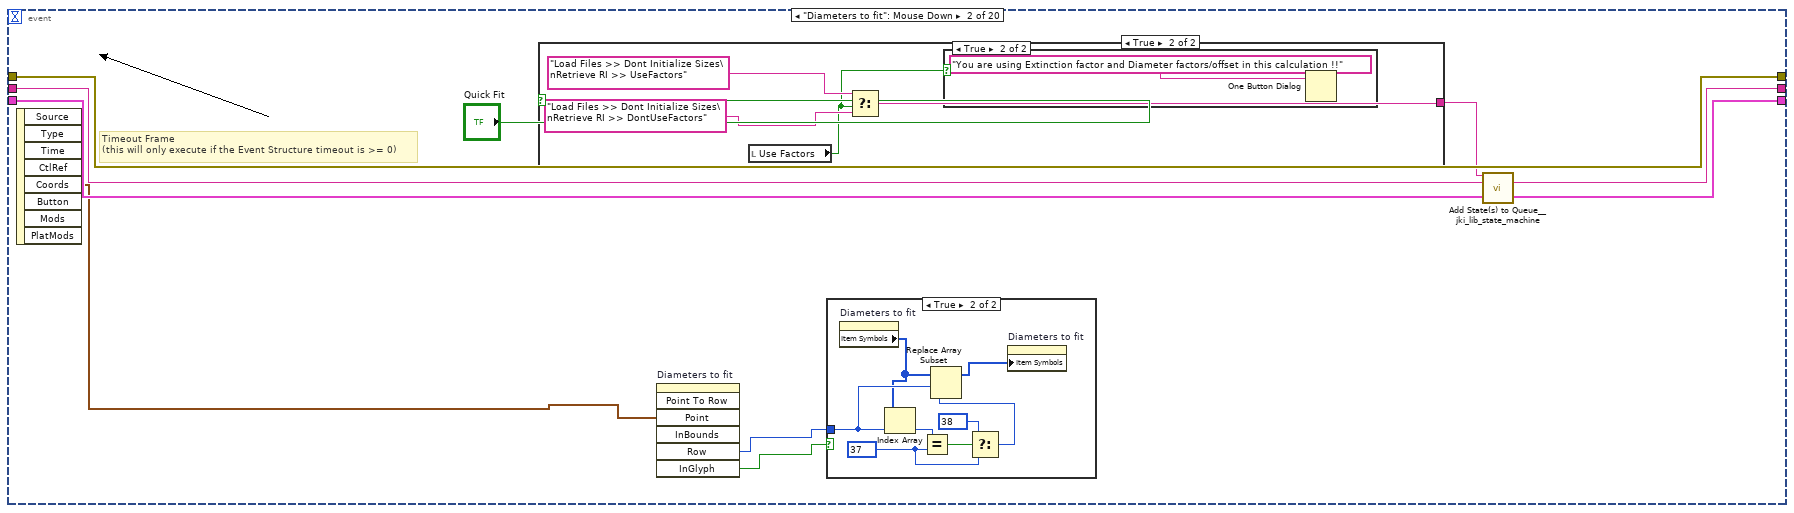
[diagram p3: hidden frame]
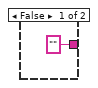
[diagram p4: hidden frame]
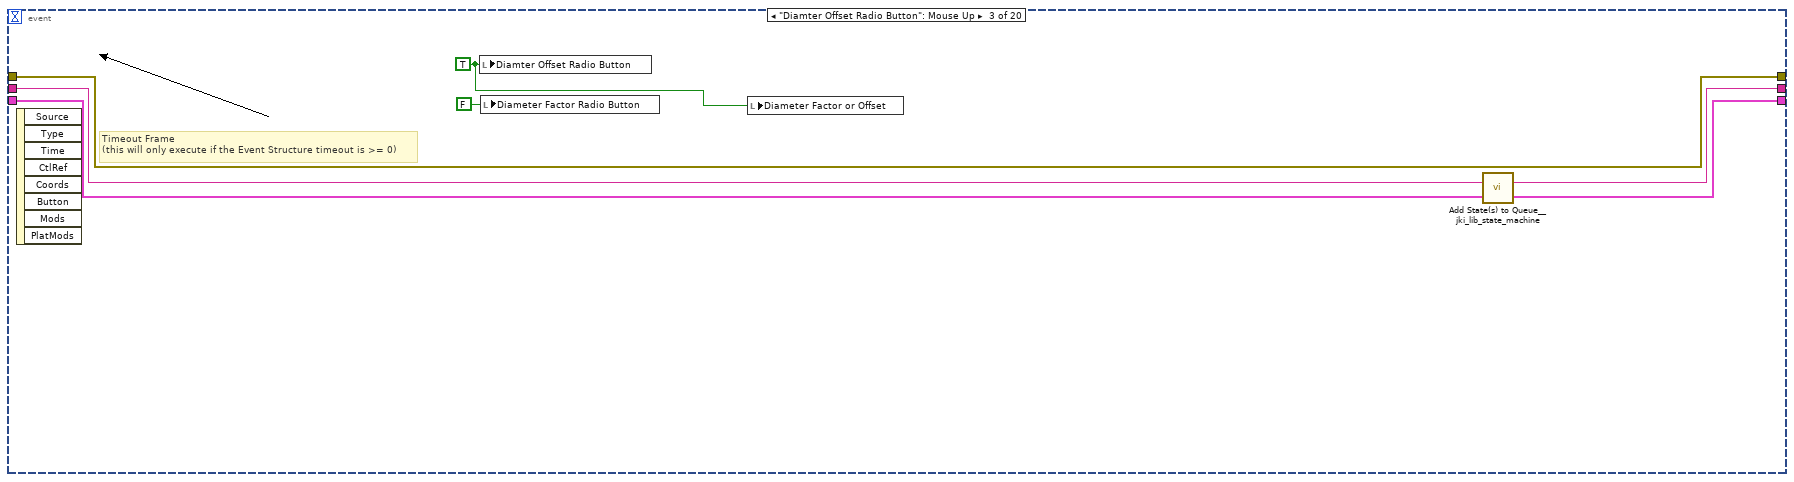
[diagram p7: hidden frame]
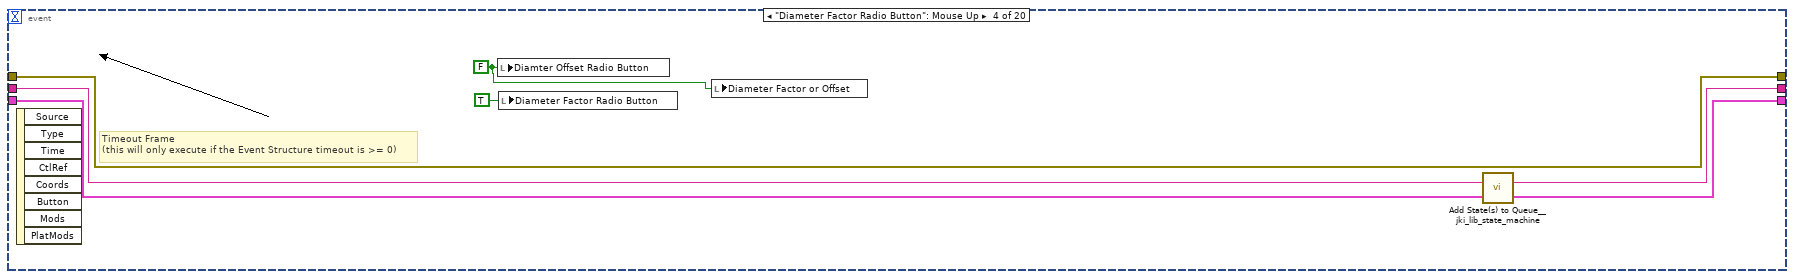
[diagram p8: hidden frame]
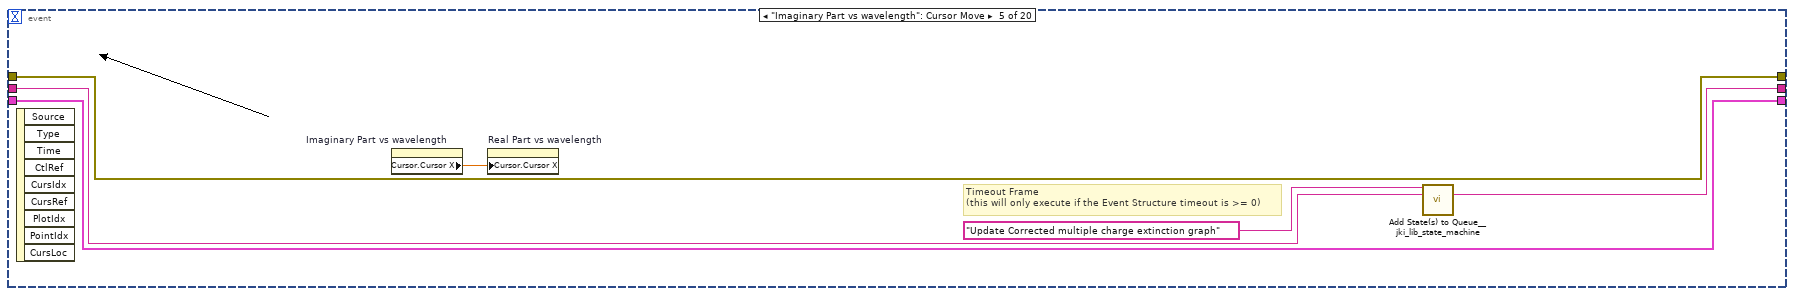
[diagram p9: hidden frame]
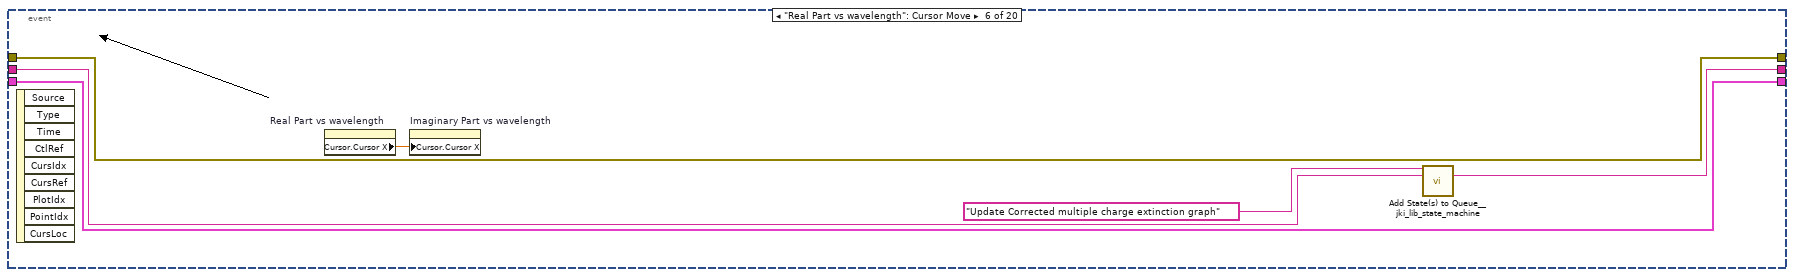
[diagram p10: hidden frame]
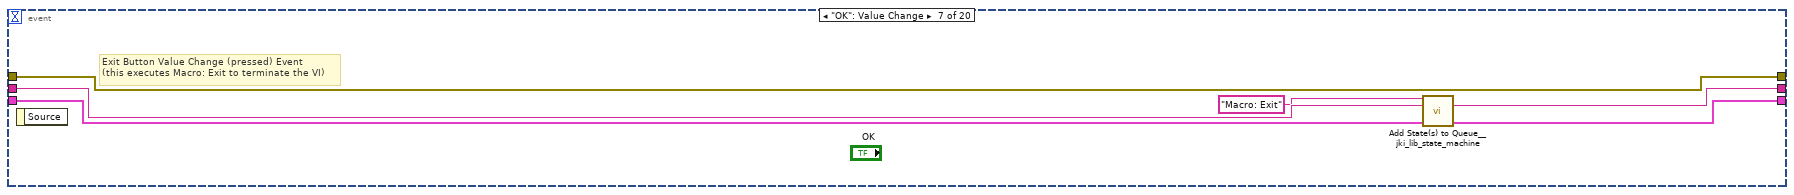
[diagram p11: hidden frame]
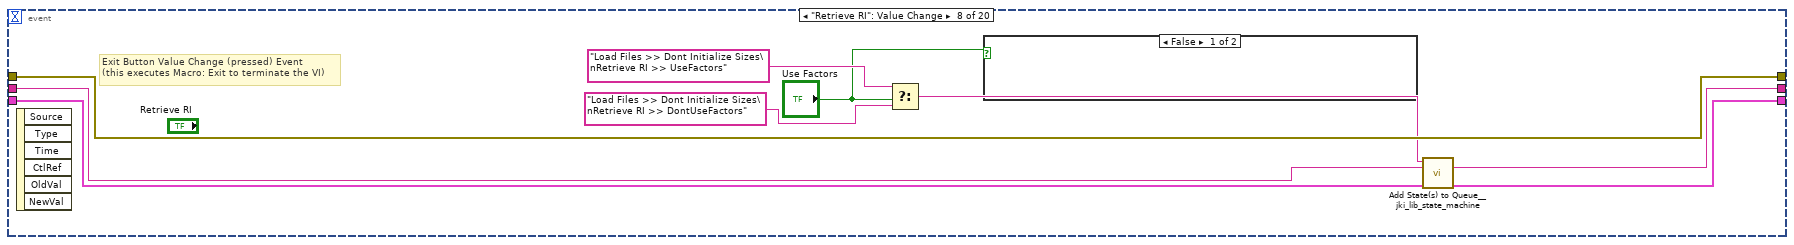
[diagram p12: hidden frame]
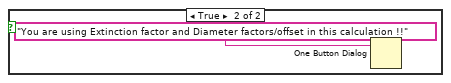
[diagram p13: hidden frame]
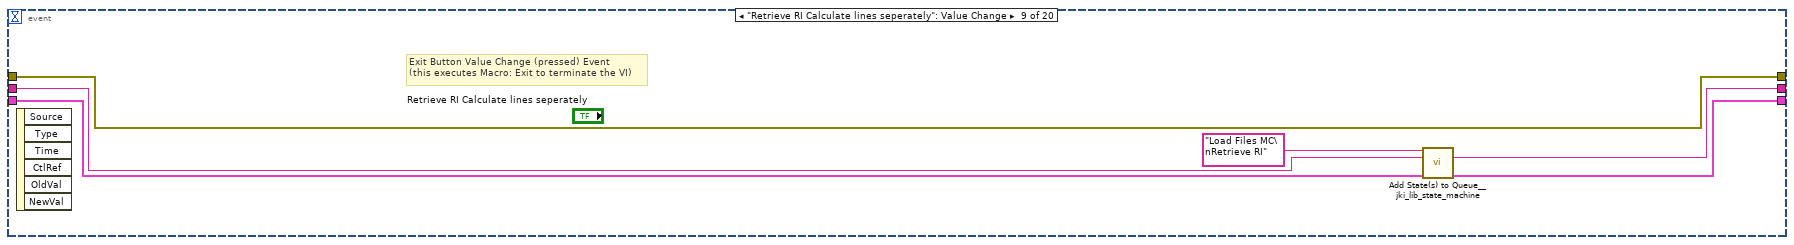
[diagram p14: hidden frame]
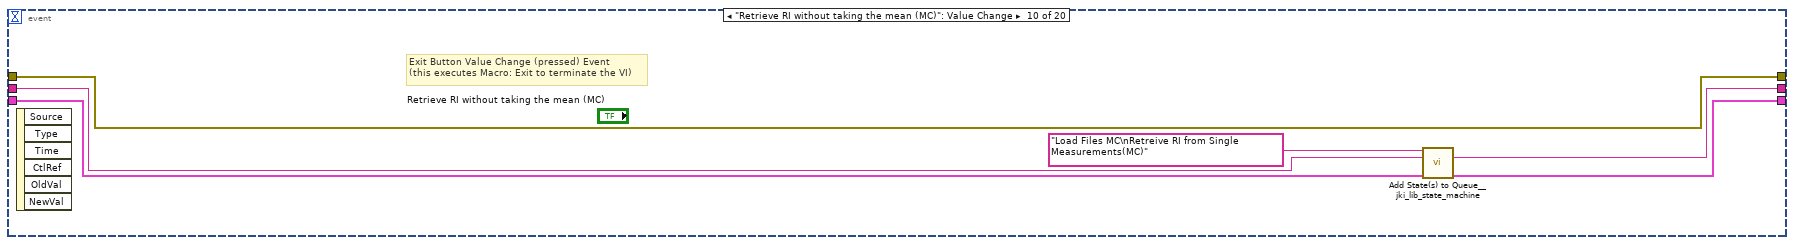
[diagram p15: hidden frame]
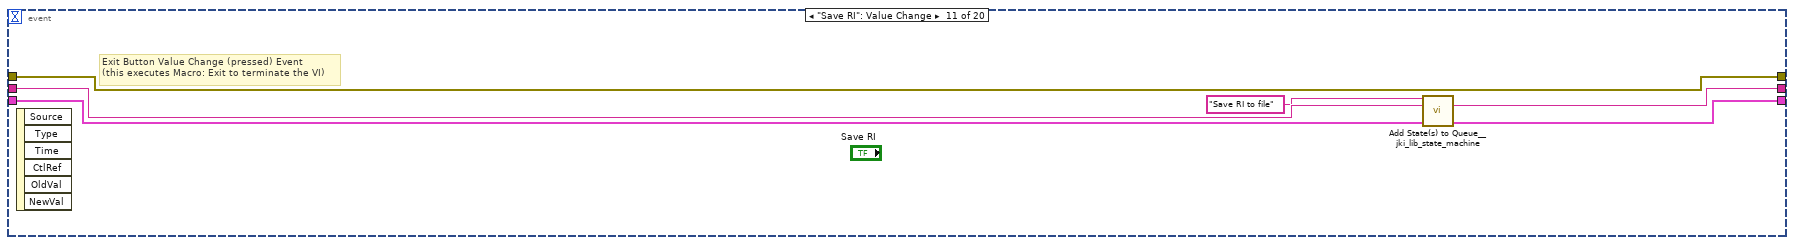
[diagram p16: hidden frame]
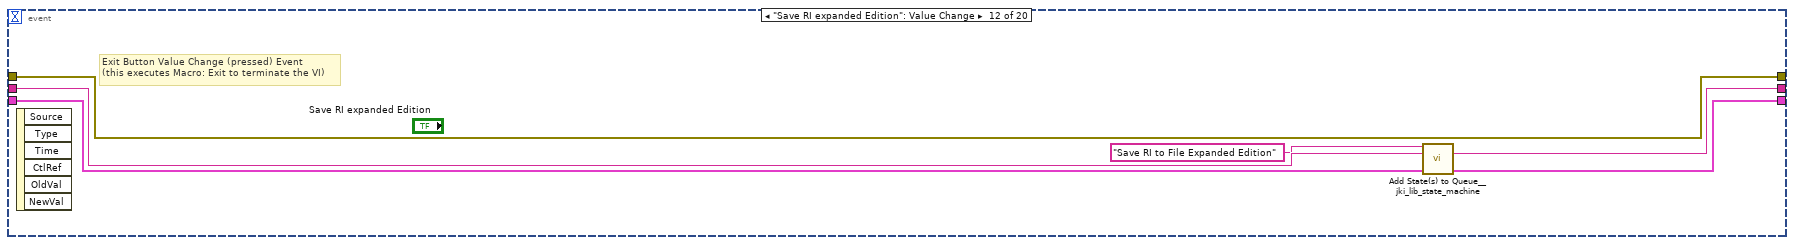
[diagram p17: hidden frame]
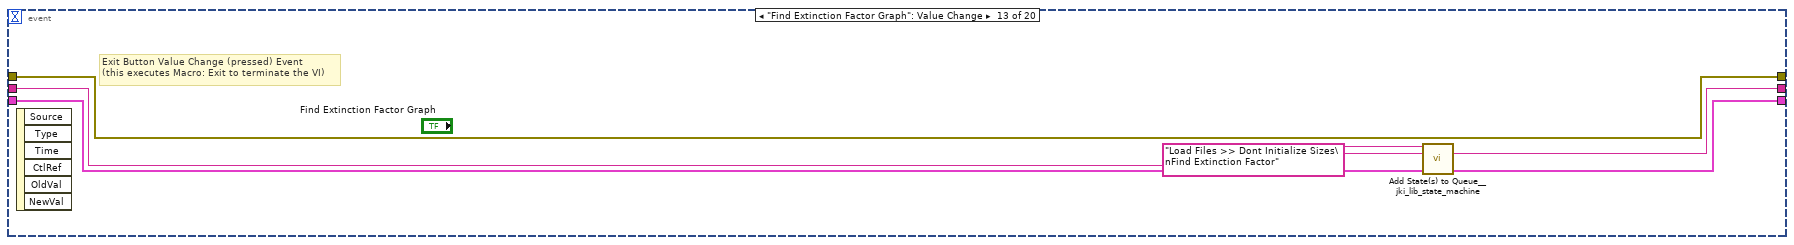
[diagram p18: hidden frame]
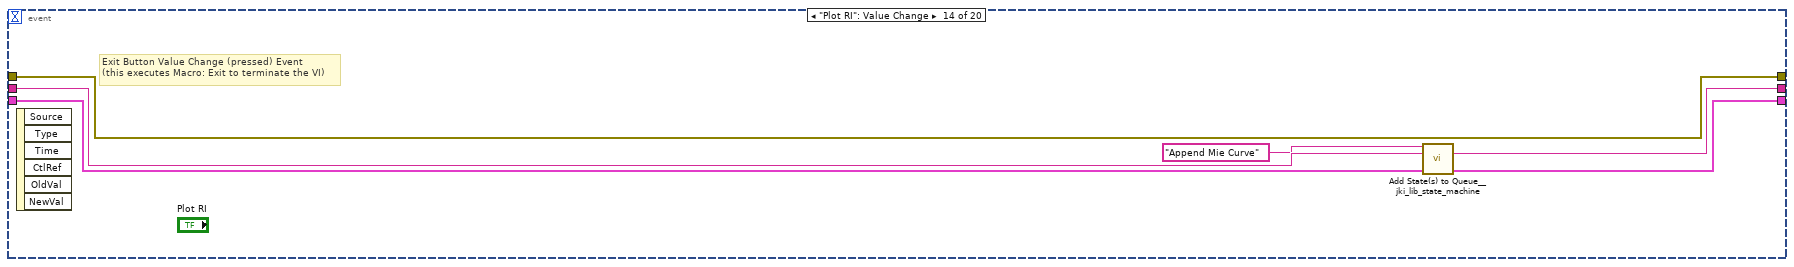
[diagram p19: hidden frame]
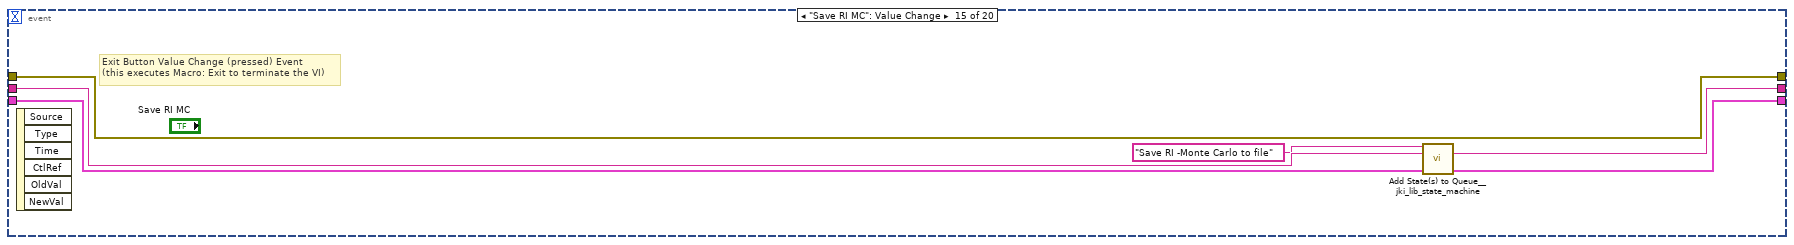
[diagram p20: hidden frame]
diagram:
  (unwired) cluster{dbl[], dbl[]}[] [{[353.79999, 354.37, 354.94, 355.51001, 356.07999, 356.64999, 357.22, 357.78, 358.35001, 358.91, 359.47, 360.03, 360.59, 361.14999, 361.70001, 362.26001, 362.81, 363.35999, 363.91, 364.45999, 365.01001, 365.56, 366.10001, 366.64999, 367.19, 367.73001, 368.26999, 368.81, 369.35001, 369.89001, 370.42001, 370.95999, 371.48999, 372.03, 372.56, 373.09, 373.62, 374.14999, 374.67999, 375.20999, 375.73001, 376.26001, 376.78, 377.31, 377.82999, 378.35001, 378.87, 379.39001, 379.91, 380.42999, 380.95001, 381.47, 381.98001, 382.5, 383.01001, 383.53, 384.04001, 384.54999, 385.07001, 385.57999, 386.09, 386.60001, 387.10999, 387.62, 388.13, 388.63, 389.14001, 389.64999, 390.14999, 388.63, 389.14001, 389.64999, 390.14999, 390.66, 391.16, 391.67001, 392.17001, 392.67999, 393.17999, 393.67999, 394.17999, 394.67999, 395.19, 395.69, 396.19, 396.69, 397.19, 397.69, 398.19, 398.69, 399.19, 399.67999, 400.17999, 400.67999, 401.17999, 401.67999, 402.17001, 402.67001, 403.17001, 403.66, 404.16, 404.66, 405.14999, 405.64999, 406.14999, 406.64001, 407.14001, 407.64001, 408.13, 408.63, 409.13, 409.62, 410.12, 410.62, 411.10999, 411.60999, 412.10001, 412.60001, 413.10001, 413.60001, 414.09, 414.59, 415.09, 415.59, 416.07999, 416.57999, 417.07999, 417.57999, 418.07999, 418.57999], [-0.006880589406937364, -0.005591015240643177, -0.0008128900086740067, 0.0059132125129690355, 0.004727233671001155, 0.005285323022981176, 0.012079702376504426, 0.013295932917972094, 0.009723681324539938, 0.01340675951578305, 0.014300736755976685, 0.017412400216708195, 0.016082847953221062, 0.019541949361009746, 0.016681812204333245, 0.021839119627984467, 0.01917857630542129, 0.01659316249089897, 0.017920546232635386, 0.02331211752971285, 0.018736628440528875, 0.02278859303667559, 0.020160162589600072, 0.01944517701034782, 0.01722059774576336, 0.014545686876081154, 0.017064244530774875, 0.014871257634513302, 0.015814167710632307, 0.012323804928601011, 0.017001137568295226, 0.01761462364709586, 0.011094176200131175, 0.013484050217230092, 0.015463713328499572, 0.017445979654003158, 0.017890194826904918, 0.012171772373985729, 0.0090971027467458, 0.010861800449201833, 0.009486644105636509, 0.009660218265489668, 0.011543706295196892, 0.009241826302022669, 0.0043825353242573275, 0.006012733183160885, 0.016684276899031823, 0.004574877464619924, 0.004680287507653695, 0.005436664247245053, 0.005769621008366801, 0.007016844481986471, 0.005292591657780566, 0.0023362286578048827, 0.001404106784902966, 0.006018627453886426, 0.005868676603131451, 0.004574542292684771, 0.00013407550315604303, 0.005111191491887428, 0.006244050999230227, 0.008470422941900313, 0.0019502929036388976, 0.00693045579799217, 0.00729891092487377, 0.006591697414114595, -0.00464719874347794, -0.0028833235584898023, 0.0030601034901337606, -0.019172722466464624, 0.00349415319418767, -0.019612863241454764, 0.006230360324734642, -0.007644525136092856, -0.0024464061374237676, -0.015743142364772214, -0.01362771525815333, 0.0023827303007783484, 0.004434076127836306, 0.0015447059453072153, -0.0012530544220862782, 0.013970670419985256, 0.005734164261953947, 0.008763635301725982, 0.006956973905904259, 0.0058963200240359104, 0.004165371933482626, 0.009600835719607804, 0.0037134970421865933, 0.01607998543651406, 0.007081749858913052, 0.014576117182728877, 0.010330077196118458, 0.013431346724388227, 0.009247446675431951, 0.013068538923394903, 0.009279456157815679, 0.013932752616816237, 0.013225407198184207, 0.014934507206195071, 0.017106424708032086, 0.01564773346122451, 0.017710188001506998, 0.011882676676028447, 0.014042275741809086, 0.014230648119115306, 0.011795090172377915, 0.01414643231400618, 0.01678394258342081, 0.006007592633110041, 0.012137073369673021, 0.015868997327494014, 0.008004974625515329, 0.012176508619891986, 0.011391254549822344, 0.01562344561258754, 0.005349593450524416, 0.012534566898108031, 0.015731735948216675, 0.012454435731493445, 0.016355219901748506, 0.007853560039517043, 0.0044201289692190875, 0.009950585420452563, 0.0011992242078176175, -0.0040610702724316675, 0.005166605821146673, 0.00788498225462348, -0.004714349788695529, 0.007145714404910847]}, ...(3 in all)] ("Imaginary Part vs wavelength")
  (unwired) cluster{dbl[], dbl[]}[] [{[353.79999, 354.37, 354.94, 355.51001, 356.07999, 356.64999, 357.22, 357.78, 358.35001, 358.91, 359.47, 360.03, 360.59, 361.14999, 361.70001, 362.26001, 362.81, 363.35999, 363.91, 364.45999, 365.01001, 365.56, 366.10001, 366.64999, 367.19, 367.73001, 368.26999, 368.81, 369.35001, 369.89001, 370.42001, 370.95999, 371.48999, 372.03, 372.56, 373.09, 373.62, 374.14999, 374.67999, 375.20999, 375.73001, 376.26001, 376.78, 377.31, 377.82999, 378.35001, 378.87, 379.39001, 379.91, 380.42999, 380.95001, 381.47, 381.98001, 382.5, 383.01001, 383.53, 384.04001, 384.54999, 385.07001, 385.57999, 386.09, 386.60001, 387.10999, 387.62, 388.13, 388.63, 389.14001, 389.64999, 390.14999, 388.63, 389.14001, 389.64999, 390.14999, 390.66, 391.16, 391.67001, 392.17001, 392.67999, 393.17999, 393.67999, 394.17999, 394.67999, 395.19, 395.69, 396.19, 396.69, 397.19, 397.69, 398.19, 398.69, 399.19, 399.67999, 400.17999, 400.67999, 401.17999, 401.67999, 402.17001, 402.67001, 403.17001, 403.66, 404.16, 404.66, 405.14999, 405.64999, 406.14999, 406.64001, 407.14001, 407.64001, 408.13, 408.63, 409.13, 409.62, 410.12, 410.62, 411.10999, 411.60999, 412.10001, 412.60001, 413.10001, 413.60001, 414.09, 414.59, 415.09, 415.59, 416.07999, 416.57999, 417.07999, 417.57999, 418.07999, 418.57999], [1.6483722836524246, 1.6546363395359365, 1.647298907653894, 1.6533287796168583, 1.6513909602141936, 1.6441728100483295, 1.6485630092327472, 1.6465913680498476, 1.644326968253007, 1.6458723273169005, 1.6423749873362237, 1.6435071871004756, 1.6412154858600103, 1.6396834087598822, 1.6391132715105765, 1.6382846511661762, 1.6358307684719318, 1.6354408519662669, 1.6334428509272396, 1.6328074965992703, 1.630211530333035, 1.629597879928187, 1.6276773015694914, 1.6248549924331006, 1.6221911228582016, 1.619860370624227, 1.6186660879658288, 1.6177483954461045, 1.618059125989092, 1.616294733806861, 1.6164932554209357, 1.6163255198620012, 1.615138021497404, 1.6164105257665495, 1.617235077199874, 1.6147912416880703, 1.6164196882297972, 1.6150368907017385, 1.6144850551191468, 1.6133228562399728, 1.6128153905854543, 1.6139403869979996, 1.6131967111234533, 1.6143159173824806, 1.6121220874076225, 1.6114366661699004, 1.6094507790415067, 1.6108839833096118, 1.6122492163476982, 1.6122322997299472, 1.6077321043459216, 1.6138723793940135, 1.6118005408009028, 1.6157486465235684, 1.6147077896853421, 1.6142964675684908, 1.614804272990439, 1.6117647309822476, 1.6161328124848642, 1.6101356911507883, 1.612094662439775, 1.6118531546799915, 1.614236269971587, 1.6062328837497617, 1.6105586500151539, 1.6108228692284308, 1.6178782024106462, 1.6087987962691102, 1.6074587087659151, 1.6187364188290658, 1.6209092605148896, 1.6151493452793495, 1.6182798966697, 1.6109338276299237, 1.6085077651242317, 1.613655399235577, 1.612511934789509, 1.607851046633587, 1.6057532268507935, 1.6024870719133475, 1.6038884748636346, 1.605523559015856, 1.5960101592112506, 1.5997312604952778, 1.598377877440321, 1.597392154092918, 1.600589807386528, 1.5995684913350448, 1.5979434008328421, 1.5961998900762004, 1.5970150338732805, 1.5939307380342091, 1.596156816544494, 1.5962182334684933, 1.597512896681686, 1.595101996088882, 1.5933960300930927, 1.592688229676817, 1.5913322143224218, 1.5917530088094214, 1.591614538502429, 1.5914637114820218, 1.5878221602705458, 1.5928834293750267, 1.5915729711917386, 1.587309104722474, 1.5918112038963161, 1.5881066262119135, 1.584965267353939, 1.5914289179893895, 1.586911737372422, 1.581731065142223, 1.5886590769172397, 1.5849680475176062, 1.586099454232746, 1.581195601241917, 1.5854707251659343, 1.5865012245981702, 1.5838978086861526, 1.584800751487047, 1.5848505559733816, 1.5857486239152707, 1.585591816537336, 1.5810404634087085, 1.5851743649291072, 1.5859104770394237, 1.5823664432736304, 1.5792071958230995, 1.590530467368216, 1.5870072549949592]}, {[353.79999, 353.79999, 353.79999, 354.37, 354.37, 354.37, 354.94, 354.94, 354.94, 355.51001, 355.51001, 355.51001, 356.07999, 356.07999, 356.07999, 356.64999, 356.64999, 356.64999, 357.22, 357.22, 357.22, 357.78, 357.78, 357.78, 358.35001, 358.35001, 358.35001, 358.91, 358.91, 358.91, 359.47, 359.47, 359.47, 360.03, 360.03, 360.03, 360.59, 360.59, 360.59, 361.14999, 361.14999, 361.14999, 361.70001, 361.70001, 361.70001, 362.26001, 362.26001, 362.26001, 362.81, 362.81, 362.81, 363.35999, 363.35999, 363.35999, 363.91, 363.91, 363.91, 364.45999, 364.45999, 364.45999, 365.01001, 365.01001, 365.01001, 365.56, 365.56, 365.56, 366.10001, 366.10001, 366.10001, 366.64999, 366.64999, 366.64999, 367.19, 367.19, 367.19, 367.73001, 367.73001, 367.73001, 368.26999, 368.26999, 368.26999, 368.81, 368.81, 368.81, 369.35001, 369.35001, 369.35001, 369.89001, 369.89001, 369.89001, 370.42001, 370.42001, 370.42001, 370.95999, 370.95999, 370.95999, 371.48999, 371.48999, 371.48999, 372.03, 372.03, 372.03, 372.56, 372.56, 372.56, 373.09, 373.09, 373.09, 373.62, 373.62, 373.62, 374.14999, 374.14999, 374.14999, 374.67999, 374.67999, 374.67999, 375.20999, 375.20999, 375.20999, 375.73001, 375.73001, 375.73001, 376.26001, 376.26001, 376.26001, 376.78, 376.78, 376.78, 377.31, 377.31, 377.31, 377.82999, 377.82999, 377.82999, 378.35001, 378.35001, 378.35001, 378.87, 378.87, 378.87, 379.39001, 379.39001, 379.39001, 379.91, 379.91, 379.91, 380.42999, 380.42999, 380.42999, 380.95001, 380.95001, 380.95001, 381.47, 381.47, 381.47, 381.98001, 381.98001, 381.98001, 382.5, 382.5, 382.5, 383.01001, 383.01001, 383.01001, 383.53, 383.53, 383.53, 384.04001, 384.04001, 384.04001, 384.54999, 384.54999, 384.54999, 385.07001, 385.07001, 385.07001, 385.57999, 385.57999, 385.57999, 386.09, 386.09, 386.09, 386.60001, 386.60001, 386.60001, 387.10999, 387.10999, 387.10999, 387.62, 387.62, 387.62, 388.13, 388.13, 388.13, 388.63, 388.63, 388.63, 389.14001, 389.14001, 389.14001, 389.64999, 389.64999, 389.64999, 390.14999, 390.14999, 390.14999, 388.63, 388.63, 388.63, 389.14001, 389.14001, 389.14001, 389.64999, 389.64999, 389.64999, 390.14999, 390.14999, 390.14999, 390.66, 390.66, 390.66, 391.16, 391.16, 391.16, 391.67001, 391.67001, 391.67001, 392.17001, 392.17001, 392.17001, 392.67999, 392.67999, 392.67999, 393.17999, 393.17999, 393.17999, 393.67999, 393.67999, 393.67999, 394.17999, 394.17999, 394.17999, 394.67999, 394.67999, 394.67999, 395.19, 395.19, 395.19, 395.69, 395.69, 395.69, 396.19, 396.19, 396.19, 396.69, 396.69, 396.69, 397.19, 397.19, 397.19, 397.69, 397.69, 397.69, 398.19, 398.19, 398.19, 398.69, 398.69, 398.69, 399.19, 399.19, 399.19, 399.67999, 399.67999, 399.67999, 400.17999, 400.17999, 400.17999, 400.67999, 400.67999, 400.67999, 401.17999, 401.17999, 401.17999, 401.67999, 401.67999, 401.67999, 402.17001, 402.17001, 402.17001, 402.67001, 402.67001, 402.67001, 403.17001, 403.17001, 403.17001, 403.66, 403.66, 403.66, 404.16, 404.16, 404.16, 404.66, 404.66, 404.66, 405.14999, 405.14999, 405.14999, 405.64999, 405.64999, 405.64999, 406.14999, 406.14999, 406.14999, 406.64001, 406.64001, 406.64001, 407.14001, 407.14001, 407.14001, 407.64001, 407.64001, 407.64001, 408.13, 408.13, 408.13, 408.63, 408.63, 408.63, 409.13, 409.13, 409.13, 409.62, 409.62, 409.62, 410.12, 410.12, 410.12, 410.62, 410.62, 410.62, 411.10999, 411.10999, 411.10999, 411.60999, 411.60999, 411.60999, 412.10001, 412.10001, 412.10001, 412.60001, 412.60001, 412.60001, 413.10001, 413.10001, 413.10001, 413.60001, 413.60001, 413.60001, 414.09, 414.09, 414.09, 414.59, 414.59, 414.59, 415.09, 415.09, 415.09, 415.59, 415.59, 415.59, 416.07999, 416.07999, 416.07999, 416.57999, 416.57999, 416.57999, 417.07999, 417.07999, 417.07999, 417.57999, 417.57999, 417.57999, 418.07999, 418.07999, 418.07999, 418.57999, 418.57999, 418.57999], [nan, 1.6563722836524246, 1.6403722836524246, nan, 1.6616363395359364, 1.6476363395359366, nan, 1.6542989076538939, 1.640298907653894, nan, 1.6603287796168582, 1.6463287796168584, nan, 1.6573909602141936, 1.6453909602141936, nan, 1.6501728100483295, 1.6381728100483295, nan, 1.6535630092327471, 1.6435630092327473, nan, 1.6515913680498475, 1.6415913680498477, nan, 1.649326968253007, 1.6393269682530072, nan, 1.6508723273169004, 1.6408723273169006, nan, 1.6473749873362236, 1.6373749873362238, nan, 1.6485071871004755, 1.6385071871004757, nan, 1.6462154858600102, 1.6362154858600104, nan, 1.6436834087598822, 1.6356834087598822, nan, 1.6431132715105765, 1.6351132715105765, nan, 1.6422846511661762, 1.6342846511661762, nan, 1.6398307684719318, 1.6318307684719318, nan, 1.6394408519662669, 1.6314408519662669, nan, 1.6374428509272396, 1.6294428509272396, nan, 1.6368074965992703, 1.6288074965992703, nan, 1.634211530333035, 1.626211530333035, nan, 1.633597879928187, 1.625597879928187, nan, 1.6316773015694914, 1.6236773015694914, nan, 1.6288549924331006, 1.6208549924331006, nan, 1.6261911228582016, 1.6181911228582015, nan, 1.623860370624227, 1.615860370624227, nan, 1.6226660879658288, 1.6146660879658288, nan, 1.6217483954461045, 1.6137483954461045, nan, 1.622059125989092, 1.614059125989092, nan, 1.620294733806861, 1.612294733806861, nan, 1.6204932554209357, 1.6124932554209357, nan, 1.6203255198620012, 1.6123255198620012, nan, 1.619138021497404, 1.611138021497404, nan, 1.6204105257665495, 1.6124105257665495, nan, 1.621235077199874, 1.613235077199874, nan, 1.6187912416880703, 1.6107912416880703, nan, 1.6204196882297972, 1.6124196882297972, nan, 1.6190368907017385, 1.6110368907017385, nan, 1.6184850551191468, 1.6104850551191467, nan, 1.6173228562399729, 1.6093228562399728, nan, 1.6168153905854543, 1.6088153905854543, nan, 1.6179403869979996, 1.6099403869979996, nan, 1.6171967111234533, 1.6091967111234533, nan, 1.6183159173824806, 1.6103159173824806, nan, 1.6161220874076225, 1.6081220874076225, nan, 1.6154366661699004, 1.6074366661699004, nan, 1.6134507790415067, 1.6054507790415067, nan, 1.6148839833096118, 1.6068839833096118, nan, 1.6172492163476981, 1.6072492163476984, nan, 1.617232299729947, 1.6072322997299473, nan, 1.6127321043459215, 1.6027321043459217, nan, 1.6188723793940134, 1.6088723793940136, nan, 1.6168005408009027, 1.606800540800903, nan, 1.6207486465235683, 1.6107486465235685, nan, 1.619707789685342, 1.6097077896853422, nan, 1.6192964675684907, 1.6092964675684909, nan, 1.619804272990439, 1.6098042729904392, nan, 1.6167647309822475, 1.6067647309822477, nan, 1.621132812484864, 1.6111328124848643, nan, 1.6161356911507883, 1.6041356911507882, nan, 1.618094662439775, 1.606094662439775, nan, 1.6178531546799915, 1.6058531546799915, nan, 1.620236269971587, 1.608236269971587, nan, 1.6122328837497617, 1.6002328837497617, nan, 1.6175586500151538, 1.603558650015154, nan, 1.6168228692284308, 1.6048228692284308, nan, 1.624878202410646, 1.6108782024106463, nan, 1.61579879626911, 1.6017987962691103, nan, 1.614458708765915, 1.6004587087659152, nan, 1.6347364188290658, 1.6027364188290658, nan, 1.6349092605148896, 1.6069092605148896, nan, 1.6281493452793494, 1.6021493452793496, nan, 1.6302798966697, 1.6062798966697, nan, 1.6219338276299236, 1.5999338276299238, nan, 1.6185077651242317, 1.5985077651242316, nan, 1.622655399235577, 1.6046553992355772, nan, 1.6215119347895088, 1.603511934789509, nan, 1.6168510466335868, 1.598851046633587, nan, 1.6137532268507935, 1.5977532268507935, nan, 1.6104870719133475, 1.5944870719133475, nan, 1.6108884748636345, 1.5968884748636347, nan, 1.613523559015856, 1.597523559015856, nan, 1.6030101592112505, 1.5890101592112507, nan, 1.6067312604952777, 1.592731260495278, nan, 1.605377877440321, 1.591377877440321, nan, 1.6043921540929178, 1.590392154092918, nan, 1.606589807386528, 1.594589807386528, nan, 1.6055684913350448, 1.5935684913350447, nan, 1.604943400832842, 1.5909434008328422, nan, 1.6031998900762003, 1.5891998900762005, nan, 1.6030150338732805, 1.5910150338732805, nan, 1.598930738034209, 1.5889307380342093, nan, 1.602156816544494, 1.590156816544494, nan, 1.6022182334684933, 1.5902182334684933, nan, 1.603512896681686, 1.591512896681686, nan, 1.601101996088882, 1.589101996088882, nan, 1.5993960300930927, 1.5873960300930927, nan, 1.598688229676817, 1.586688229676817, nan, 1.5963322143224217, 1.5863322143224219, nan, 1.5967530088094213, 1.5867530088094215, nan, 1.5966145385024288, 1.586614538502429, nan, 1.5964637114820217, 1.586463711482022, nan, 1.5928221602705457, 1.582822160270546, nan, 1.5978834293750266, 1.5878834293750268, nan, 1.5965729711917385, 1.5865729711917387, nan, 1.592309104722474, 1.5823091047224742, nan, 1.596811203896316, 1.5868112038963162, nan, 1.5931066262119133, 1.5831066262119136, nan, 1.590965267353939, 1.578965267353939, nan, 1.5964289179893894, 1.5864289179893896, nan, 1.5919117373724219, 1.581911737372422, nan, 1.5867310651422228, 1.576731065142223, nan, 1.5946590769172397, 1.5826590769172397, nan, 1.5899680475176061, 1.5799680475176063, nan, 1.592099454232746, 1.580099454232746, nan, 1.587195601241917, 1.575195601241917, nan, 1.5914707251659344, 1.5794707251659343, nan, 1.5925012245981702, 1.5805012245981702, nan, 1.5898978086861526, 1.5778978086861526, nan, 1.591800751487047, 1.5778007514870471, nan, 1.5918505559733815, 1.5778505559733818, nan, 1.5927486239152706, 1.5787486239152708, nan, 1.5925918165373358, 1.578591816537336, nan, 1.5880404634087084, 1.5740404634087086, nan, 1.5931743649291072, 1.5771743649291072, nan, 1.5939104770394237, 1.5779104770394237, nan, 1.5903664432736304, 1.5743664432736304, nan, 1.5882071958230994, 1.5702071958230996, nan, 1.5995304673682158, 1.581530467368216, nan, 1.5970072549949592, 1.5770072549949592]}, {[353.79999, 354.37, 354.94, 355.51001, 356.07999, 356.64999, 357.22, 357.78, 358.35001, 358.91, 359.47, 360.03, 360.59, 361.14999, 361.70001, 362.26001, 362.81, 363.35999, 363.91, 364.45999, 365.01001, 365.56, 366.10001, 366.64999, 367.19, 376.78, 378.87, 379.39001, 379.91, 380.42999, 380.95001, 381.47, 381.98001, 382.5, 383.01001, 383.53, 384.04001, 384.54999, 385.07001, 385.57999, 386.09, 386.60001, 387.10999, 387.62, 388.13, 388.63, 389.14001, 389.64999, 390.14999, 388.63, 389.14001, 389.64999, 390.14999, 390.66, 391.16, 391.67001, 392.17001, 392.67999, 393.17999, 393.67999, 394.17999, 394.67999, 395.19, 395.69, 396.19, 396.69, 397.19, 397.69, 398.19, 398.69, 399.19, 399.67999, 400.17999, 400.67999, 401.17999, 401.67999, 402.17001, 402.67001, 403.17001, 403.66, 404.16, 404.66, 405.14999, 405.64999, 406.14999, 406.64001, 407.14001, 407.64001, 408.13, 408.63, 409.13, 409.62, 410.12, 410.62, 411.10999, 411.60999, 412.10001, 412.60001, 413.10001, 413.60001, 414.09, 414.59, 415.09, 415.59, 416.07999, 416.57999, 417.07999, 417.57999, 418.07999, 418.57999], [1.6483722836524246, 1.6546363395359365, 1.647298907653894, 1.6533287796168583, 1.6513909602141936, 1.6441728100483295, 1.6485630092327472, 1.6465913680498476, 1.644326968253007, 1.6458723273169005, 1.6423749873362237, 1.6435071871004756, 1.6412154858600103, 1.6396834087598822, 1.6391132715105765, 1.6382846511661762, 1.6358307684719318, 1.6354408519662669, 1.6334428509272396, 1.6328074965992703, 1.630211530333035, 1.629597879928187, 1.6276773015694914, 1.6248549924331006, 1.6221911228582016, 1.6131967111234533, 1.6094507790415067, 1.6108839833096118, 1.6122492163476982, 1.6122322997299472, 1.6077321043459216, 1.6138723793940135, 1.6118005408009028, 1.6157486465235684, 1.6147077896853421, 1.6142964675684908, 1.614804272990439, 1.6117647309822476, 1.6161328124848642, 1.6101356911507883, 1.612094662439775, 1.6118531546799915, 1.614236269971587, 1.6062328837497617, 1.6105586500151539, 1.6108228692284308, 1.6178782024106462, 1.6087987962691102, 1.6074587087659151, 1.6187364188290658, 1.6209092605148896, 1.6151493452793495, 1.6182798966697, 1.6109338276299237, 1.6085077651242317, 1.613655399235577, 1.612511934789509, 1.607851046633587, 1.6057532268507935, 1.6024870719133475, 1.6038884748636346, 1.605523559015856, 1.5960101592112506, 1.5997312604952778, 1.598377877440321, 1.597392154092918, 1.600589807386528, 1.5995684913350448, 1.5979434008328421, 1.5961998900762004, 1.5970150338732805, 1.5939307380342091, 1.596156816544494, 1.5962182334684933, 1.597512896681686, 1.595101996088882, 1.5933960300930927, 1.592688229676817, 1.5913322143224218, 1.5917530088094214, 1.591614538502429, 1.5914637114820218, 1.5878221602705458, 1.5928834293750267, 1.5915729711917386, 1.587309104722474, 1.5918112038963161, 1.5881066262119135, 1.584965267353939, 1.5914289179893895, 1.586911737372422, 1.581731065142223, 1.5886590769172397, 1.5849680475176062, 1.586099454232746, 1.581195601241917, 1.5854707251659343, 1.5865012245981702, 1.5838978086861526, 1.584800751487047, 1.5848505559733816, 1.5857486239152707, 1.585591816537336, 1.5810404634087085, 1.5851743649291072, 1.5859104770394237, 1.5823664432736304, 1.5792071958230995, 1.590530467368216, 1.5870072549949592]}] ("Real Part vs wavelength")
  n1 = call <vilib>:"Add State(s) to Queue__jki_lib_state_machine.vi"("State(s) in (\"\")"="Macro: Initialize") -> ("States Out"=w2:string)  [unwired: 14 in]
  n2 = while "JKI - String-Based Queued State Machine (Basic) v1.0" {
    shift-right: [w6] -> _
    shift-left: _ -> [w5]
    shift-right: [w9] -> _
    shift-left: _ -> [w3]
    shift-right: [w8] -> _
    shift-left: w2 -> [w10]
    stop <- w7 stop-if-true
    w4 = -1  # Timeout
    # "Template Copyright © 2008 JKI - http://jkisoft.com/state-machine"
    n3 = call <vilib>:"Parse State Queue__jki_lib_state_machine.vi"("State Queue"=w10, "Error In (no error)"=w3) -> ("Remaining States"=w12:string, "Current State"=w13:string, "Arguments"=w11:string)  [unwired: 11 in]
    n4 = case shown="\"\", \"Idle\"" w13 {
      selector: w13 -> [_ _ w158 _ _ _ _ _ _ _ _ _ _ _ _ _ _ _ _ _ _ _ _ _ _ _ _ _ _ _]
      tunnel: w12 -> [w20 w157 w162 w180 w186 w191 w195 w209 w215 w219 w224 w230 w241 w267 w272 w282 w286 w308 w346 w360 w367 w420 w467 w593 w661 w740 w810 w912 w1064 w1142]
      tunnel: w11 -> [_ _ _ _ _ _ _ _ _ _ _ w225 w235 _ _ _ _ w289 _ _ w361 _ _ _ _ _ _ _ _ _]
      tunnel: w5 -> [w18 w154 w160 w171 w183 w189 w192 _ w210 w216 w222 w228 w237 w264 w269 w279 w283 w293 w343 w357 w364 w417 w464 w591 w659 w738 w782 w887 w1061 w1100]
      tunnel: [w17 w155 w164 w177 errorcluster {"status"=FALSE, "code"=0, "source"=""} ("error out") w188 w193 w206 w211 w217 w221 w226 w238 w265 w270 w280 w284 w306 w344 w358 w365 w418 w465 w590 w658 w737 w808 w910 w1062 w1140] -> w9
      tunnel: w3 -> [w16 w155 w163 w177 w182 w188 w193 w206 w212 w217 w221 w227 w239 w265 w270 w280 w284 w306 w344 w358 w365 w418 w465 w590 w658 w737 w808 w910 w1062 w1140]
      tunnel: [w19 w156 w161 w179 w185 w190 w194 w208 w214 w218 w223 w229 w240 w266 w271 w281 w285 w307 w345 w359 w366 w419 w466 w592 w660 w739 w809 w911 w1063 w1141] -> w8
      tunnel: [_ _ _ _ _ TRUE _ _ _ _ _ _ _ _ _ _ _ _ _ _ _ _ _ _ _ _ _ _ _ _] -> w7
      tunnel: [w15 w154 w160 w178 w183 w189 w192 w207 w210 w216 w222 w228 w237 w264 w269 w279 w283 w305 w343 w356 w363 w416 w463 w591 w659 w738 w781 w886 w1061 w1099] -> w6
      tunnel: w4 -> [w14 _ _ _ _ _ _ _ _ _ _ _ _ _ _ _ _ _ _ _ _ _ _ _ _ _ _ _ _ _]
      frame "", "Idle" {
        # "executes when the state queue is empty"
        n5 = event shown="[18] \"Calculate Errors\": Value Change" {
          selector: _ -> [_ _ _ _ _ _ _ _ _ _ _ _ _ _ _ _ _ _ _ _]
          dyn-events: _ -> [_ _ _ _ _ _ _ _ _ _ _ _ _ _ _ _ _ _ _ _]
          timeout: w14 -> [_ _ _ _ _ _ _ _ _ _ _ _ _ _ _ _ _ _ _ _]
          tunnel: w20 -> [w24 w33 w53 w59 w65 w71 w76 w84 w90 w95 w100 w105 w110 w115 w120 w125 w132 w139 w147 w153]
          tunnel: [w23 w32 w52 w58 w64 w70 w75 w83 w89 w94 w99 w104 w109 w114 w119 w124 w131 w138 w146 w152] -> w19
          tunnel: w18 -> [w21 w30 w50 w56 w62 w68 w73 w81 w87 w92 w97 w102 w107 w112 w117 w122 w127 w134 w144 w150]
          tunnel: [w22 w31 w51 w57 w63 w69 w74 w82 w88 w93 w98 w103 w108 w113 w118 w123 w130 w137 w145 w151] -> w17
          tunnel: w16 -> [w22 w31 w51 w57 w63 w69 w74 w82 w88 w93 w98 w103 w108 w113 w118 w123 w130 w137 w145 w151]
          tunnel: [w21 w30 w50 w56 w62 w68 w73 w81 w87 w92 w97 w102 w107 w112 w117 w122 w126 w133 w144 w150] -> w15
          event Timeout {
            # "Timeout Frame\n(this will only execute if the Event Structure timeout is >= 0)"
            n6 = event-data() -> ()  [unwired: 1 in, 1 out]
            n7 = call <vilib>:"Add State(s) to Queue__jki_lib_state_machine.vi"("State(s) in (\"\")"=w24) -> ("States Out"=w23:string)  [unwired: 14 in]
          }
          event "Diameters to fit": Mouse Down {
            # "Timeout Frame\n(this will only execute if the Event Structure timeout is >= 0)"
            n8 = event-data() -> ("Coords"=w29:T12)  [unwired: 1 in, 7 out]
            n9 = case shown="True" "Quick Fit" {
              tunnel: ["" w36] -> w25
              frame False {
              }
              frame True {
                n10 = local read "Use Factors"() -> (w35:bool)
                n11 = Select(t="Load Files >> Dont Initialize Sizes\nRetrieve RI >> UseFactors", s=w35, f="Load Files >> Dont Initialize Sizes\nRetrieve RI >> DontUseFactors") -> (s? t:f=w36:string)
                n12 = case shown="True" w35 {
                  frame False {
                  }
                  frame True {
                    n13 = One Button Dialog(message="You are using Extinction factor and Diameter factors/offset in this calculation !!") -> ()  [unwired: 1 in, 1 out]
                  }
                }
              }
            }
            n14 = invoke on="Diameters to fit" class="LstBox (strict)" method="Point To Row"("Point"=w29) -> ("Row"=w28:i32, "InGlyph"=w27:bool)  [unwired: 6 in, 5 out]
            n15 = case shown="True" w27 {
              tunnel: w28 -> [_ w47]
              frame False {
              }
              frame True {
                w43 = 37 ("Item Symbols")
                n16 = property on="Diameters to fit" class="LstBox (strict)"() -> ("Item Symbols"=w40:i32[])  [unwired: 2 in, 2 out]
                n17 = Index Array(array=w40, index=w47) -> (element=w46:i32)
                n18 = Equal?(x=w46, y=w43) -> (x = y?=w45:bool)
                n19 = Select(t=38 ("Item Symbols"), s=w45, f=w43) -> (s? t:f=w44:i32)
                n20 = Replace Array Subset(array=w40, new element=w44, index=w47) -> (w41:i32[])
                n21 = property on="Diameters to fit" class="LstBox (strict)"("Item Symbols"=w41) -> ()  [unwired: 2 in, 2 out]
              }
            }
            n22 = call <vilib>:"Add State(s) to Queue__jki_lib_state_machine.vi"("State(s) in Front (\"\")"=w25, "State(s) in (\"\")"=w33) -> ("States Out"=w32:string)  [unwired: 13 in]
          }
          event "Diamter Offset Radio Button": Mouse Up {
            w48 = TRUE ("Diamter Offset Radio Button")
            # "Timeout Frame\n(this will only execute if the Event Structure timeout is >= 0)"
            n23 = event-data() -> ()  [unwired: 1 in, 8 out]
            n24 = local write "Diamter Offset Radio Button"(w48) -> ()
            n25 = local write "Diameter Factor Radio Button"(FALSE ("Diameter Factor Radio Button")) -> ()
            n26 = local write "Diameter Factor or Offset"(w48) -> ()
            n27 = call <vilib>:"Add State(s) to Queue__jki_lib_state_machine.vi"("State(s) in (\"\")"=w53) -> ("States Out"=w52:string)  [unwired: 14 in]
          }
          event "Diameter Factor Radio Button": Mouse Up {
            w54 = FALSE ("Diamter Offset Radio Button")
            # "Timeout Frame\n(this will only execute if the Event Structure timeout is >= 0)"
            n28 = event-data() -> ()  [unwired: 1 in, 8 out]
            n29 = local write "Diamter Offset Radio Button"(w54) -> ()
            n30 = local write "Diameter Factor Radio Button"(TRUE ("Diameter Factor Radio Button")) -> ()
            n31 = local write "Diameter Factor or Offset"(w54) -> ()
            n32 = call <vilib>:"Add State(s) to Queue__jki_lib_state_machine.vi"("State(s) in (\"\")"=w59) -> ("States Out"=w58:string)  [unwired: 14 in]
          }
          event "Imaginary Part vs wavelength": Cursor Move {
            # "Timeout Frame\n(this will only execute if the Event Structure timeout is >= 0)"
            n33 = event-data() -> ()  [unwired: 1 in, 9 out]
            n34 = property on="Imaginary Part vs wavelength" class="XYGraph (strict)"() -> ("Cursor.Cursor X"=w61:dbl)  [unwired: 2 in, 2 out]
            n35 = property on="Real Part vs wavelength" class="XYGraph (strict)"("Cursor.Cursor X"=w61) -> ()  [unwired: 2 in, 2 out]
            n36 = call <vilib>:"Add State(s) to Queue__jki_lib_state_machine.vi"("State(s) in Front (\"\")"="Update Corrected multiple charge extinction graph" ("State(s) in Front (\"\")"), "State(s) in (\"\")"=w65) -> ("States Out"=w64:string)  [unwired: 13 in]
          }
          event "Real Part vs wavelength": Cursor Move {
            n37 = event-data() -> ()  [unwired: 1 in, 9 out]
            n38 = property on="Real Part vs wavelength" class="XYGraph (strict)"() -> ("Cursor.Cursor X"=w67:dbl)  [unwired: 2 in, 2 out]
            n39 = property on="Imaginary Part vs wavelength" class="XYGraph (strict)"("Cursor.Cursor X"=w67) -> ()  [unwired: 2 in, 2 out]
            n40 = call <vilib>:"Add State(s) to Queue__jki_lib_state_machine.vi"("State(s) in Front (\"\")"="Update Corrected multiple charge extinction graph" ("State(s) in Front (\"\")"), "State(s) in (\"\")"=w71) -> ("States Out"=w70:string)  [unwired: 13 in]
          }
          event "OK": Value Change {
            # "Exit Button Value Change (pressed) Event\n(this executes Macro: Exit to terminate the VI)"
            n41 = event-data() -> ()  [unwired: 1 in, 1 out]
            n42 = call <vilib>:"Add State(s) to Queue__jki_lib_state_machine.vi"("State(s) in Front (\"\")"="Macro: Exit", "State(s) in (\"\")"=w76) -> ("States Out"=w75:string)  [unwired: 13 in]
          }
          event "Retrieve RI": Value Change {
            # "Exit Button Value Change (pressed) Event\n(this executes Macro: Exit to terminate the VI)"
            n43 = event-data() -> ()  [unwired: 1 in, 6 out]
            n44 = Select(t="Load Files >> Dont Initialize Sizes\nRetrieve RI >> UseFactors", s="Use Factors", f="Load Files >> Dont Initialize Sizes\nRetrieve RI >> DontUseFactors") -> (s? t:f=w80:string)
            n45 = case shown="False" "Use Factors" {
              frame False {
              }
              frame True {
                n46 = One Button Dialog(message="You are using Extinction factor and Diameter factors/offset in this calculation !!") -> ()  [unwired: 1 in, 1 out]
              }
            }
            n47 = call <vilib>:"Add State(s) to Queue__jki_lib_state_machine.vi"("State(s) in Front (\"\")"=w80, "State(s) in (\"\")"=w84) -> ("States Out"=w83:string)  [unwired: 13 in]
          }
          event "Retrieve RI Calculate lines seperately": Value Change {
            # "Exit Button Value Change (pressed) Event\n(this executes Macro: Exit to terminate the VI)"
            n48 = event-data() -> ()  [unwired: 1 in, 6 out]
            n49 = call <vilib>:"Add State(s) to Queue__jki_lib_state_machine.vi"("State(s) in Front (\"\")"="Load Files MC\nRetrieve RI", "State(s) in (\"\")"=w90) -> ("States Out"=w89:string)  [unwired: 13 in]
          }
          event "Retrieve RI without taking the mean (MC)": Value Change {
            # "Exit Button Value Change (pressed) Event\n(this executes Macro: Exit to terminate the VI)"
            n50 = event-data() -> ()  [unwired: 1 in, 6 out]
            n51 = call <vilib>:"Add State(s) to Queue__jki_lib_state_machine.vi"("State(s) in Front (\"\")"="Load Files MC\nRetreive RI from Single Measurements(MC)", "State(s) in (\"\")"=w95) -> ("States Out"=w94:string)  [unwired: 13 in]
          }
          event "Save RI": Value Change {
            # "Exit Button Value Change (pressed) Event\n(this executes Macro: Exit to terminate the VI)"
            n52 = event-data() -> ()  [unwired: 1 in, 6 out]
            n53 = call <vilib>:"Add State(s) to Queue__jki_lib_state_machine.vi"("State(s) in Front (\"\")"="Save RI to file", "State(s) in (\"\")"=w100) -> ("States Out"=w99:string)  [unwired: 13 in]
          }
          event "Save RI expanded Edition": Value Change {
            # "Exit Button Value Change (pressed) Event\n(this executes Macro: Exit to terminate the VI)"
            n54 = event-data() -> ()  [unwired: 1 in, 6 out]
            n55 = call <vilib>:"Add State(s) to Queue__jki_lib_state_machine.vi"("State(s) in Front (\"\")"="Save RI to File Expanded Edition", "State(s) in (\"\")"=w105) -> ("States Out"=w104:string)  [unwired: 13 in]
          }
          event "Find Extinction Factor Graph": Value Change {
            # "Exit Button Value Change (pressed) Event\n(this executes Macro: Exit to terminate the VI)"
            n56 = event-data() -> ()  [unwired: 1 in, 6 out]
            n57 = call <vilib>:"Add State(s) to Queue__jki_lib_state_machine.vi"("State(s) in Front (\"\")"="Load Files >> Dont Initialize Sizes\nFind Extinction Factor", "State(s) in (\"\")"=w110) -> ("States Out"=w109:string)  [unwired: 13 in]
          }
          event "Plot RI": Value Change {
            # "Exit Button Value Change (pressed) Event\n(this executes Macro: Exit to terminate the VI)"
            n58 = event-data() -> ()  [unwired: 1 in, 6 out]
            n59 = call <vilib>:"Add State(s) to Queue__jki_lib_state_machine.vi"("State(s) in Front (\"\")"="Append Mie Curve", "State(s) in (\"\")"=w115) -> ("States Out"=w114:string)  [unwired: 13 in]
          }
          event "Save RI MC": Value Change {
            # "Exit Button Value Change (pressed) Event\n(this executes Macro: Exit to terminate the VI)"
            n60 = event-data() -> ()  [unwired: 1 in, 6 out]
            n61 = call <vilib>:"Add State(s) to Queue__jki_lib_state_machine.vi"("State(s) in Front (\"\")"="Save RI -Monte Carlo to file", "State(s) in (\"\")"=w120) -> ("States Out"=w119:string)  [unwired: 13 in]
          }
          event "Retrieve RI (MC)": Value Change {
            # "Exit Button Value Change (pressed) Event\n(this executes Macro: Exit to terminate the VI)"
            n62 = event-data() -> ()  [unwired: 1 in, 6 out]
            n63 = call <vilib>:"Add State(s) to Queue__jki_lib_state_machine.vi"("State(s) in Front (\"\")"="Load Files\nRetrieve RI Monte Carlo", "State(s) in (\"\")"=w125) -> ("States Out"=w124:string)  [unwired: 13 in]
          }
          event "Extinction Cross Section File": Value Change {
            # "Exit Button Value Change (pressed) Event\n(this executes Macro: Exit to terminate the VI)"
            n64 = event-data() -> ()  [unwired: 1 in, 6 out]
            n65 = local read "Extinction Cross Section File"() -> (w128:path)
            n66 = Bundle By Name(cluster=w127, "Extinction Cross section Path"=w128) -> (w126:T14)
            n67 = call <vilib>:"Add State(s) to Queue__jki_lib_state_machine.vi"("State(s) in Front (\"\")"="Load Files >> Initialize Sizes\nUpdate Window after Load Files", "State(s) in (\"\")"=w132) -> ("States Out"=w131:string)  [unwired: 13 in]
          }
          event "Mutiple Charge Data File": Value Change {
            # "Exit Button Value Change (pressed) Event\n(this executes Macro: Exit to terminate the VI)"
            n68 = event-data() -> ()  [unwired: 1 in, 6 out]
            n69 = local read "Mutiple Charge Data File"() -> (w135:path)
            n70 = Bundle By Name(cluster=w134, "Multiple charge correction file Path"=w135) -> (w133:T14)
            n71 = call <vilib>:"Add State(s) to Queue__jki_lib_state_machine.vi"("State(s) in Front (\"\")"="Load Files\nUpdate Window after Load Files", "State(s) in (\"\")"=w139) -> ("States Out"=w138:string)  [unwired: 13 in]
          }
          event "Calculate Errors": Value Change {
            # "Exit Button Value Change (pressed) Event\n(this executes Macro: Exit to terminate the VI)"
            n72 = event-data() -> ("NewVal"=w143:bool)  [unwired: 1 in, 5 out]
            n73 = Select(t=FALSE, s=w143, f=FALSE) -> (s? t:f=w141:bool)
            n74 = property on="Approximate Errors" class="Bool (strict)"("Visible"=w143) -> ()  [unwired: 2 in, 2 out]
            n75 = property on="Approximate Errors" class="Bool (strict)"("Value"=w141) -> ()  [unwired: 2 in, 2 out]
            n76 = call <vilib>:"Add State(s) to Queue__jki_lib_state_machine.vi"("State(s) in (\"\")"=w147) -> ("States Out"=w146:string)  [unwired: 14 in]
          }
          event Panel Close? {
            # "Discard the event because we'll close the front panel ourselves in Macro: Exit"
            # "Close Panel button (pressed) Event\n(this executes Macro: Exit to terminate the VI)"
            n77 = event-data() -> ()  [unwired: 1 in, 1 out]
            n78 = call <vilib>:"Add State(s) to Queue__jki_lib_state_machine.vi"("State(s) in Front (\"\")"="Macro: Exit", "State(s) in (\"\")"=w153) -> ("States Out"=w152:string)  [unwired: 13 in]
            n79 = event-data("Discard?"=TRUE) -> ()  [unwired: 1 in, 1 out]
          }
        }
      }
      frame "---------- Core ----------" {
        # "Do not put any code in this frame.\n(it is a separator no-op)"
        n80 = call <vilib>:"Add State(s) to Queue__jki_lib_state_machine.vi"("State(s) in (\"\")"=w157) -> ("States Out"=w156:string)  [unwired: 14 in]
      }
      frame Default {
        w167 = 42 items=["No error", "Argument error", "Memory is full", "Out of zone", "End of file", "File already open", "Generic file I/O error", "File not found", "File permission error", "Disk is full", "Duplicate path", "Too many files open", "System feature not enabled", "Resource file not found", "Cannot add resource", "Resource not found", "Image not found", "Image memory error", "Pen does not exist", "Config type invalid", "Config token not found", "Config parse error", "Config memory error", "Bad external code format", "Bad external code offset", "External code not present", "Null window", "Destroy window error", "Null menu", "Print aborted", "Bad print record", "Print driver error", "Windows error during printing", "Memory error during printing", "Print dialog error", "Generic print error", "Invalid device refnum", "Device not found", "Device parameter error", "Device unit error", "Cannot open device", "Device call aborted", "Generic error", "Cancelled by user", "Object ID too low", "Object ID too high", "Object not in heap", "Unknown heap", "Unknown object (invalid DefProc)", "Unknown object (DefProc not in table)", "Message out of range", "Invalid (null) method", "Unknown message", "Manager call not supported", "Bad address", "Network operation in progress", "Network operation timed out", "Connection is busy", "Network attribute not supported", "Network error", "Address in use", "System out of memory", "Connection aborted", "Connection refused", "Not connected", "Already connected", "Connection closed", "Initialization error (interapplication manager)", "Bad occurrence", "Wait on unbound occurrence handler", "Occurrence queue overflow", "Datalog type conflict", "Unused", "Unrecognized type (interapplication manager)", "Memory corrupt", "Failed to make temporary DLL", "Old CIN version", "Drag socket not found", "Failed to load drop-object", "Failed to register OLE object", "Failed to release OLE object", "Format specifier type mismatch", "Unknown format specifier", "Too few format specifiers", "Too many format specifiers", "Scan failed", "Newer CIN version", "Error converting to variant", "Runtime menu error", "Password tampered", "Variant attribute not found", "Incompatible variant data type", "Event data is not available", "Event Store is not present", "Occurrence is not found", "Event Queue is not created", "Event info is not available", "Refnum passed is NULL", "Error retrieving Class GUID", "Error retrieving CoClass GUID", "Error retrieving TypeLib GUID.", "Bad built application magic bytes.", "Specific driver is different from the specific driver associated with the Logical Name.", "There is no session opened to the class driver.", "Max Error", "MAX - Error with config objects", "MAX - Error loading configuration", "MAX - Group not supported"]
        # "Current State"
        # "Do not delete, rename, or modify this frame.\n(this is used to capture unhandled states and typos)"
        # "Handle mistyped state name (developer tool)"
        n81 = call <vilib>:"Add State(s) to Queue__jki_lib_state_machine.vi"("State(s) in (\"\")"=w162) -> ("States Out"=w161:string)  [unwired: 14 in]
        n82 = Format Into String(format string="Software Exception: Unhandled State \"%s\"." ("message"), error in=w163, w158) -> (resulting string=w166:string, error out=w165:errorcluster)  [unwired: 1 in]
        n83 = call <vilib>:"Error Cluster From Error Code.vi"("show call chain? (False)"=TRUE, "error in (no error)"=w165, "error message (\"\")"=w166, "error code (0)"=w167) -> ("error out"=w164:errorcluster)  [unwired: 5 in]
      }
      frame "Initialize Core Data" {
        # "Do not delete, rename, or modify this frame.\n(this is used to determine panel behavior on exit)"
        # "originally closed?"
        # "exe?"
        # "If panel starts closed or is an EXE, then close it when we exit"
        n84 = call <vilib>:"Add State(s) to Queue__jki_lib_state_machine.vi"("State(s) in (\"\")"=w180) -> ("States Out"=w179:string)  [unwired: 14 in]
        n85 = property class="App"() -> ("App.Kind"=w175:T9)  [unwired: 2 in, 2 out]
        n86 = property class="VI"() -> ("Front Panel.Open"=w176:bool)  [unwired: 2 in, 2 out]
        n87 = Equal?(x=w175, y=T9."Run Time System" ("Application:Kind")) -> (x = y?=w172:bool)
        n88 = Not(x=w176) -> (.not. x?=w173:bool)
        n89 = Or(x=w173, y=w172) -> (x .or. y?=w170:bool)
        n90 = control-ref of="Current VI Reference"() -> (w169:refnum<vi>)
        n91 = Bundle By Name(cluster=w171, "Core.Current VI Reference"=w169, "Core.Close Panel on Exit?"=w170) -> (w178:T14)
      }
      frame "Error Handler" {
        # "Unhandled Error -- Display it"
        # "Handle any errors here.\nYou can also output any states to clean-up after errors occur"
        # "Clear error"
        n92 = call <vilib>:"General Error Handler.vi"("error in (no error)"=w182) -> ()  [unwired: 10 in, 5 out]
        n93 = call <vilib>:"Add State(s) to Queue__jki_lib_state_machine.vi"("State(s) in Front (\"\")"="/* Post Error States", "State(s) in (\"\")"=w186) -> ("States Out"=w185:string)  [unwired: 13 in]
      }
      frame "Exit" {
        # "Do not put any code in this frame.\n(No errors that occur here will be handled.)"
        n94 = call <vilib>:"Add State(s) to Queue__jki_lib_state_machine.vi"("State(s) in (\"\")"=w191) -> ("States Out"=w190:string)  [unwired: 14 in]
      }
      frame "---------- Data ----------" {
        # "Do not put any code in this frame.\n(It is a separator no-op. You can make a copy of this frame to create a new Data frame)"
        n95 = call <vilib>:"Add State(s) to Queue__jki_lib_state_machine.vi"("State(s) in (\"\")"=w195) -> ("States Out"=w194:string)  [unwired: 14 in]
      }
      frame "Data: Initialize" {
        w197 = 0  # NumberOfMeasurementsperSize
        w198 = dbl[][] []  # FullExtinctionData
        w199 = path ""  # Multiple charge correction file Path
        w200 = path ""  # Extinction Cross section Path
        w201 = T13 {"Real RI"=[], "Imaginary RI"=[], "Std Imaginary RI"=[], "Std Real RI"=[], "Wavelength"=[], "Residue"=[], "Extinction Factor"=[], "Diameter Factor"=[], "Diameter Offset"=[], "Best fit result"=[], "Normalized Residuals"=[]}  # RI MC results
        w202 = T13 {"Real RI"=[], "Imaginary RI"=[], "Std Imaginary RI"=[], "Std Real RI"=[], "Wavelength"=[], "Residue"=[], "Extinction Factor"=[], "Diameter Factor"=[], "Diameter Offset"=[], "Best fit result"=[], "Normalized Residuals"=[]}  # RI results
        w203 = T6 {"SMPS Sizes"=[], "Concentration"=[], "Double Charge Correction Flag"=FALSE}  # Particle Distribution Data
        w204 = T5 {"Extinction"=[], "Extinction Uncertainty"=[], "Size parameters"=[], "Number ofSizes"=0.0, "GeometricCrossSection"=[], "WaveLength"=[], "Sizes"=[]}  # Extinction ExtinctionUncertainity Size parameter and Number ofS sizes
        w205 = T15 {"Current VI Reference"=refnum, "Close Panel on Exit?"=FALSE}  # Core
        # "do not delete - used by framework"
        # "Data names and types of shift register data are defined by this bundle."
        # "Initialize the shift-register data, here.\n(data names are defined by what you wire into the bundle function)"
        n96 = call <vilib>:"Add State(s) to Queue__jki_lib_state_machine.vi"("State(s) in (\"\")"=w209) -> ("States Out"=w208:string)  [unwired: 14 in]
        n97 = Bundle("Core"=w205, "Extinction ExtinctionUncertainity Size parameter and Number ofS sizes"=w204, "Particle Distribution Data"=w203, "RI results"=w202, "RI MC results"=w201, "Extinction Cross section Path"=w200, "Multiple charge correction file Path"=w199, "FullExtinctionData"=w198, "NumberOfMeasurementsperSize"=w197, "Baes data type definition"="Baes data type definition") -> (w207:T14)  [unwired: 1 in]
      }
      frame "Data: Cleanup" {
        # "Cleanup any data and references, here.\n(this is called automatically, by the Macro: Exit)"
        n98 = Unbundle By Name(w210) -> ("Core.Current VI Reference"=w213:refnum<vi>)
        n99 = call <vilib>:"Add State(s) to Queue__jki_lib_state_machine.vi"("State(s) in (\"\")"=w215) -> ("States Out"=w214:string)  [unwired: 14 in]
        n100 = Close Reference(reference=w213, error in (no error)=w212) -> (error out=w211:errorcluster)
      }
      frame "---------- UI ----------" {
        # "Do not put any code in this frame.\n(It is a separator no-op. You can make a copy of this frame to create a new UI frame)"
        n101 = call <vilib>:"Add State(s) to Queue__jki_lib_state_machine.vi"("State(s) in (\"\")"=w219) -> ("States Out"=w218:string)  [unwired: 14 in]
      }
      frame "UI: Initialize" {
        # "Initialize the User Interface, here.\n(this is called automatically, by the Macro: Init)"
        n102 = call <vilib>:"Add State(s) to Queue__jki_lib_state_machine.vi"("State(s) in (\"\")"=w224) -> ("States Out"=w223:string)  [unwired: 14 in]
        n103 = property on="Retrieve RI" class="Bool"("BoolText.Text"="Retrieve RI" ("Boolean Text.Text")) -> ()  [unwired: 2 in, 2 out]
      }
      frame "UI: Cursor Set" {
        # "Argument"
        # "Set and Unset Cursor Busy.\n(Usage: \"UI: Cursor Set >> Busy|Idle\")"
        n104 = call <vilib>:"Add State(s) to Queue__jki_lib_state_machine.vi"("State(s) in (\"\")"=w230) -> ("States Out"=w229:string)  [unwired: 14 in]
        n105 = case shown="\"Idle\", Default" w225 {
          tunnel: w227 -> [w232 w234]
          tunnel: [w231 w233] -> w226
          frame "Idle", Default {
            n106 = call <vilib>:"Unset Busy.vi"("error in (no error)"=w232) -> ("error out"=w231:errorcluster)  [unwired: 10 in]
          }
          frame "Busy" {
            n107 = call <vilib>:"Set Busy.vi"("error in (no error)"=w234) -> ("error out"=w233:errorcluster)  [unwired: 9 in, 1 out]
          }
        }
      }
      frame "UI: Front Panel State" {
        # "Argument"
        # "Set Front Panel Open or Closed\n(Usage: \"UI: Front Panel State >> Open|Close\")"
        n108 = Unbundle By Name(w237) -> ("Core.Current VI Reference"=w236:refnum<vi>)
        n109 = call <vilib>:"Add State(s) to Queue__jki_lib_state_machine.vi"("State(s) in (\"\")"=w241) -> ("States Out"=w240:string)  [unwired: 14 in]
        n110 = case shown="\"Open\", Default" w235 {
          tunnel: w239 -> [w245 w258]
          tunnel: [w247 w259] -> w238
          tunnel: w236 -> [w246 w256]
          frame "Open", Default {
            n111 = property class="VI"(reference=w246, error in=w245) -> (reference out=w243:refnum<vi>, error out=w244:errorcluster, "Front Panel.Open"=w242:bool)
            n112 = case shown="False" w242 {
              tunnel: [w250 w253] -> w247
              tunnel: w244 -> [w249 w253]
              tunnel: w243 -> [w248 _]
              frame False {
                n113 = invoke class="VI" method="FP.Open"(reference=w248, error in=w249, "Activate"=TRUE, "State"=T10."Standard") -> (error out=w250:errorcluster)  [unwired: 1 in, 4 out]
              }
              frame True {
              }
            }
          }
          frame "Close" {
            n114 = property class="VI"(reference=w256, error in=w258) -> (reference out=w255:refnum<vi>, error out=w257:errorcluster, "Front Panel.Open"=w254:bool)
            n115 = case shown="True" w254 {
              tunnel: [w260 w263] -> w259
              tunnel: w257 -> [w260 w262]
              tunnel: w255 -> [_ w261]
              frame False {
              }
              frame True {
                n116 = invoke class="VI" method="FP.Close"(reference=w261, error in=w262) -> (error out=w263:errorcluster)  [unwired: 1 in, 2 out]
              }
            }
          }
        }
      }
      frame "---------- Macro ----------" {
        # "Do not put any code in this frame.\n(It is a separator no-op. You can make a copy of this frame to create a new Macro frame)"
        n117 = call <vilib>:"Add State(s) to Queue__jki_lib_state_machine.vi"("State(s) in (\"\")"=w267) -> ("States Out"=w266:string)  [unwired: 14 in]
      }
      frame "Macro: Initialize" {
        w268 = "Data: Initialize\nInitialize Core Data\nUI: Initialize\nUI: Front Panel State >> Open"  # Data: Initialize Initialize Core Data UI: Initialize UI: Front Panel State >> Open
        # "Initialization Macro\n(This is called once, when the VI starts)"
        n118 = call <vilib>:"Add State(s) to Queue__jki_lib_state_machine.vi"("State(s) in Front (\"\")"=w268, "State(s) in (\"\")"=w272) -> ("States Out"=w271:string)  [unwired: 13 in]
      }
      frame "Macro: Exit" {
        # "Exit Macro\n(This is called once, when the VI exits)"
        n119 = Unbundle By Name(w279) -> ("Core.Close Panel on Exit?"=w278:bool)
        n120 = Select(t="UI: Front Panel State >> Close", s=w278, f="") -> (s? t:f=w275:string)
        n121 = call <vilib>:"Add State(s) to Queue__jki_lib_state_machine.vi"("State(s) in (\"\")"=w275, "State(s) at Back (\"\")"="Data: Cleanup\nExit") -> ("States Out"=w273:string)  [unwired: 13 in]
        n122 = call <vilib>:"Add State(s) to Queue__jki_lib_state_machine.vi"("State(s) in Front (\"\")"=w273, "State(s) in (\"\")"=w282) -> ("States Out"=w281:string)  [unwired: 13 in]
      }
      frame "---------- New Category ----------" {
        # "Template Separator\n(You can make a copy of, or modify, this frame)"
        n123 = call <vilib>:"Add State(s) to Queue__jki_lib_state_machine.vi"("State(s) in (\"\")"=w286) -> ("States Out"=w285:string)  [unwired: 14 in]
      }
      frame "Load Files" {
        n124 = call <vilib>:"Add State(s) to Queue__jki_lib_state_machine.vi"("State(s) in (\"\")"=w308) -> ("States Out"=w307:string)  [unwired: 14 in]
        n125 = Unbundle By Name(w293) -> ("Extinction Cross section Path"=w292:path, "Multiple charge correction file Path"=w291:path)
        n126 = call "ReadBAESdataFromFileVer3.vi"("Factor Size Parameter"=1.0, "Factor Extinction"="Extinction Factor in Data", "Factor Ext Uncertainty"="Factor Ext Uncertainty in Data", "file path"=w292) -> ("Extinction data in graph format"=→"Extinction Data per size":T16, "Extinction ExtinctionUncertainity Size parameter and Number ofS sizes"=w290:T5)
        n127 = call "ReadParticleSizeSpectrum.vi"("file path"=w291, "Factor Size paramter"=1.0) -> ("SMPS sizes"=→"Size Distribution":cluster{"Sizes":dbl[], "Concentration":dbl[]}[], "Particle Distribution Data"=w304:T6)
        n128 = Strip Path(path=w292) -> (stripped path=w295:path, name=w299:string)
        n129 = Strip Path(path=w291) -> (stripped path=w294:path, name=w297:string)
        n130 = case shown="\"Initialize Sizes\"" w289 {
          tunnel: w290 -> [_ w311 _]
          frame "False", Default {
          }
          frame "Initialize Sizes" {
            n131 = Unbundle By Name(w311) -> ("Number ofSizes"=w310:dbl, "Sizes"=w309:dbl[])
            n132 = for {
              N: w310 -> [_]
              tunnel: [w316] -> w312 mode=indexing
              tunnel: w309 -> [w315] mode=indexing
              n133 = Number To Decimal String(number=w315) -> (decimal integer string=w316:string)  [unwired: 1 in]
            }
            n134 = Initialize Array(38 ("Item Symbols"), w310) -> (w313:i32[])
            n135 = property on="Diameters to fit" class="LstBox (strict)"("Item Symbols"=w313, "Item Names"=w312) -> ()  [unwired: 2 in, 2 out]
          }
          frame "Dont Initialize Sizes" {
          }
        }
        n136 = Bundle By Name(cluster=w293, "Extinction ExtinctionUncertainity Size parameter and Number ofS sizes"=w290, "Particle Distribution Data"=w304) -> (w305:T14)
        n137 = property on="Extinction Cross Section File" class="Path"("StartPath"=w295) -> ()  [unwired: 2 in, 2 out]
        n138 = property on="Mutiple Charge Data File" class="Path"("StartPath"=w294) -> ()  [unwired: 2 in, 2 out]
        n139 = String To Path(string=w299) -> (path=w298:path)
        n140 = String To Path(string=w297) -> (path=w296:path)
        n141 = local write "Extinction Cross Section File"(w298) -> ()
        n142 = local write "Mutiple Charge Data File"(w296) -> ()
      }
      frame "Append Mie Curve" {
        # "Calculate\nThe correction\nfor tested n and k"
        n143 = call <vilib>:"Add State(s) to Queue__jki_lib_state_machine.vi"("State(s) in (\"\")"=w346) -> ("States Out"=w345:string)  [unwired: 14 in]
        n144 = disable-structure shown="Disabled" {
          frame Disabled {
            n145 = control-ref of="Real Part vs wavelength"() -> (w348:refnum<vi>)
            n146 = control-ref of="Imaginary Part vs wavelength"() -> (w347:refnum<vi>)
            n147 = property on="Property Node" class="XYGraph (strict)" props=["Cursor", "Cursor Y"](reference=w348) -> ()  [unwired: 1 in, 3 out]
            n148 = property on="Property Node" class="XYGraph (strict)" props=["Cursor", "Cursor Y"](reference=w347) -> ()  [unwired: 1 in, 3 out]
          }
          frame Enabled {
          }
        }
        n149 = Unbundle By Name(w343) -> ("Baes data type definition"=w325:T8, "Baes data type definition.Extinction"=w326:dbl[], "Baes data type definition.Extinction Uncertainty"=w329:dbl[], "Baes data type definition.Number ofSizes"=w328:dbl)
        n150 = property on="Corrected for multiple charge particles" class="XYGraph (strict)"() -> ("Value"=w340:cluster{"Size parameters":dbl[], dbl[]}[])  [unwired: 2 in, 2 out]
        n151 = call "CalculateExtinctionCorrectionsToDoublyChargeParticleContribution.vi"("refractive index, imaginary"="k", "refractive index, real"="n", "Extinction ExtinctionUncertainity Size parameter and Number ofS sizes"=w325) -> ("Expected Extinction Cross Section"=w327:sgl[])  [unwired: 1 out]
        n152 = call "CalculateAreaOfFirstPeakofSizeDistribution.vi"("Extinction ExtinctionUncertainity Size parameter and Number ofS sizes"=w325) -> ("Area of First peak"=w323:dbl[])
        n153 = Subtract(x=w326, y=w327) -> (x-y=w324:dbl[])
        n154 = call "PlotMieCurve.vi"("refractive index, imaginary"="k", "refractive index, real"="n", "Use Extinction Factor"=FALSE, "Extinction ExtinctionUncertainity Size parameter and Number ofS sizes"=w325) -> ("Mie Results In Size Parameters"=w330:sgl[], "Size parameters"=w342:dbl[], "Extinction Crosssections"=w341:dbl[])
        n155 = Divide(x=w324, y=w323) -> (x/y=w322:dbl[])
        n156 = Subtract(x=w322, y=w330) -> (x-y=w332:dbl[])
        n157 = Bundle("Size parameters"=w342, "Extinction Crosssections"=w341) -> (w339:T17)  [unwired: 1 in]
        n158 = Divide(x=w332, y=w329) -> (x/y=w331:dbl[])
        n159 = Build Array (concatenate)(w340, w339) -> (w337:T18)
        n160 = Square(x=w331) -> (x^2=w321:dbl[])
        n161 = Array Size(array=w337) -> (size(s)=w336:i32)
        n162 = Add Array Elements(numeric array=w321) -> (sum=w320:dbl)
        n163 = Subtract(x=w336, y=1) -> (x-y=w334:i32)
        n164 = Divide(x=w320, y=w328) -> (x/y=→"Residue":dbl)
        n165 = property on="Corrected for multiple charge particles" class="XYGraph (strict)"("Value"=w337, "Active Plot"=w334, "Plot.Plot Color"=u32 0) -> ()  [unwired: 2 in, 2 out]
      }
      frame "Load Files MC" {
        # "Loading files for Monte Carlo simulation for the purpoese of error analysis"
        n166 = call <vilib>:"Add State(s) to Queue__jki_lib_state_machine.vi"("State(s) in (\"\")"=w360) -> ("States Out"=w359:string)  [unwired: 14 in]
        n167 = local read "Extinction Cross Section File"() -> (w353:path)
        n168 = local read "Mutiple Charge Data File"() -> (w352:path)
        n169 = local read "Diameter Factor"() -> (w349:dbl)
        n170 = call "ReadParticleSizeSpectrum.vi"("file path"=w352, "Factor Size paramter"=w349) -> ("Particle Distribution Data"=w354:T6)  [unwired: 1 out]
        n171 = call "ReadBAESdataFromFileMCVersion.vi"("file path"=w353) -> ("Extinction ExtinctionUncertainity Size parameter and Number ofS sizes"=w355:T5, "FullExtinctionData"=w351:dbl[][], "NumberOfMeasurementsperSize"=w350:i32)
        n172 = Bundle By Name(cluster=w357, "Extinction ExtinctionUncertainity Size parameter and Number ofS sizes"=w355, "Particle Distribution Data"=w354, "Extinction Cross section Path"=w353, "Multiple charge correction file Path"=w352, "FullExtinctionData"=w351, "NumberOfMeasurementsperSize"=w350) -> (w356:T14)
      }
      frame "Retrieve RI" {
        n173 = stacked-sequence {
          tunnel: w364 -> [w395 _]
          tunnel: [w397 _] -> w363
          tunnel: w361 -> [w377 _]
          frame #0 {
            n174 = case shown="\"UseFactors\"" w377 {
              tunnel: [1.0 ("Extinction Factor") "Extinction Factor"] -> w380
              tunnel: [1.0 ("Diameter Factor") "Diameter Factor"] -> w379
              tunnel: [0.0 ("Diameter Offset") "Diameter Offset"] -> w378
              frame "DontUseFactors", Default {
              }
              frame "UseFactors" {
              }
            }
            n175 = property on="Diameters to fit" class="LstBox (strict)"() -> ("Item Symbols"=w376:i32[])  [unwired: 2 in, 2 out]
            n176 = for {
              tunnel: w376 -> [w406] mode=indexing
              tunnel: 38 ("Item Symbols") -> [w405]
              tunnel: [w404] -> w374 mode=indexing
              n177 = Equal?(x=w406, y=w405) -> (x = y?=w404:bool)
            }
            n178 = property on="Max Wavelength" class="CmbBox"() -> ("Value"=w388:string)  [unwired: 2 in, 2 out]
            n179 = property on="Min Wavelength" class="CmbBox"() -> ("Value"=w389:string)  [unwired: 2 in, 2 out]
            n180 = property on="Retrieve RI" class="Bool"("BoolText.Text"="Running...." ("Boolean Text.Text")) -> ()  [unwired: 2 in, 2 out]
            n181 = Unbundle By Name(w395) -> ("Extinction ExtinctionUncertainity Size parameter and Number ofS sizes"=w372:T5, "Particle Distribution Data"=w373:T6)
            n182 = Decimal String To Number(string=w389) -> (number=w387:i32)  [unwired: 2 in, 1 out]
            n183 = Decimal String To Number(string=w388) -> (number=w386:i32)  [unwired: 2 in, 1 out]
            n184 = local read "General Data for RI Retrieval VI"() -> (w382:T3)
            n185 = local read "ExtinctionOrAbsorptionOrScattering"() -> (w369:i8)
            n186 = control-ref of="Real Part vs wavelength"() -> (w403:refnum<vi>)
            n187 = control-ref of="Not Corrected for Multiple charge Best fit result"() -> (w401:refnum<vi>)
            n188 = control-ref of="Imaginary Part vs wavelength"() -> (w402:refnum<vi>)
            n189 = control-ref of="Normalized Residuals vs Size parameter"() -> (w400:refnum<vi>)
            n190 = control-ref of="Simplex"() -> (w381:refnum<vi>)
            n191 = local read "Approximate Errors"() -> (w393:bool)
            n192 = Bundle("Real Part vs wavelength"=w403, "Imaginary Part vs wavelength"=w402, "Normalized Residuals vs Size parameter"=w400, "Not Corrected for Multiple charge Best fit result"=w401, "Simplex"=w381) -> (w399:T19)  [unwired: 1 in]
            n193 = Bundle By Name(cluster=w382, "Min WaveLength Index"=w387, "Max WaveLength Index"=w386, "Extinction Factor"="Extinction Factor", "Size Parameter Factor"="Size Parameter Factor", "Size Paramter Offset"="Size Parameter Offset", "Extinction Factor"=w380, "Diameter Factor"=w379, "Diameter Offset"=w378, "ExtinctionOrAbsorptionOrScattering"=w369) -> (w398:T3)
            n194 = call "RestructureDataAccordingToSelectedSizes.vi"("Extinction Data input"=w372, "Particle Distribution input"=w373, "Sizes to Fit"=w374) -> ("Extinciton Data ouput"=w371:T5, "Particle Distribution output"=w370:T6)
            n195 = call "RIRetrieval.vi"("General Data for RI Retrieval VI"=w398, "Approximate Errors"=w393, "Restrict to Positive Imaginary Part"="Restrict to Positive Imaginary Part", "Extinction Measured Data"=w371, "Calculate Errors"="Calculate Errors", "Particle Distribution Data"=w370, "Graph Refs"=w399, "Minimization method"="Minimization method") -> ("All Input data in one Cluster"=w390:T8, "RI results"=w396:T13)  [unwired: 2 out]
            n196 = Bundle By Name(cluster=w395, "RI results"=w396, "Baes data type definition"=w390, "Extinction ExtinctionUncertainity Size parameter and Number ofS sizes"=w371, "Particle Distribution Data"=w370) -> (w397:T14)
          }
          frame #1 {
            n197 = disable-structure shown="Disabled" {
              frame Disabled {
                n198 = One Button Dialog(message="RI retrieval finished successfully") -> ()  [unwired: 1 in, 1 out]
              }
              frame Enabled {
              }
            }
            n199 = property on="Retrieve RI" class="Bool"("BoolText.Text"="Retrieve RI" ("Boolean Text.Text")) -> ()  [unwired: 2 in, 2 out]
          }
        }
        n200 = call <vilib>:"Add State(s) to Queue__jki_lib_state_machine.vi"("State(s) in Front (\"\")"="Update Corrected multiple charge extinction graph" ("State(s) in Front (\"\")"), "State(s) in (\"\")"=w367) -> ("States Out"=w366:string)  [unwired: 13 in]
      }
      frame "Find Extinction and Size Parameter Factor" {
        n201 = stacked-sequence {
          tunnel: w417 -> [w454 _]
          tunnel: [w456 _] -> w416
          frame #0 {
            # "Real"
            n202 = property on="Max Wavelength" class="CmbBox"() -> ("Value"=w451:string)  [unwired: 2 in, 2 out]
            n203 = property on="Min Wavelength" class="CmbBox"() -> ("Value"=w452:string)  [unwired: 2 in, 2 out]
            n204 = local read "General Data for RI Retrieval VI"() -> (w423:T3)
            n205 = local read "Size Parameter Factor"() -> (w426:bool)
            n206 = local read "Size Parameter Offset"() -> (w425:bool)
            n207 = Decimal String To Number(string=w452) -> (number=w450:i32)  [unwired: 2 in, 1 out]
            n208 = Decimal String To Number(string=w451) -> (number=w449:i32)  [unwired: 2 in, 1 out]
            n209 = control-ref of="Simplex"() -> (w422:refnum<vi>)
            n210 = local read "Extinction Factor"() -> (w427:bool)
            n211 = control-ref of="Real Part vs wavelength"() -> (w460:refnum<vi>)
            n212 = control-ref of="Not Corrected for Multiple charge Best fit result"() -> (w458:refnum<vi>)
            n213 = control-ref of="Imaginary Part vs wavelength"() -> (w459:refnum<vi>)
            n214 = control-ref of="Normalized Residuals vs Size parameter"() -> (w457:refnum<vi>)
            n215 = Unbundle By Name(w454) -> ("Extinction ExtinctionUncertainity Size parameter and Number ofS sizes"=w447:T5, "Particle Distribution Data"=w445:T6)
            n216 = Bundle By Name(cluster=w423, "Min WaveLength Index"=w450, "Max WaveLength Index"=w449, "Extinction Factor"=w427, "Size Parameter Factor"=w426, "Size Paramter Offset"=w425, "ExtinctionOrAbsorptionOrScattering"="ExtinctionOrAbsorptionOrScattering") -> (w424:T3)
            n217 = Bundle(cluster="Graph Refs", "Real Part vs wavelength"=w460, "Imaginary Part vs wavelength"=w459, "Normalized Residuals vs Size parameter"=w457, "Not Corrected for Multiple charge particles"=w458, "Simplex 2"=w422) -> (w440:T4)
            n218 = local read "Restrict to Positive Imaginary Part"() -> (w443:bool)
            n219 = local read "Minimization method"() -> (w446:u16)
            n220 = local read "Approximate Errors"() -> (w448:bool)
            n221 = local read "Calculate Errors"() -> (w444:bool)
            n222 = Bundle(cluster="Data for RIRetrieval VI", "Approximate Errors"=w448, "Extinction ExtinctionUncertainity Size parameter and Number ofS sizes"=w447, "Minimization method"=w446, "Graph Ref"=w440, "Particle Distribution Data"=w445, "Calculate Errors"=w444, "Restrict to Positive Imaginary Part"=w443, "MinMaxWavelength"=w424) -> (w433:T7)
            n223 = call "RIRetrieval.vi"("General Data for RI Retrieval VI"=w424, "Approximate Errors"=w448, "Restrict to Positive Imaginary Part"=w443, "Extinction Measured Data"=w447, "Calculate Errors"=w444, "Particle Distribution Data"=w445, "Graph Refs"=w440, "Minimization method"=w446) -> ("All Input data in one Cluster"=w453:T8, "RI results"=w455:T13)  [unwired: 2 out]
            n224 = Bundle By Name(cluster=w454, "RI results"=w455, "Baes data type definition"=w453) -> (w456:T14)
            n225 = To Variant(anything=w433) -> (Variant=w437:variant)
            n226 = vi-ref "FindExtinctionAndSizeParameterFactors.vi"() -> (w436:refnum<vi>)
            n227 = Build Array(5.0 ("element"), 5.0 ("element")) -> (w439:dbl[])
            n228 = call-poly <vilib>:"Unconstrained Optimization.vi"("function data"=w437, "objective function"=w436, "stopping criteria"=T11 {"function tolerance"=0.01, "parameter tolerance"=0.05, "max iterations"=10, "max function calls"=1000, "gradient tolerance"=1000000.0, "max time (sec)"=-1.0}, "start"=w439) -> ("minimum"=w429:dbl[])  [unwired: 4 in, 3 out]
            n229 = Index Array(array=w429, index=0) -> (element=→"Minimized Extinction Factor":dbl)
            n230 = Index Array(array=w429, index=0) -> (element=→"Minimized Size Parameter Factor":dbl)
          }
          frame #1 {
            n231 = One Button Dialog(message="RI retrieval finished successfully") -> ()  [unwired: 1 in, 1 out]
          }
        }
        n232 = call <vilib>:"Add State(s) to Queue__jki_lib_state_machine.vi"("State(s) in Front (\"\")"="Update Corrected multiple charge extinction graph" ("State(s) in Front (\"\")"), "State(s) in (\"\")"=w420) -> ("States Out"=w419:string)  [unwired: 13 in]
      }
      frame "Find Extinction Factor" {
        n233 = stacked-sequence {
          tunnel: w464 -> [w473 _]
          tunnel: [w502 _] -> w463
          frame #0 {
            n234 = Subtract(x="Diameter FO Finish", y="Diameter FO start") -> (x-y=w497:dbl)
            n235 = Divide(x=w497, y="Diameter FO Interval") -> (x/y=w495:dbl)
            n236 = Round To Nearest(number=w495) -> (nearest integer value=w494:dbl)
            n237 = Increment(x=w494) -> (x+1=w493:dbl)
            n238 = call-poly <vilib>:"Ramp Pattern.vi"("start"="Diameter FO start", "end"="Diameter FO Finish", "samples"=w493) -> ("Ramp Pattern"=w477:dbl[])  [unwired: 7 in, 1 out]
            n239 = Tick Count (ms)() -> (millisecond timer value=w476:u32)
            n240 = property on="Diameters to fit" class="LstBox (strict)"() -> ("Item Symbols"=w475:i32[])  [unwired: 2 in, 2 out]
            n241 = for {
              tunnel: w475 -> [w505] mode=indexing
              tunnel: 38 ("Item Symbols") -> [w504]
              tunnel: [w503] -> w470 mode=indexing
              n242 = Equal?(x=w505, y=w504) -> (x = y?=w503:bool)
            }
            n243 = Unbundle By Name(w473) -> ("Particle Distribution Data"=w472:T6, "Extinction ExtinctionUncertainity Size parameter and Number ofS sizes"=w471:T5)
            n244 = call "RestructureDataAccordingToSelectedSizes.vi"("Extinction Data input"=w471, "Particle Distribution input"=w472, "Sizes to Fit"=w470) -> ("Extinciton Data ouput"=w468:T5, "Particle Distribution output"=w469:T6)
            n245 = for {
              tunnel: [w535] -> w501
              tunnel: w473 -> [w534]
              tunnel: [w533] -> w500
              tunnel: w477 -> [w526] mode=indexing
              tunnel: [w525] -> w480 mode=indexing
              tunnel: [w523] -> _
              tunnel: ["Extinction Factor Start"] -> _
              tunnel: [w514] -> w478
              tunnel: w477 -> [w515]
              tunnel: w476 -> [w513]
              tunnel: w469 -> [w507]
              tunnel: w468 -> [w506]
              i -> [w511]
              n246 = Subtract(x="Extinction Factor Finish", y="Extinction Factor Start") -> (x-y=w520:dbl)
              n247 = Divide(x=w520, y="Extinction Factor Interval") -> (x/y=w518:dbl)
              n248 = Array Size(array=w515) -> (size(s)=w510:i32)
              n249 = Round To Nearest(number=w518) -> (nearest integer value=w517:dbl)
              n250 = Subtract(x="Extinction Factor Finish", y="Extinction Factor Start") -> (x-y=w524:dbl)
              n251 = Increment(x=w517) -> (x+1=w516:dbl)
              n252 = Divide(x=w524, y=w516) -> (x/y=w523:dbl)
              n253 = call-poly <vilib>:"Ramp Pattern.vi"("start"="Extinction Factor Start", "end"="Extinction Factor Finish", "samples"=w516) -> ("Ramp Pattern"=w514:dbl[])  [unwired: 7 in, 1 out]
              n254 = Array Size(array=w514) -> (size(s)=w508:i32)
              n255 = control-ref of="Progress bar for Extinction search"() -> (w512:refnum<vi>)
              n256 = Multiply(x=w510, y=w508) -> (x*y=w509:i32)
              n257 = for {
                tunnel: [w570] -> w535
                tunnel: w534 -> [_]
                tunnel: [w585] -> w533
                tunnel: w514 -> [w571] mode=indexing
                tunnel: [w566] -> w532 mode=indexing
                tunnel: [w565] -> w531 mode=indexing
                tunnel: [w564] -> w525 mode=indexing
                tunnel: w526 -> [w558]
                shift-right: [w542] -> _
                shift-left: w513 -> [w550]
                tunnel: w511 -> [_]
                tunnel: w512 -> [w548]
                tunnel: w511 -> [w545]
                tunnel: w509 -> [w541]
                tunnel: w508 -> [w538]
                tunnel: w507 -> [w537]
                tunnel: w506 -> [w536]
                i -> [w549]
                n258 = local read "Size Parameter Factor"() -> (w575:bool)
                n259 = local read "Size Parameter Offset"() -> (w574:bool)
                n260 = local read "Extinction Factor"() -> (w576:bool)
                n261 = property on="Max Wavelength" class="CmbBox"() -> ("Value"=w583:string)  [unwired: 2 in, 2 out]
                n262 = property on="Min Wavelength" class="CmbBox"() -> ("Value"=w584:string)  [unwired: 2 in, 2 out]
                n263 = Decimal String To Number(string=w584) -> (number=w582:i32)  [unwired: 2 in, 1 out]
                n264 = Decimal String To Number(string=w583) -> (number=w581:i32)  [unwired: 2 in, 1 out]
                n265 = Select(t=w558, s="Diameter Factor or Offset", f=0.0) -> (s? t:f=w560:dbl)
                n266 = Select(t=1.0 ("Diameter Factor"), s="Diameter Factor or Offset", f=w558) -> (s? t:f=w556:dbl)
                n267 = Tick Count (ms)() -> (millisecond timer value=w542:u32)
                n268 = Bundle By Name(cluster="General Data for RI Retrieval VI", "Min WaveLength Index"=w582, "Max WaveLength Index"=w581, "Extinction Factor"=w576, "Size Parameter Factor"=w575, "Size Paramter Offset"=w574, "Extinction Factor"=w571, "Diameter Offset"=w560, "Diameter Factor"=w556) -> (w573:T3)
                n269 = Subtract(x=w542, y=w550) -> (x-y=w551:u32)
                n270 = Multiply(x=w538, y=w545) -> (x*y=w544:i32)
                n271 = control-ref of="Real Part vs wavelength"() -> (w589:refnum<vi>)
                n272 = control-ref of="Not Corrected for Multiple charge Best fit result"() -> (w587:refnum<vi>)
                n273 = control-ref of="Imaginary Part vs wavelength"() -> (w588:refnum<vi>)
                n274 = control-ref of="Normalized Residuals vs Size parameter"() -> (w586:refnum<vi>)
                n275 = control-ref of="Simplex"() -> (w555:refnum<vi>)
                n276 = Increment(x=w549) -> (x+1=w543:i32)
                n277 = Add(x=w544, y=w543) -> (x+y=w540:i32)
                n278 = Subtract(x=w541, y=w540) -> (x-y=w539:i32)
                n279 = property class="Slide (strict)"(reference=w548, "Value"=w540) -> ()  [unwired: 1 in, 2 out]
                n280 = Bundle(cluster="Graph Refs 2", "Real Part vs wavelength"=w589, "Imaginary Part vs wavelength"=w588, "Normalized Residuals vs Size parameter"=w586, "Not Corrected for Multiple charge particles"=w587, "Simplex 2"=w555) -> (w577:T4)
                n281 = local read "Restrict to Positive Imaginary Part"() -> (w579:bool)
                n282 = Divide(x=w551, y=u32 60000) -> (x/y=w547:dbl)
                n283 = Multiply(x=w547, y=w539) -> (x*y=→"Time Left (min)":dbl)
                n284 = local read "Minimization method"() -> (w580:u16)
                n285 = local read "Max Wavelength"() -> (w563:string)
                n286 = call "RIRetrieval.vi"("General Data for RI Retrieval VI"=w573, "Approximate Errors"=FALSE, "Restrict to Positive Imaginary Part"=w579, "Extinction Measured Data"=w536, "Calculate Errors"=FALSE, "Particle Distribution Data"=w537, "Graph Refs"=w577, "Minimization method"=w580) -> ("All Input data in one Cluster"=w585:T8, "RI results"=w570:T13)  [unwired: 2 out]
                n287 = Unbundle By Name(w570) -> ("Real RI"=w569:dbl[], "Imaginary RI"=w568:dbl[], "Residue"=w567:dbl[])
                n288 = Decimal String To Number(string=w563) -> (number=w562:i32)  [unwired: 2 in, 1 out]
                n289 = Index Array(array=w569, index=w562) -> (element=w566:dbl)
                n290 = Index Array(array=w568, index=w562) -> (element=w565:dbl)
                n291 = Index Array(array=w567, index=w562) -> (element=w564:dbl)
              }
              n292 = property class="Slide (strict)"(reference=w512, "Scale.Maximum"=w509) -> ()  [unwired: 1 in, 2 out]
              n293 = Bundle("Ramp Pattern"=w514, w532) -> (w530:cluster{"Ramp Pattern":dbl[], dbl[]})  [unwired: 1 in]
              n294 = Bundle("Ramp Pattern"=w514, w531) -> (w529:cluster{"Ramp Pattern":dbl[], dbl[]})  [unwired: 1 in]
              n295 = Bundle("Ramp Pattern"=w514, w525) -> (w528:cluster{"Ramp Pattern":dbl[], dbl[]})  [unwired: 1 in]
              n296 = Build Array(w530, w529, w528) -> (→"Extinction Factor Results":cluster{"Ramp Pattern":dbl[], dbl[]}[])
            }
            "Residue Graph Matrix" <- w480
            n297 = Bundle By Name(cluster=w473, "RI results"=w501, "Baes data type definition"=w500) -> (w502:T14)
            n298 = Array Max & Min(array=w480) -> (min index (indices)=w492:i32[])  [unwired: 3 out]
            n299 = call <vilib>:"create_plot_surface.vi"("z matrix"=w480, "y vector"=w478, "x vector"=w477) -> ("plots out"=→"3D Graph":refnum<class "Base Datatype.lvclass">[])  [unwired: 2 in, 6 out]
            n300 = local read "Diameter Factor or Offset"() -> (w484:bool)
            n301 = Index Array(array=w492, index #1=0 ("index"), index #2=1 ("index")) -> (element #1=w488:i32, element #2=w489:i32)
            n302 = Index Array(array=w478, index=w489) -> (element=w487:dbl)
            n303 = Index Array(array=w477, index=w488) -> (element=w483:dbl)
            n304 = local write "Extinction Factor"(w487) -> ()
            n305 = Select(t=1.0 ("Diameter Factor"), s=w484, f=w483) -> (s? t:f=w481:dbl)
            n306 = Select(t=w483, s=w484, f=0.0) -> (s? t:f=w482:dbl)
            n307 = local write "Diameter Factor"(w481) -> ()
            n308 = local write "Diameter Offset"(w482) -> ()
          }
          frame #1 {
          }
        }
        n309 = call <vilib>:"Add State(s) to Queue__jki_lib_state_machine.vi"("State(s) in Front (\"\")"="Load Files >> Dont Initialize Sizes\nRetrieve RI >> UseFactors\nUpdate Corrected multiple charge extinction graph" ("State(s) in Front (\"\")"), "State(s) in (\"\")"=w467) -> ("States Out"=w466:string)  [unwired: 13 in]
      }
      frame "Save RI to file" {
        n310 = stacked-sequence {
          tunnel: w591 -> [w644 _]
          frame #0 {
            n311 = local read "Approximate Errors"() -> (w609:bool)
            n312 = property on="Max Wavelength" class="CmbBox"() -> ("Value"=w620:string)  [unwired: 2 in, 2 out]
            n313 = property on="Min Wavelength" class="CmbBox"() -> ("Value"=w621:string)  [unwired: 2 in, 2 out]
            n314 = Unbundle By Name(w644) -> ("Extinction Cross section Path"=w652:path, "RI results.Wavelength"=w653:dbl[], "RI results.Real RI"=w654:dbl[], "RI results.Std Real RI"=w623:dbl[], "RI results.Imaginary RI"=w624:dbl[], "RI results.Std Imaginary RI"=w622:dbl[], "RI results.Residue"=w597:dbl[], "RI results.Extinction Factor"=w596:dbl[], "RI results.Diameter Factor"=w595:dbl[], "RI results.Diameter Offset"=w594:dbl[])
            n315 = local read "Calculate Errors"() -> (w610:bool)
            n316 = Decimal String To Number(string=w620) -> (number=w619:i32)  [unwired: 2 in, 1 out]
            n317 = Decimal String To Number(string=w621) -> (number=w599:i32)  [unwired: 2 in, 1 out]
            n318 = Unbundle By Name(w644) -> ("Extinction ExtinctionUncertainity Size parameter and Number ofS sizes"=w643:T5, "Particle Distribution Data"=w642:T6, "RI results"=w641:T13)
            n319 = Build Array(w653, w654, w624, w623, w622, w597, w596, w595, w594) -> (w651:dbl[][])
            n320 = Select(t="+ApproxError" ("name or relative path"), s=w609, f="-ApproxError" ("name or relative path")) -> (s? t:f=w608:string)
            n321 = Subtract(x=w619, y=w599) -> (x-y=w649:i32)
            n322 = call <vilib>:"Get File Extension.vi"("file"=w652) -> ("filename without extension"=w602:string)  [unwired: 7 in, 3 out]
            n323 = local read "Restrict to Positive Imaginary Part"() -> (w615:bool)
            n324 = Concatenate Strings(w602, w608) -> (w607:string)
            n325 = call "PrepareExtinctionCrossSectionToFile.vi"("Extinction ExtinctionUncertainity Size parameter and Number ofS sizes"=w643, "RI results"=w641, "Particle Distribution Data"=w642, "Min Wavelength index"=w599, "Max Wavelength index"=w619) -> ("Extinction"=w639:dbl[][], "CorrectedExtinction"=w640:dbl[][], "Sigma_diameter_string"=w629:string[])
            n326 = Transpose 2D Array(2D array=w651) -> (transposed array=w650:dbl[][])
            n327 = Increment(x=w649) -> (x+1=w598:i32)
            n328 = Select(t="+Error" ("name or relative path"), s=w610, f="-Error" ("name or relative path")) -> (s? t:f=w606:string)
            n329 = Concatenate Strings(w607, w606) -> (w605:string)
            n330 = Select(t="+Restricted" ("name or relative path"), s=w615, f="-Restricted" ("name or relative path")) -> (s? t:f=w604:string)
            n331 = Array Subset(array=w650, index (row)=w599, length (row)=w598) -> (w648:dbl[][])  [unwired: 2 in]
            n332 = Array Subset(array=w639, index (row)=w599, length (row)=w598) -> (w638:dbl[][])  [unwired: 2 in]
            n333 = Array Subset(array=w640, index (row)=w599, length (row)=w598) -> (w637:dbl[][])  [unwired: 2 in]
            n334 = Concatenate Strings(w605, w604) -> (w603:string)
            n335 = Transpose 2D Array(2D array=w638) -> (transposed array=w636:dbl[][])
            n336 = Transpose 2D Array(2D array=w637) -> (transposed array=w635:dbl[][])
            n337 = Number To Fractional String(number=w648, precision (6)=i16 3) -> (F-format string=w633:string[][])  [unwired: 2 in]
            n338 = Build Array (concatenate)(w636, w635) -> (w634:dbl[][])
            n339 = Concatenate Strings(w603, "_RIresult.txt" ("name or relative path")) -> (w655:string)
            n340 = Strip Path(path=w652) -> (stripped path=w656:path)  [unwired: 1 out]
            n341 = Number To Engineering String(4:w634) -> (0:w626:string[][])  [unwired: 3 in]
            n342 = Build Path(base path=w656, name or relative path=w655) -> (appended path=w645:path)
            "Saved RI to this filename and path" <- w645
            n343 = Transpose 2D Array(2D array=w626) -> (transposed array=w625:string[][])
            n344 = Build Array (concatenate)(string[] ["Wavelength (nm)", "Real Part", "Imaginary Part", "Conf Real Part", "Conf Imaginary part", "Residue (MDBF)", "Extinction Factor", "Diameter Factor", "Diameter Offset (nm)"] ("column headers"), w633) -> (w630:string[][])
            n345 = Build Array (concatenate)(w629, w625) -> (w628:string[][])
            n346 = Transpose 2D Array(2D array=w630) -> (transposed array=w632:string[][])
            n347 = Transpose 2D Array(2D array=w628) -> (transposed array=w627:string[][])
            n348 = Build Array (concatenate)(w632, w627) -> (w601:string[][])
            n349 = Transpose 2D Array(2D array=w601) -> (transposed array=w600:string[][])
            n350 = call-poly <vilib>:"Write To Spreadsheet File.vi"("transpose? (no:F)"=FALSE, "2D data"=w600, "file path (dialog if empty)"=w645) -> ()  [unwired: 5 in, 1 out]
          }
          frame #1 {
            n351 = One Button Dialog(message="File save was completed successfully") -> ()  [unwired: 1 in, 1 out]
          }
        }
        n352 = call <vilib>:"Add State(s) to Queue__jki_lib_state_machine.vi"("State(s) in (\"\")"=w593) -> ("States Out"=w592:string)  [unwired: 14 in]
      }
      frame "Save RI to File Expanded Edition" {
        n353 = stacked-sequence {
          tunnel: w659 -> [w718 _]
          frame #0 {
            # "This inlcudes the number of sizes and the reduced chi^2 measurement for each wavelength"
            n354 = Unbundle By Name(w718) -> ("Extinction Cross section Path"=w726:path, "RI results.Wavelength"=w727:dbl[], "RI results.Real RI"=w728:dbl[], "RI results.Std Real RI"=w696:dbl[], "RI results.Imaginary RI"=w697:dbl[], "RI results.Std Imaginary RI"=w695:dbl[], "RI results.Residue"=w667:dbl[], "Extinction ExtinctionUncertainity Size parameter and Number ofS sizes.Number ofSizes"=w666:dbl)
            n355 = Build Array(w727, w728, w697, w696, w695, w667) -> (w725:dbl[][])
            n356 = Transpose 2D Array(2D array=w725) -> (transposed array=w724:dbl[][])
            n357 = property on="Min Wavelength" class="CmbBox"() -> ("Value"=w694:string)  [unwired: 2 in, 2 out]
            n358 = property on="Max Wavelength" class="CmbBox"() -> ("Value"=w693:string)  [unwired: 2 in, 2 out]
            n359 = Decimal String To Number(string=w693) -> (number=w691:i32)  [unwired: 2 in, 1 out]
            n360 = Decimal String To Number(string=w694) -> (number=w692:i32)  [unwired: 2 in, 1 out]
            n361 = Unbundle By Name(w718) -> ("Extinction ExtinctionUncertainity Size parameter and Number ofS sizes"=w717:T5, "Particle Distribution Data"=w716:T6, "RI results"=w715:T13)
            n362 = Subtract(x=w691, y=w692) -> (x-y=w723:i32)
            n363 = call "PrepareExtinctionCrossSectionToFile.vi"("Extinction ExtinctionUncertainity Size parameter and Number ofS sizes"=w717, "RI results"=w715, "Particle Distribution Data"=w716, "Min Wavelength index"=w692, "Max Wavelength index"=w691) -> ("Extinction"=w712:dbl[][], "CorrectedExtinction"=w714:dbl[][], "Sigma_diameter_string"=w702:string[])
            n364 = Increment(x=w723) -> (x+1=w713:i32)
            n365 = Array Subset(array=w724, index (row)=w692, length (row)=w713) -> (w722:dbl[][])  [unwired: 2 in]
            n366 = Array Subset(array=w712, index (row)=w692, length (row)=w713) -> (w711:dbl[][])  [unwired: 2 in]
            n367 = Array Subset(array=w714, index (row)=w692, length (row)=w713) -> (w710:dbl[][])  [unwired: 2 in]
            n368 = Transpose 2D Array(2D array=w711) -> (transposed array=w709:dbl[][])
            n369 = Transpose 2D Array(2D array=w710) -> (transposed array=w708:dbl[][])
            n370 = Number To Fractional String(number=w722, precision (6)=i16 3) -> (F-format string=w706:string[][])  [unwired: 2 in]
            n371 = Build Array (concatenate)(w709, w708) -> (w707:dbl[][])
            n372 = Number To Engineering String(4:w707) -> (0:w699:string[][])  [unwired: 3 in]
            n373 = Transpose 2D Array(2D array=w699) -> (transposed array=w698:string[][])
            n374 = local read "Calculate Errors"() -> (w682:bool)
            n375 = Build Array (concatenate)(string[] ["Wavelength (nm)", "Real Part", "Imaginary Part", "Conf Real Part", "Conf Imaginary part", "Eta (reduced Chi^2)"] ("column headers"), w706) -> (w703:string[][])
            n376 = Build Array (concatenate)(w702, w698) -> (w701:string[][])
            n377 = local read "Approximate Errors"() -> (w681:bool)
            n378 = Transpose 2D Array(2D array=w703) -> (transposed array=w705:string[][])
            n379 = Transpose 2D Array(2D array=w701) -> (transposed array=w700:string[][])
            n380 = local read "Restrict to Positive Imaginary Part"() -> (w687:bool)
            n381 = Select(t="+ApproxError" ("name or relative path"), s=w681, f="-ApproxError" ("name or relative path")) -> (s? t:f=w680:string)
            n382 = Build Array (concatenate)(w705, w700) -> (w669:string[][])
            n383 = Select(t="+Error" ("name or relative path"), s=w682, f="-Error" ("name or relative path")) -> (s? t:f=w678:string)
            n384 = call <vilib>:"Get File Extension.vi"("file"=w726) -> ("filename without extension"=w665:string)  [unwired: 7 in, 3 out]
            n385 = Number To Decimal String(number=w666) -> (decimal integer string=w664:string)  [unwired: 1 in]
            n386 = Concatenate Strings(w665, w680) -> (w679:string)
            n387 = Array Size(array=w669) -> (size(s)=w674:i32[])
            n388 = Concatenate Strings(w665, "_" ("element"), w664) -> (w662:string)
            n389 = Select(t="+Restricted" ("name or relative path"), s=w687, f="-Restricted" ("name or relative path")) -> (s? t:f=w676:string)
            n390 = Concatenate Strings(w679, w678) -> (w677:string)
            n391 = Index Array(array=w674, index=0) -> (element=w672:i32)
            n392 = for {
              N: w672 -> [_]
              tunnel: [w732] -> w671 mode=indexing
              tunnel: w662 -> [w733]
              i -> [w735]
              n393 = Equal To 0?(x=w735) -> (x = 0?=w734:bool)
              n394 = Select(t=w733, s=w734, f="") -> (s? t:f=w732:string)
            }
            n395 = Concatenate Strings(w677, w676) -> (w675:string)
            n396 = Concatenate Strings(w675, "-RIresult.txt" ("name or relative path")) -> (w729:string)
            n397 = Strip Path(path=w726) -> (stripped path=w730:path)  [unwired: 1 out]
            n398 = Build Path(base path=w730, name or relative path=w729) -> (appended path=w719:path)
            "Saved RI to this filename and path 2" <- w719
            n399 = Transpose 2D Array(2D array=w669) -> (transposed array=w668:string[][])
            n400 = Build Array (concatenate)(w671, w668) -> (w670:string[][])
            n401 = call-poly <vilib>:"Write To Spreadsheet File.vi"("transpose? (no:F)"=FALSE, "2D data"=w670, "file path (dialog if empty)"=w719) -> ()  [unwired: 5 in, 1 out]
          }
          frame #1 {
            n402 = One Button Dialog(message="File save was completed successfully") -> ()  [unwired: 1 in, 1 out]
          }
        }
        n403 = call <vilib>:"Add State(s) to Queue__jki_lib_state_machine.vi"("State(s) in (\"\")"=w661) -> ("States Out"=w660:string)  [unwired: 14 in]
      }
      frame "Save RI -Monte Carlo to file" {
        n404 = stacked-sequence {
          tunnel: w738 -> [w758 _]
          frame #0 {
            n405 = Unbundle By Name(w758) -> ("Extinction Cross section Path"=w748:path, "RI MC results.Wavelength"=w749:dbl[], "RI MC results.Real RI"=w753:dbl[], "RI MC results.Std Real RI"=w752:dbl[], "RI MC results.Imaginary RI"=w751:dbl[], "RI MC results.Std Imaginary RI"=w750:dbl[])
            n406 = Build Array(w749, w753, w752, w751, w750) -> (w747:dbl[][])
            n407 = call <vilib>:"Get File Extension.vi"("file"=w748) -> ("filename without extension"=w756:string)  [unwired: 7 in, 3 out]
            n408 = Transpose 2D Array(2D array=w747) -> (transposed array=w742:dbl[][])
            n409 = Concatenate Strings(w756, "-RI-MC-result.xls" ("name or relative path")) -> (w754:string)
            n410 = Strip Path(path=w748) -> (stripped path=w757:path)  [unwired: 1 out]
            n411 = Number To Fractional String(number=w742, precision (6)=i16 3) -> (F-format string=w743:string[][])  [unwired: 2 in]
            n412 = Build Array (concatenate)(string[] ["Wavelength (nm)", "Real Part (MC)", "Std Real Part (MC)", "Imaginary Part  (MC)", "Std Imaginary part (MC)"] ("column headers"), w743) -> (w745:string[][])
            n413 = Build Path(base path=w757, name or relative path=w754) -> (appended path=w744:path)
            "Saved RI (MC) to this filename and path" <- w744
            n414 = call-poly <vilib>:"Write To Spreadsheet File.vi"("2D data"=w745, "file path (dialog if empty)"=w744) -> ()  [unwired: 6 in, 1 out]
          }
          frame #1 {
            n415 = One Button Dialog(message="File save was completed successfully") -> ()  [unwired: 1 in, 1 out]
          }
        }
        n416 = call <vilib>:"Add State(s) to Queue__jki_lib_state_machine.vi"("State(s) in (\"\")"=w740) -> ("States Out"=w739:string)  [unwired: 14 in]
      }
      frame "Retrieve RI Monte Carlo" {
        w783 = T13 {"Real RI"=[], "Imaginary RI"=[], "Std Imaginary RI"=[], "Std Real RI"=[], "Wavelength"=[], "Residue"=[], "Extinction Factor"=[], "Diameter Factor"=[], "Diameter Offset"=[], "Best fit result"=[], "Normalized Residuals"=[]}  # RI MC results
        n417 = call <vilib>:"Add State(s) to Queue__jki_lib_state_machine.vi"("State(s) in (\"\")"=w810) -> ("States Out"=w809:string)  [unwired: 14 in]
        n418 = property on="Min Wavelength" class="CmbBox"() -> ("Value"=w767:string)  [unwired: 2 in, 2 out]
        n419 = property on="Max Wavelength" class="CmbBox"() -> ("Value"=w765:string)  [unwired: 2 in, 2 out]
        n420 = Decimal String To Number(string=w767) -> (number=w766:i32)  [unwired: 2 in, 1 out]
        n421 = Decimal String To Number(string=w765) -> (number=w764:i32)  [unwired: 2 in, 1 out]
        n422 = Unbundle By Name(w782) -> ("Extinction ExtinctionUncertainity Size parameter and Number ofS sizes"=w804:T5, "Particle Distribution Data"=w807:T6)
        n423 = local read "General Data for RI Retrieval VI"() -> (w760:T3)
        n424 = local read "Size Parameter Factor"() -> (w762:bool)
        n425 = local read "Size Parameter Offset"() -> (w761:bool)
        n426 = local read "Extinction Factor"() -> (w763:bool)
        n427 = Bundle(cluster=w760, "Min WaveLength Index"=w766, "Max WaveLength Index"=w764, "Extinction Factor"=w763, "Size Parameter Factor"=w762, "Size Paramter Offset"=w761) -> (w774:T3)  [unwired: 4 in]
        n428 = Unbundle By Name(w804) -> ("Extinction"=w806:dbl[][], "Extinction Uncertainty"=w805:dbl[][])
        n429 = local read "Restrict to Positive Imaginary Part"() -> (w768:bool)
        n430 = local read "Size of statistics"() -> (w784:i32)
        n431 = local read "Size of statistics"() -> (w772:i32)
        n432 = control-ref of="MC progress"() -> (w773:refnum<vi>)
        n433 = Tick Count (ms)() -> (millisecond timer value=w785:u32)
        n434 = property class="Slide (strict)"(reference=w773, "Scale.Maximum"=w772) -> ()  [unwired: 1 in, 2 out]
        n435 = for {
          N: w784 -> [_]
          tunnel: w807 -> [w845]
          tunnel: w806 -> [w842]
          tunnel: w805 -> [w841]
          tunnel: w804 -> [w839]
          tunnel: [w834] -> w803 mode=indexing
          tunnel: [w830] -> w792 mode=indexing
          tunnel: [w829] -> w776
          tunnel: w784 -> [w824]
          shift-right: [w821] -> _
          shift-left: w785 -> [w828]
          tunnel: w774 -> [w820]
          tunnel: w773 -> [w819]
          tunnel: [w817] -> w771
          tunnel: w768 -> [w813]
          i -> [w818]
          n436 = for {
            tunnel: w842 -> [w851] mode=indexing
            tunnel: w841 -> [w850] mode=indexing
            tunnel: [w849] -> w840 mode=indexing
            n437 = for {
              tunnel: w851 -> [w859] mode=indexing
              tunnel: w850 -> [w857] mode=indexing
              tunnel: [w852] -> w849 mode=indexing
              w856 = 1000000000.0 ("y")
              n438 = Multiply(x=w859, y=w856) -> (x*y=w858:dbl)
              n439 = Multiply(x=w857, y=w856) -> (x*y=w855:dbl)
              n440 = Random Number (0-1)() -> (number: 0 to 1=w860:dbl)
              n441 = call-poly <vilib>:"Continuous Inverse CDF.vi"("std"=w855, "mean"=w858, "cdf(x)"=w860) -> ("x"=w854:dbl)  [unwired: 7 in, 1 out]
              n442 = Multiply(x=w854, y=1e-09) -> (x*y=w852:dbl)
            }
          }
          n443 = Tick Count (ms)() -> (millisecond timer value=w821:u32)
          n444 = Subtract(x=w821, y=w828) -> (x-y=w827:u32)
          n445 = Increment(x=w818) -> (x+1=w817:i32)
          n446 = property class="Slide (strict)"(reference=w819, "Value"=w817) -> ()  [unwired: 1 in, 2 out]
          n447 = Divide(x=w827, y=u32 60000) -> (x/y=w825:dbl)
          n448 = Subtract(x=w824, y=w818) -> (x-y=w823:i32)
          n449 = Multiply(x=w825, y=w823) -> (x*y=→"Time Left (min) (MC)":dbl)
          n450 = control-ref of="Simplex"() -> (w812:refnum<vi>)
          n451 = control-ref of="Real Part vs wavelength"() -> (w848:refnum<vi>)
          n452 = control-ref of="Not Corrected for Multiple charge Best fit result"() -> (w846:refnum<vi>)
          n453 = control-ref of="Imaginary Part vs wavelength"() -> (w847:refnum<vi>)
          n454 = control-ref of="Normalized Residuals vs Size parameter"() -> (w844:refnum<vi>)
          n455 = local read "Minimization method"() -> (w816:u16)
          n456 = local read "Calculate Errors"() -> (w814:bool)
          n457 = Bundle By Name(cluster=w839, "Extinction"=w840) -> (w838:T5)
          n458 = Bundle("Real Part vs wavelength"=w848, "Imaginary Part vs wavelength"=w847, "Normalized Residuals vs Size parameter"=w844, "Not Corrected for Multiple charge Best fit result"=w846, "Simplex"=w812) -> (w843:T19)  [unwired: 1 in]
          n459 = call "RIRetrieval.vi"("General Data for RI Retrieval VI"=w820, "Approximate Errors"="Approximate Errors", "Restrict to Positive Imaginary Part"=w813, "Extinction Measured Data"=w838, "Calculate Errors"=w814, "Particle Distribution Data"=w845, "Graph Refs"=w843, "Minimization method"=w816) -> ("Imaginary Part vs wavelength"=w831:cluster{dbl[], dbl[]}[], "Real Part vs wavelength"=w837:cluster{dbl[], dbl[]}[])  [unwired: 2 out]
          n460 = Index Array(array=w837, index=0) -> (element=w835:cluster{dbl[], dbl[]})
          n461 = Index Array(array=w831, index=0) -> (element=w832:cluster{dbl[], dbl[]})
          n462 = Unbundle(w832) -> (w830:dbl[])  [unwired: 1 out]
          n463 = Unbundle(w835) -> (w829:dbl[], w834:dbl[])
          "Loop index (MC)" <- w818
        }
        n464 = call <vilib>:"Covariance Matrix.vi"("X"=w803) -> ("mean vector"=w775:dbl[], "covariance matrix V"=w802:T20)  [unwired: 9 in]
        n465 = call <vilib>:"Covariance Matrix.vi"("X"=w792) -> ("mean vector"=w779:dbl[], "covariance matrix V"=w797:T20)  [unwired: 9 in]
        n466 = Greater?(x=w771, y=0) -> (0:w769:bool)
        n467 = case shown="True" w769 {
          frame False {
          }
          frame True {
            n468 = One Button Dialog(message="MC run finished successfully") -> ()  [unwired: 1 in, 1 out]
          }
        }
        n469 = Index Array(array=w802) -> (element=w801:T20)  [unwired: 2 in]
        n470 = Index Array(array=w797) -> (element=w796:T20)  [unwired: 2 in]
        n471 = call-poly <vilib>:"Matrix To Array.vi"("Real Matrix"=w801) -> ("Real 2D Array"=w800:dbl[][])
        n472 = call-poly <vilib>:"Matrix To Array.vi"("Real Matrix"=w796) -> ("Real 2D Array"=w795:dbl[][])
        n473 = Index Array(array=w800, index (col)=0 ("disabled index (col)")) -> (element=w798:dbl[])  [unwired: 1 in]
        n474 = Index Array(array=w795, index (col)=0 ("disabled index (col)")) -> (element=w793:dbl[])  [unwired: 1 in]
        n475 = Bundle(w776, "mean vector"=w775) -> (w791:cluster{dbl[], "mean vector":dbl[]})  [unwired: 1 in]
        n476 = Square Root(x=w798) -> (sqrt(x)=w777:dbl[])
        n477 = Bundle(w776, "mean vector"=w779) -> (w788:cluster{dbl[], "mean vector":dbl[]})  [unwired: 1 in]
        n478 = Square Root(x=w793) -> (sqrt(x)=w778:dbl[])
        n479 = call "XY error bars.vi"("XY plot"=w791, "Yerror"=w777) -> ("Y error bars"=w790:cluster{dbl[], dbl[]})  [unwired: 6 in, 2 out]
        n480 = call "XY error bars.vi"("XY plot"=w788, "Yerror"=w778) -> ("Y error bars"=w787:cluster{dbl[], dbl[]})  [unwired: 6 in, 2 out]
        n481 = Bundle By Name(cluster=w783, "Real RI"=w775, "Imaginary RI"=w779, "Std Imaginary RI"=w778, "Std Real RI"=w777, "Wavelength"=w776) -> (w780:T13)
        n482 = Build Array(w791, w790) -> (→"Real Part MC":cluster{dbl[], "mean vector":dbl[]}[])
        n483 = Build Array(w788, w787) -> (→"Imaginary Part MC":cluster{dbl[], "mean vector":dbl[]}[])
        n484 = Bundle By Name(cluster=w782, "RI MC results"=w780) -> (w781:T14)
      }
      frame "Retreive RI from Single Measurements(MC)" {
        w888 = T13 {"Real RI"=[], "Imaginary RI"=[], "Std Imaginary RI"=[], "Std Real RI"=[], "Wavelength"=[], "Residue"=[], "Extinction Factor"=[], "Diameter Factor"=[], "Diameter Offset"=[], "Best fit result"=[], "Normalized Residuals"=[]}  # RI MC results
        n485 = call <vilib>:"Add State(s) to Queue__jki_lib_state_machine.vi"("State(s) in (\"\")"=w912) -> ("States Out"=w911:string)  [unwired: 14 in]
        n486 = property on="Min Wavelength" class="CmbBox"() -> ("Value"=w868:string)  [unwired: 2 in, 2 out]
        n487 = property on="Max Wavelength" class="CmbBox"() -> ("Value"=w867:string)  [unwired: 2 in, 2 out]
        n488 = Unbundle By Name(w887) -> ("Extinction ExtinctionUncertainity Size parameter and Number ofS sizes"=w906:T5, "Particle Distribution Data"=w909:T6, "FullExtinctionData"=w873:dbl[][], "NumberOfMeasurementsperSize"=w870:i32)
        n489 = Decimal String To Number(string=w868) -> (number=w865:i32)  [unwired: 2 in, 1 out]
        n490 = Decimal String To Number(string=w867) -> (number=w866:i32)  [unwired: 2 in, 1 out]
        n491 = local write "Size of statistics"(w870) -> ()
        n492 = local read "General Data for RI Retrieval VI"() -> (w861:T3)
        n493 = local read "Size Parameter Factor"() -> (w863:bool)
        n494 = local read "Size Parameter Offset"() -> (w862:bool)
        n495 = local read "Extinction Factor"() -> (w864:bool)
        n496 = Unbundle By Name(w906) -> ("Number ofSizes"=w908:dbl, "Extinction Uncertainty"=w907:dbl[][])
        n497 = Bundle(cluster=w861, "Min WaveLength Index"=w865, "Max WaveLength Index"=w866, "Extinction Factor"=w864, "Size Parameter Factor"=w863, "Size Paramter Offset"=w862) -> (w879:T3)  [unwired: 4 in]
        n498 = local read "Restrict to Positive Imaginary Part"() -> (w869:bool)
        n499 = local read "Size of statistics"() -> (w877:i32)
        n500 = control-ref of="MC progress"() -> (w878:refnum<vi>)
        n501 = Tick Count (ms)() -> (millisecond timer value=w889:u32)
        n502 = property class="Slide (strict)"(reference=w878, "Scale.Maximum"=w877) -> ()  [unwired: 1 in, 2 out]
        n503 = for {
          N: w870 -> [_]
          tunnel: w909 -> [w949]
          tunnel: w908 -> [w921]
          tunnel: w907 -> [_]
          tunnel: w906 -> [w946]
          tunnel: [w941] -> w905 mode=indexing
          tunnel: [w937] -> w894 mode=indexing
          tunnel: [w936] -> w881
          tunnel: w870 -> [w931]
          shift-right: [w929] -> _
          shift-left: w889 -> [w935]
          tunnel: w879 -> [w915]
          tunnel: w878 -> [w928]
          tunnel: [w927] -> w876
          tunnel: w873 -> [w922]
          tunnel: w870 -> [w917]
          tunnel: w869 -> [w916]
          i -> [w920]
          n504 = Tick Count (ms)() -> (millisecond timer value=w929:u32)
          n505 = Subtract(x=w929, y=w935) -> (x-y=w934:u32)
          n506 = Increment(x=w920) -> (x+1=w919:i32)
          n507 = Increment(x=w920) -> (x+1=w927:i32)
          n508 = mathscript code="Extinction=[];\nfor j=0:(NumOfSizes-1)\nExtinction=[Extinction FullExt(:,j*NumOfMeas+i)];\ntemp=j*NumOfMeas+i;\nend\n%Extinction=Extinction';"("FullExt"=w922, "i"=w919, "NumOfSizes"=w921, "NumOfMeas"=w917) -> ("Extinction"=w918:dbl[][])  [unwired: 1 in, 1 out]
          n509 = property class="Slide (strict)"(reference=w928, "Value"=w927) -> ()  [unwired: 1 in, 2 out]
          n510 = Divide(x=w934, y=u32 60000) -> (x/y=w932:dbl)
          n511 = Bundle By Name(cluster=w946, "Extinction"=w918) -> (w945:T5)
          n512 = Subtract(x=w931, y=w920) -> (x-y=w930:i32)
          n513 = control-ref of="Simplex"() -> (w914:refnum<vi>)
          n514 = Multiply(x=w932, y=w930) -> (x*y=w924:dbl)
          n515 = control-ref of="Real Part vs wavelength"() -> (w952:refnum<vi>)
          n516 = control-ref of="Not Corrected for Multiple charge Best fit result"() -> (w950:refnum<vi>)
          n517 = control-ref of="Imaginary Part vs wavelength"() -> (w951:refnum<vi>)
          n518 = control-ref of="Normalized Residuals vs Size parameter"() -> (w948:refnum<vi>)
          n519 = local write "Time Left (min) (MC)"(w924) -> ()
          n520 = local read "Minimization method"() -> (w926:u16)
          n521 = local read "Approximate Errors"() -> (w923:bool)
          n522 = local read "Calculate Errors"() -> (w925:bool)
          n523 = Bundle("Real Part vs wavelength"=w952, "Imaginary Part vs wavelength"=w951, "Normalized Residuals vs Size parameter"=w948, "Not Corrected for Multiple charge Best fit result"=w950, "Simplex"=w914) -> (w947:T19)  [unwired: 1 in]
          n524 = call "RIRetrieval.vi"("General Data for RI Retrieval VI"=w915, "Approximate Errors"=w923, "Restrict to Positive Imaginary Part"=w916, "Extinction Measured Data"=w945, "Calculate Errors"=w925, "Particle Distribution Data"=w949, "Graph Refs"=w947, "Minimization method"=w926) -> ("Imaginary Part vs wavelength"=w938:cluster{dbl[], dbl[]}[], "Real Part vs wavelength"=w944:cluster{dbl[], dbl[]}[])  [unwired: 2 out]
          n525 = Index Array(array=w944, index=0) -> (element=w942:cluster{dbl[], dbl[]})
          n526 = Index Array(array=w938, index=0) -> (element=w939:cluster{dbl[], dbl[]})
          n527 = Unbundle(w942) -> (w936:dbl[], w941:dbl[])
          n528 = Unbundle(w939) -> (w937:dbl[])  [unwired: 1 out]
          "Loop index (MC) 2" <- w920
        }
        n529 = call <vilib>:"Covariance Matrix.vi"("X"=w905) -> ("mean vector"=w880:dbl[], "covariance matrix V"=w904:T20)  [unwired: 9 in]
        n530 = call <vilib>:"Covariance Matrix.vi"("X"=w894) -> ("mean vector"=w884:dbl[], "covariance matrix V"=w899:T20)  [unwired: 9 in]
        n531 = Greater?(x=w876, y=0) -> (0:w874:bool)
        n532 = case shown="True" w874 {
          frame False {
          }
          frame True {
            n533 = One Button Dialog(message="MC run finished successfully") -> ()  [unwired: 1 in, 1 out]
          }
        }
        n534 = Index Array(array=w904) -> (element=w903:T20)  [unwired: 2 in]
        n535 = Index Array(array=w899) -> (element=w898:T20)  [unwired: 2 in]
        n536 = call-poly <vilib>:"Matrix To Array.vi"("Real Matrix"=w903) -> ("Real 2D Array"=w902:dbl[][])
        n537 = call-poly <vilib>:"Matrix To Array.vi"("Real Matrix"=w898) -> ("Real 2D Array"=w897:dbl[][])
        n538 = Index Array(array=w902, index (col)=0 ("disabled index (col)")) -> (element=w900:dbl[])  [unwired: 1 in]
        n539 = Index Array(array=w897, index (col)=0 ("disabled index (col)")) -> (element=w895:dbl[])  [unwired: 1 in]
        n540 = Bundle(w881, "mean vector"=w880) -> (w893:cluster{dbl[], "mean vector":dbl[]})  [unwired: 1 in]
        n541 = Square Root(x=w900) -> (sqrt(x)=w882:dbl[])
        n542 = Bundle(w881, "mean vector"=w884) -> (w891:cluster{dbl[], "mean vector":dbl[]})  [unwired: 1 in]
        n543 = Square Root(x=w895) -> (sqrt(x)=w883:dbl[])
        n544 = call "XY error bars.vi"("XY plot"=w893, "Yerror"=w882) -> ("Y error bars"=w892:cluster{dbl[], dbl[]})  [unwired: 6 in, 2 out]
        n545 = call "XY error bars.vi"("XY plot"=w891, "Yerror"=w883) -> ("Y error bars"=w890:cluster{dbl[], dbl[]})  [unwired: 6 in, 2 out]
        n546 = Bundle By Name(cluster=w888, "Real RI"=w880, "Imaginary RI"=w884, "Std Imaginary RI"=w883, "Std Real RI"=w882, "Wavelength"=w881) -> (w885:T13)
        n547 = Build Array(w893, w892) -> (w872:cluster{dbl[], "mean vector":dbl[]}[])
        n548 = Build Array(w891, w890) -> (w871:cluster{dbl[], "mean vector":dbl[]}[])
        n549 = local write "Real Part MC"(w872) -> ()
        n550 = local write "Imaginary Part MC"(w871) -> ()
        n551 = Bundle By Name(cluster=w887, "RI MC results"=w885) -> (w886:T14)
      }
      frame "Update Window after Load Files" {
        n552 = Unbundle By Name(w1061) -> ("Extinction ExtinctionUncertainity Size parameter and Number ofS sizes.WaveLength"=w1060:dbl[])
        n553 = call <vilib>:"Add State(s) to Queue__jki_lib_state_machine.vi"("State(s) in (\"\")"=w1064) -> ("States Out"=w1063:string)  [unwired: 14 in]
        n554 = for {
          tunnel: w1060 -> [w1076] mode=indexing
          tunnel: [w1077] -> w1059 mode=indexing
          tunnel: [w1075] -> w1058 mode=indexing
          i -> [w1075]
          n555 = Number To Decimal String(number=w1075) -> (decimal integer string=w1074:string)  [unwired: 1 in]
          n556 = Number To Fractional String(number=w1076, precision (6)=i16 3) -> (F-format string=w1073:string)  [unwired: 2 in]
          n557 = Bundle(w1073, w1074) -> (w1077:cluster{string, string})  [unwired: 1 in]
        }
        n558 = flat-sequence {
          tunnel: w1059 -> [w1066]
          tunnel: w1059 -> [w1065]
          tunnel: w1058 -> [w1071]
          frame #0 {
            n559 = property on="Max Wavelength" class="CmbBox"("Strings And Values[]"=w1066) -> ()  [unwired: 2 in, 2 out]
            n560 = property on="Min Wavelength" class="CmbBox"("Strings And Values[]"=w1065) -> ()  [unwired: 2 in, 2 out]
          }
          frame #1 {
            n561 = Array Max & Min(array=w1071) -> (max value=w1067:i32, min value=w1070:i32)  [unwired: 2 out]
            n562 = Number To Decimal String(number=w1067) -> (decimal integer string=w1069:string)  [unwired: 1 in]
            n563 = Number To Decimal String(number=w1070) -> (decimal integer string=w1068:string)  [unwired: 1 in]
            n564 = property on="Max Wavelength" class="CmbBox"("Value"=w1069) -> ()  [unwired: 2 in, 2 out]
            n565 = property on="Min Wavelength" class="CmbBox"("Value"=w1068) -> ()  [unwired: 2 in, 2 out]
          }
        }
      }
      frame "Update Corrected multiple charge extinction graph" {
        w1081 = i16 3 ("precision (6)")
        n566 = call <vilib>:"Add State(s) to Queue__jki_lib_state_machine.vi"("State(s) in (\"\")"=w1142) -> ("States Out"=w1141:string)  [unwired: 14 in]
        n567 = control-ref of="Imaginary Part vs wavelength"() -> (w1137:refnum<vi>)
        n568 = Unbundle By Name(w1100) -> ("Baes data type definition"=w1122:T8, "Extinction ExtinctionUncertainity Size parameter and Number ofS sizes.WaveLength"=w1136:dbl[], "Extinction ExtinctionUncertainity Size parameter and Number ofS sizes.Extinction"=w1125:dbl[][], "Extinction ExtinctionUncertainity Size parameter and Number ofS sizes.Extinction Uncertainty"=w1126:dbl[][], "Extinction ExtinctionUncertainity Size parameter and Number ofS sizes.Size parameters"=w1128:dbl[][], "Extinction ExtinctionUncertainity Size parameter and Number ofS sizes.Number ofSizes"=w1129:dbl, "Extinction ExtinctionUncertainity Size parameter and Number ofS sizes.GeometricCrossSection"=w1130:dbl[], "Extinction ExtinctionUncertainity Size parameter and Number ofS sizes.WaveLength"=w1132:dbl[], "Particle Distribution Data.SMPS Sizes"=w1133:dbl[], "Particle Distribution Data.Concentration"=w1134:dbl[][], "Particle Distribution Data.Double Charge Correction Flag"=w1135:bool, "RI results.Extinction Factor"=w1118:dbl[], "RI results.Diameter Factor"=w1114:dbl[], "RI results.Diameter Offset"=w1113:dbl[], "RI results.Residue"=w1116:dbl[], "RI results.Real RI"=w1109:dbl[], "RI results.Std Real RI"=w1108:dbl[], "RI results.Imaginary RI"=w1107:dbl[], "RI results.Std Imaginary RI"=w1106:dbl[], "RI results.Best fit result"=w1105:dbl[][], "RI results.Normalized Residuals"=w1104:dbl[][])  [unwired: 1 out]
        n569 = property on="Property Node" class="XYGraph (strict)"(reference=w1137) -> ("Cursor.Cursor X"=w1080:dbl)  [unwired: 1 in, 2 out]
        "Wavelength" <- w1080
        n570 = Search 1D Array(1D array=w1136, element=w1080) -> (index of element=w1103:i32)  [unwired: 1 in]
        "index of element" <- w1103
        n571 = Index Array(array=w1132, index=w1103) -> (element=w1131:dbl)
        n572 = Index Array(array=w1116, index=w1103) -> (element=→"Residue (MDBF)":dbl)
        n573 = Index Array(array=w1125, index (row)=w1103) -> (element=w1124:dbl[])  [unwired: 1 in]
        n574 = Index Array(array=w1126, index (row)=w1103) -> (element=w1123:dbl[])  [unwired: 1 in]
        n575 = Index Array(array=w1128, index (row)=w1103) -> (element=w1127:dbl[])  [unwired: 1 in]
        n576 = Index Array(array=w1118, index=w1103) -> (element=w1115:dbl)
        "Extinction Factor" <- w1115
        n577 = Index Array(array=w1114, index=w1103) -> (element=w1111:dbl)
        "Diameter Factor" <- w1111
        n578 = Index Array(array=w1113, index=w1103) -> (element=w1110:dbl)
        "Diameter Offset" <- w1110
        n579 = Index Array(array=w1109, index=w1103) -> (element=w1097:dbl)
        "Real part" <- w1097
        n580 = Index Array(array=w1108, index=w1103) -> (element=w1096:dbl)
        "Real Uncertainty" <- w1096
        n581 = Index Array(array=w1106, index=w1103) -> (element=w1084:dbl)
        "Imaginary Uncertainty" <- w1084
        n582 = Index Array(array=w1107, index=w1103) -> (element=w1085:dbl)
        "Imaginary Part" <- w1085
        n583 = Index Array(array=w1105, index (row)=w1103) -> (element=w1102:dbl[])  [unwired: 1 in]
        n584 = Index Array(array=w1104, index (row)=w1103) -> (element=w1101:dbl[])  [unwired: 1 in]
        n585 = Less Than 0?(x=w1103) -> (x < 0?=w1119:bool)
        n586 = Number To Fractional String(number=w1097, precision (6)=w1081) -> (F-format string=w1095:string)  [unwired: 2 in]
        n587 = Number To Fractional String(number=w1080, precision (6)=w1081) -> (F-format string=w1079:string)  [unwired: 2 in]
        n588 = Number To Fractional String(number=w1096, precision (6)=w1081) -> (F-format string=w1093:string)  [unwired: 2 in]
        n589 = Number To Fractional String(number=w1085, precision (6)=w1081) -> (F-format string=w1090:string)  [unwired: 2 in]
        n590 = Number To Fractional String(number=w1084, precision (6)=w1081) -> (F-format string=w1088:string)  [unwired: 2 in]
        n591 = Concatenate Strings("WL=" ("string"), w1079, "nm" ("string")) -> (→"Wavelength":string)
        n592 = Concatenate Strings("n=" ("string"), w1095, "±" ("element"), w1093) -> (→"Real Part":string)
        n593 = Concatenate Strings("k=" ("string"), w1090, "±" ("element"), w1088) -> (→"Imaginary Part":string)
        n594 = Bundle By Name(cluster=w1122, "Extinction"=w1124, "Extinction Uncertainty"=w1123, "Size parameters"=w1127, "Number ofSizes"=w1129, "GeometricCrossSection"=w1130, "Wave Length"=w1131, "SMPS Sizes"=w1133, "Concentration"=w1134, "Double Charge Correction"=w1135, "Extincation Factor"=w1115) -> (w1098:T8)
        n595 = in-place {
          in-place-border: w1111 -> [w1150]
          in-place-border: w1110 -> [w1148]
          n596 = in-place-cluster #1(w1098) -> ("Size parameters"=w1154:dbl[], "Wave Length"=w1144:dbl)
          n597 = Multiply(x=w1154, y=w1144) -> (x*y=w1153:dbl[])
          n598 = Divide(x=w1153, y=3.141592653589793) -> (x/y=w1151:dbl[])
          n599 = Multiply(x=w1151, y=w1150) -> (x*y=w1149:dbl[])
          n600 = Add(x=w1149, y=w1148) -> (x+y=w1147:dbl[])
          n601 = Multiply(x=w1147, y=3.141592653589793) -> (x*y=w1145:dbl[])
          n602 = Divide(x=w1145, y=w1144) -> (x/y=w1143:dbl[])
          n603 = in-place-cluster #1("Size parameters"=w1143, "Wave Length"=w1144) -> (w1112:T8)
        }
        n604 = Bundle By Name(cluster=w1100, "Baes data type definition"=w1098) -> (w1099:T14)
        n605 = control-ref of="Real Part vs wavelength"() -> (w1139:refnum<vi>)
        n606 = control-ref of="Imaginary Part vs wavelength"() -> (w1138:refnum<vi>)
        n607 = property on="Property Node" class="XYGraph (strict)"(reference=w1139) -> ("Cursor.Cursor Y"=w1121:dbl)  [unwired: 1 in, 2 out]
        n608 = property on="Property Node" class="XYGraph (strict)"(reference=w1138) -> ("Cursor.Cursor Y"=w1120:dbl)  [unwired: 1 in, 2 out]
        n609 = case shown="False" w1119 {
          tunnel: w1112 -> [w1172 _]
          tunnel: w1121 -> [w1168 _]
          tunnel: w1120 -> [w1167 _]
          tunnel: w1098 -> [w1169 _]
          tunnel: w1102 -> [w1182 _]
          tunnel: w1101 -> [w1178 _]
          frame False {
            # "Calculate Residue (CDMRI)"
            # "Update Measured graph as well"
            n610 = call "CalculateExpectedExtinctionIncludingDoublyChargeParticleCorrection.vi"("refractive index, imaginary"=w1167, "refractive index, real"=w1168, "Extinction ExtinctionUncertainity Size parameter and Number ofS sizes"=w1169) -> ("Expected Extinction Cross Section"=w1166:sgl[])  [unwired: 1 out]
            n611 = call "CalculateExtinctionCorrectionsToDoublyChargeParticleContribution.vi"("refractive index, imaginary"=w1167, "refractive index, real"=w1168, "Extinction ExtinctionUncertainity Size parameter and Number ofS sizes"=w1169) -> ("Expected Extinction graph"=→"Multiple charge correction term":cluster{"Size parameters":dbl[], dbl[]}, "Expected Extinction Cross Section"=w1165:sgl[])
            n612 = Subtract(x=w1166, y=w1165) -> (x-y=w1162:sgl[])
            n613 = Unbundle By Name(w1172) -> ("Extinction"=w1176:dbl[], "Size parameters"=w1164:dbl[], "Extinction Uncertainty"=w1159:dbl[], "Number ofSizes"=w1156:dbl)
            n614 = Subtract(x=w1176, y=w1165) -> (x-y=w1171:dbl[])
            n615 = call "CalculateAreaOfFirstPeakofSizeDistribution.vi"("Extinction ExtinctionUncertainity Size parameter and Number ofS sizes"=w1172) -> ("Area of First peak"=w1161:dbl[])
            n616 = Bundle("Size parameters"=w1164, "Extinction"=w1176) -> (w1192:T21)  [unwired: 1 in]
            n617 = Bundle("Size parameters"=w1164, "Extinction"=w1176) -> (w1184:T21)  [unwired: 1 in]
            n618 = Bundle("Size parameters"=w1164, "Normalized Residuals"=w1178) -> (w1180:T22)  [unwired: 1 in]
            n619 = Divide(x=w1162, y=w1161) -> (x/y=w1160:dbl[])
            n620 = Divide(x=w1171, y=w1161) -> (x/y=w1170:dbl[])
            n621 = call "PlotMieCurve.vi"("refractive index, imaginary"=w1167, "refractive index, real"=w1168, "Use Extinction Factor"=TRUE, "Extinction ExtinctionUncertainity Size parameter and Number ofS sizes"=w1172) -> ("Mie Results In Size Parameters"=w1177:sgl[], "Size parameters"=w1189:dbl[], "Extinction Crosssections"=w1190:dbl[])
            n622 = Bundle("Size parameters"=w1164, "Best fit result"=w1182) -> (w1181:T23)  [unwired: 1 in]
            n623 = Build Array(w1180) -> (w1179:T2)
            n624 = call "XY error bars.vi"("XY plot"=w1184, "Yerror"=w1159) -> ("Y error bars"=w1183:cluster{dbl[], dbl[]})  [unwired: 6 in, 2 out]
            n625 = Subtract(x=w1177, y=w1170) -> (x-y=w1175:dbl[])
            n626 = Bundle("Size parameters"=w1164, w1170) -> (w1187:cluster{"Size parameters":dbl[], dbl[]})  [unwired: 1 in]
            n627 = Build Array(w1184, w1183, w1181) -> (w1185:T24)
            n628 = property on="Normalized Residuals vs Size parameter" class="XYGraph (strict)"("Value"=w1179) -> ()  [unwired: 2 in, 2 out]
            n629 = Bundle("Size parameters"=w1164, w1160) -> (w1163:cluster{"Size parameters":dbl[], dbl[]})  [unwired: 1 in]
            n630 = Bundle("Size parameters"=w1189, "Extinction Crosssections"=w1190) -> (w1188:T17)  [unwired: 1 in]
            n631 = property on="Not Corrected for Multiple charge Best fit result" class="XYGraph (strict)"("Value"=w1185) -> ()  [unwired: 2 in, 2 out]
            n632 = call "XY error bars.vi"("XY plot"=w1187, "Yerror"=w1159) -> ("Y error bars"=w1186:cluster{dbl[], dbl[]})  [unwired: 6 in, 2 out]
            n633 = Build Array(w1187, w1192, w1188, w1186, w1163) -> (→"Corrected for multiple charge particles":T18)
            n634 = Divide(x=w1175, y=w1159) -> (x/y=w1174:dbl[])
            n635 = Square(x=w1174) -> (x^2=w1158:dbl[])
            n636 = Add Array Elements(numeric array=w1158) -> (sum=w1157:dbl)
            n637 = Divide(x=w1157, y=w1156) -> (x/y=→"Residue (CDMRI)":dbl)
          }
          frame True {
          }
        }
      }
    }
  }
